vi "Position_TOTAL_R16.vi"(5 "Distance Between \nCameras  (*unit)":sgl=2.1) -> (0 "Valid Beacon Sets":bool[](array[boolean])=[FALSE, TRUE, TRUE, TRUE, FALSE], 12 "dX, dY\nLeft Cam":cluster{"X":sgl[], "Y":sgl[]}={"X"=[0.0, 0.30756128, 1.4106799, 2.4344175, 0.0], "Y"=[0.0, 5.248752, 5.2487316, 5.2487082, 0.0]}, 13 "Position Valid":bool=TRUE, 14 "Left Camera Real Coordinates":cluster{"X":sgl, "Y":sgl}={"X"=5.2487307, "Y"=1.1157805}, 16 "dX, dY\nRight Cam":cluster{"X":sgl[], "Y":sgl[]}={"X"=[-2.0986407, -1.7910794, -0.6879608, 0.3357769, -2.0986407], "Y"=[-0.07554352, 5.1732087, 5.1731877, 5.173165, -0.07554352]}, 17 "Distance to Each Beacon":cluster{" Right Cam":sgl[], " Left Cam":sgl[]}={" Right Cam"=[1.0, 5.491617, 5.181491, 5.20346, 1.0], " Left Cam"=[1.0, 5.2758446, 5.3987226, 5.8034377, 1.0]}, 18 "Robot Coordinates":cluster{"X":sgl, "Y":sgl}={"X"=5.210959, "Y"=2.1651008}, 19 "Orietnation\n(current)":sgl=-2.0627356 format="%#_13g")   [LabVIEW 2015]
uses:
  <vilib>/Analysis/NI_AALPro.lvlib
  <vilib>/myRIO/Instrument Drivers/Onboard IO/DIO/DIO.lvlib
  <vilib>/Instr/_visa.llb/VISA Configure Serial Port (Instr).vi
  <vilib>/Analysis/coordinate.llb/2D Cartesian Coordinate Rotation (Array).vi
panel:
  out "Current Recovery State -L":enum16{"Generic Sweep", "Recovery Search"}(ring)=enum."Recovery Search"
  out "Current Move Delta - L 2":u16
  out "Next Recovery State - Left":enum16{"Generic Sweep", "Recovery Search"}(ring)=enum."Recovery Search"
  out "Next Recovery State - Right":enum16{"Generic Sweep", "Recovery Search"}(ring)=enum."Recovery Search"
  out "Current Recovery State - Right":enum16{"Generic Sweep", "Recovery Search"}(ring)=enum."Recovery Search"
  in  "Initial Recovery State  - Right":enum16{"Generic Sweep", "Recovery Search"}(ring)=enum."Recovery Search"
  in  "Initial Recovery State - L":enum16{"Generic Sweep", "Recovery Search"}(ring)=enum."Recovery Search"
  out "Next Tracking State - Right":enum16{"Track", "Reactive Predict", ""}(ring)
  out "Current Tracking State - Right 2":enum16{"Track", "Reactive Predict", ""}(ring)
  in  "Initial Tracking State - Right":enum16{"Track", "Reactive Predict", ""}(ring)
  out "Last Track Angle - R":sgl=95.68359
  out "Next Tracking State - Left":enum16{"Track", "Reactive Predict", ""}(ring)
  in  "Initial Tracking State - Left":enum16{"Track", "Reactive Predict", ""}(ring)
  out "Current Tracking State - Left":enum16{"Track", "Reactive Predict", ""}(ring)
  in  "Timeout to \nEnable Reactive Predict":u16=10
  out "Tracking Timeout\nCount - R":i32
  in  "Tracking Timeout\nThreshold":i32=10
  out "Tracking Timeout\nCount - L":i32
  in  "Search Direction - in - Right":bool=TRUE
  out "Next Main State - Right":T1(ring)=enum."Tracking"
  in  "Recovery Search\nDirection - R":bool
  out "Recovery Mode Count in Right":i32
  out "Wait Tick Count - Right":i32
  out "Frames Processed\nCount - in Right":i32
  out "Recovery Search\nmove Count - Right":u16
  out "Recovery Search\nAttempt Count - Right":u16
  in  "Mounting Offset - Right":sgl=45.0
  in  "Tracking Angle - Right":sgl=95.568306
  in  "Current Servo Position\n- Right":u16
  out "New Data  Flag\nRight Servo":bool
  in  "Track Angle Valid  - R":bool=TRUE
  out "Current Main State - Right":T1(ring)=enum."Tracking"
  in  "Initial Main State- Right":T1(ring)
  in  "Recovery Search\nDirection - L 2":bool
  in  "Max Recovery Count\n(Recovery Search) 2":u16
  in  "Max Recovery\nSearch Attempts 2":u16
  in  "Image Lock - Right 2":bool
  out "Last Track Angle - L":sgl=73.76953
  in  "Recovery Search\nDirection - L":bool=TRUE
  out "Next Main State - Left":T1(ring)=enum."Tracking"
  out "Current Move Delta - L":u16
  in  "Max Recovery Count\n(Recovery Search)":u16=10
  in  "Max Recovery\nSearch Attempts":u16=3
  out "Recovery Search\nAttempt Count - in - L":u16
  out "Recovery Search\nmove Count - in - L":u16
  in  "Image Lock - Right":bool=TRUE
  out "Recovery Mode Count - in Left":u16
  in  "Middle Beacon\nCoordinates":cluster{"X":sgl, "Y":sgl}={"X"=0.0, "Y"=2.5}
  in  "Min Num Frames\nper Search":i32=3
  in  "Wait Tick Threshold":i32=10
  out "Wait Tick Count - in - L":i32
  out "Frames Processed\nCount - in -L":i32
  in  "Maximum Move \nServo Threshold":i16=300
  in  "Minimum Delta \nServo Threshold":i16=3
  in  "Mounting Offset - Left":sgl=-45.0
  in  "Search Step Size":u16=50
  in  "Search Direction - in - L":bool
  in  "Current Servo Position\n- Left":u16
  in  "Tracking Angle - Left":sgl=72.73481
  out "New Data  Flag\nLeft Servo":bool
  in  "Track Angle Valid - Left":bool=TRUE
  in  "Image Lock - Left":bool=TRUE
  in  "Initial Main State - Left":T1(ring)
  out "Current Main State - Left":T1(ring)=enum."Tracking"
  in  "Position Calc\nTimer":u32=100 caption="Position Calc Timer"
  in  "Fetch Input\n(mSec)":u32=20 caption="Update Camera Input\n(mSec)"
  out "Right Data\nInput Flag\n- Internal":bool
  in  "Position Calc\nReady":bool
  out "This Servo \nAngle - Right":sgl=95.09766
  in  "Beacon Angles -R":sgl[](array[numeric])=[117.22456, 106.97358, 95.568306, 84.2386, 100.09766]
  in  "Beacon Angles - L":sgl[](array[numeric])=[77.890625, 77.890625, 72.73481, 63.190956, 54.217514]
  in  "Valid Angles -R":bool[](array[boolean])=[TRUE, TRUE, TRUE, TRUE, FALSE]
  in  "Valid Angles - L":bool[](array[boolean])=[FALSE, FALSE, TRUE, TRUE, TRUE]
  out "Left Data\nInput Flag\n- Internal":bool=TRUE
  in  "Check Shared Var Timer":u32=50 caption="Main Loop\n Timer (ms)"
  out "Left_Flag 2":bool
  out "Right_Flag 2":bool
  out "Beacons Found\n- Left (Bool Array) 2":bool[](array[boolean])=[FALSE, FALSE, TRUE, TRUE, TRUE]
  out "LEFT Beacon Coord - X px (IN) 2":sgl[](array[numeric])=[0.0, 0.0, 159.73276, 214.00955, 263.49582]
  out "LEFT Beacon Position - Y px (IN) 2":sgl[](array[numeric])=[0.0, 0.0, 153.01732, 149.7353, 148.18039]
  out "This Servo \nAngle - Left":sgl=72.890625
  in  "Compliance Slope":u8=128
  out "deltaMoveServo\n- R":i16
  out "Move Respond - R":bool
  out "Move Respond - L":bool
  out "Last Position":cluster{"X":sgl, "Y":sgl}={"X"=5.210741, "Y"=2.1662946}
  out "Last Orientation":sgl=-2.061552
  in  "Distance\nBetween Beacons \n- Tolerance":sgl=0.35 format="%#_13g"
  in  "Distance\nBetween Beacons":sgl=1.0 format="%#_13g"
  out "atan2(y,x)":sgl=-2.481407
  out "dT":dbl=106.005
  in  "Orientation (-2) \nWeight":sgl=0.083333336 format="%#_13g"
  in  "Orientation (-1) \nWeight":sgl=0.16666667 format="%#_13g"
  in  "New Orientation \nThreshold":sgl=10.0
  out "Position Valid\nHistory":bool[](array[boolean])=[TRUE, FALSE, TRUE, TRUE, FALSE, TRUE, TRUE, FALSE, FALSE, FALSE, FALSE, FALSE, FALSE, FALSE, FALSE]
  out "Orientation\nHistory":sgl[](array[numeric])=[-2.061552, 0.0, -2.0449653, -2.0840735, 0.0, -2.086157, -2.0841389, 0.0, 0.0, 0.0, 0.0, 0.0, 0.0, 0.0, 0.0]
  out "Robot Coordinates\nHistory":cluster{sgl, sgl}[](array[cluster])=[{5.210741, 2.1662946}, {0.0, 0.0}, {5.209907, 2.1666946}, {5.2114477, 2.168679}, {0.0, 0.0}, {5.2056046, 2.1693063}, {5.2068563, 2.1687796}, {0.0, 0.0}, {0.0, 0.0}, {0.0, 0.0}, {0.0, 0.0}, {0.0, 0.0}, {0.0, 0.0}, {0.0, 0.0}, {0.0, 0.0}]
  in  "New Position \nThreshold":sgl=0.2
  in  "position(-2) weight":sgl=0.2 format="%#_13g"
  in  "position(-1) weight":sgl=0.3 format="%#_13g"
  out "Orientation Avgd":sgl=-2.061552
  in  "History Size":u8=15
  in  "Max Y (arena)":sgl=15.0
  in  "Max X (arena)":sgl=35.0
  in  "New Position\nWeight":sgl=0.5 format="%#_13g"
  in  "New Orientation\nWeight":sgl=0.75 format="%#_13g"
  in  "Max Std Dev (3)":sgl=0.2 format="%#_13g"
  in  "Max Std Dev (4)":sgl=0.2 format="%#_13g"
  out "Post Filtering\n- Valid Beacons":bool[](array[boolean])=[FALSE, TRUE, TRUE, TRUE, FALSE]
  in  "New Pos\nThreshold (*unit)\nfilterd UNUSED":sgl=0.2
  out "Robot Coordinates - Avgd":cluster{"X":sgl, "Y":sgl}={"X"=5.210741, "Y"=2.1662946}
  out "Real Position in Course 2":cluster{"X":dbl[], "Y":dbl[]}(graph)={"X"=[5.210741279561325], "Y"=[2.1662946728829504]}
  out "Position \nLock Status":bool=TRUE
  out "Right Camera Real Coordinate":cluster{"X":sgl, "Y":sgl}={"X"=5.1731873, "Y"=3.214421}
  out "deltaMoveServo\n- L":i16
  in  "Search Step Size\n(deg)":sgl=15.0 format="%#_13g"
  out "Beacons Found\n- Right (Bool Array)":bool[](array[boolean])=[TRUE, TRUE, TRUE, TRUE, FALSE]
  out "RIGHT Beacon Position - Y px (IN)":sgl[](array[numeric])=[160.86406, 153.76714, 154.61392, 152.4888, 0.0]
  out "RIGHT Beacon Coord - X px (IN)":sgl[](array[numeric])=[38.476494, 94.79557, 157.79951, 220.26955, 0.0]
  in  "Right Servo\nID":string="\u0001"
  in  "Servo Comm\nWait Time - (ms)":i32=1
  in  "Left Servo\nID":string="\u0000"
  out "dT - Comm Loop":u32=18
  in  "Servo Comm\nLoop Time (ms)":i32=10
  in  "close comms":bool
  in  "Max Read\nTx Attempts":u8=3
  in  "Max Write\nTx Attempts":u8=3
  out "Current R (10bit)":u16=683
  out "Servo Moving - R":bool
  out "Servo Moving - L":bool
  out "Current L (10bit)":u16=300
  in  "SERVO ENABLE":bool=TRUE
  out "Move Servo - L":bool
  out "Move Servo - R":bool
  in  "Servo Goal Position\n - Right":u16=685
  in  "Move Servo\nThreshold (deg)":sgl=2.0 format="%#_13g"
  in  "Servo Algorithm\nCycle Time(ms)":i32=50
  in  "Servo Goal Position\n - Left":u16=300
  in  "Current Angle\n - Left (internal)":sgl=72.890625
  in  "Current Angle\n - Right (internal)":sgl=95.09766
  in  "stop":bool
  in  "Num of Beacons (Total)":i8=5
  out "Angle to Pixel Ratios":T2={"Angle to Pixel\nRatio - Horizontal"=0.18125, "Angle to Pixel\nRatio - Vertical"=0.1875} {"Angle to Pixel\nRatio - Vertical" format="%#_13g"; "Angle to Pixel\nRatio - Horizontal" format="%#_13g"}
  in  "Cam AOV Vertical (deg)":sgl=45.0
  in  "Cam AOV Horizontal (deg)":sgl=58.0
  in  "Image Height (px)":sgl=240.0
  in  "Image Width (px)":sgl=320.0
  out "Beacon Coordinates - Left Image":T3={"Beacon Position - X px"=[0.0, 0.0, 159.73276, 214.00955, 263.49582], "Beacon Position - Y px"=[0.0, 0.0, 153.01732, 149.7353, 148.18039]}
  out "Beacon Coordinates - Right Image":T3={"Beacon Position - X px"=[38.476494, 94.79557, 157.79951, 220.26955, 0.0], "Beacon Position - Y px"=[160.86406, 153.76714, 154.61392, 152.4888, 0.0]}
  out "Distance to LBF":sgl[](array[numeric])=[0.024284193, 0.015691843, 0.008273765, 0.028971607, 0.03291407]
  out "Local Coordinates - Calculated":cluster{sgl[], sgl[]}(graph)={[0.0, 0.49682832, 1.5972277, 2.6223545, 0.0], [0.0, 5.2523994, 5.1570406, 5.1771755, 0.0]}
  out "Local Coordinates - Adjusted":cluster{sgl[], sgl[]}(graph)={[0.0, 0.49617612, 1.59858, 2.6216543, 0.0], [0.0, 5.234291, 5.1945877, 5.1577377, 0.0]}
  out "Normalized Beacons\nCoordinates Relative\nto Robot\n- Local":cluster{"X":sgl[], "Y":sgl[]}={"X"=[0.0, 0.49617612, 1.59858, 2.6216543, 0.0], "Y"=[0.0, 5.234291, 5.1945877, 5.1577377, 0.0]}
  out "Local Coordinates - Rotated":cluster{dbl[], dbl[]}(graph)={[2.0986406972551275, 0.0, 0.30756127015511747, 1.410679881134365, 2.4344175822405747, 0.0], [0.07554351912182478, 0.0, 5.248752221809901, 5.248731441918036, 5.24870847628271, 0.0]}
  out "All Object Coordinates \n- Local - Rotated":cluster{"X":sgl[], "Y":sgl[]}={"X"=[2.0986407, 0.0, 0.30756128, 1.4106799, 2.4344175, 0.0], "Y"=[0.07554352, 0.0, 5.248752, 5.2487316, 5.2487082, 0.0]}
  out "Local Coordinates - Normalized":cluster{sgl[], dbl[]}(graph)={[2.1, 0.0, 0.49617612, 1.59858, 2.6216543, 0.0], [0.0, 0.0, 5.234291076660156, 5.194587707519531, 5.157737731933594, 0.0]}
  in  "Max Std Dev (5)":sgl=0.2 format="%#_13g"
  out "All Object Coordinates \n- Local":cluster{"X":sgl[], "Y":sgl[]}={"X"=[2.1, 0.0, 0.49617612, 1.59858, 2.6216543, 0.0], "Y"=[0.0, 0.0, 5.234291, 5.1945877, 5.1577377, 0.0]}
  out "LOCAL\nBeacon Coordinates\nRelative to Robot":cluster{"dX_beacon":sgl[], "dY_beacon":sgl[]}={"dX_beacon"=[0.0, 0.49682832, 1.5972277, 2.6223545, 0.0], "dY_beacon"=[0.0, 5.2523994, 5.1570406, 5.1771755, 0.0]}
  out "dA2":sgl=26.863228 format="%#_13g"
  out "All Same\nDirection":bool=TRUE
  out "Valid Data\nSets":bool[](array[boolean])=[FALSE, TRUE, TRUE, TRUE, FALSE]
  in  "Distance Threshold\nRef Triangles (*unit)":sgl=20.0
  in  "Real Beacon\n - Coordinates":cluster{"X":dbl[], "Y":dbl[]}={"X"=[0.0, 0.0, 0.0, 0.0, 0.0, 0.0], "Y"=[0.5, 1.5, 2.5, 3.5, 4.5, 0.0]}
  # "POSITION CALCULATION VARIABLES"
  # "OUTPUT VALUES"
  # "CONFIG VALUES"
  # "FILTER CONFIG VALUES"
  # "FEEDBACK INPUT VALUES"
  # "INPUT VALUES"
  # "INTERMEDIATE VALUES"
  # "IMAGE TO ANGLE VARIABLES"
  # "VISION PROCESSEING INPUTS"
  # "Use moving average for previous orientation thresholds"
  # "INPUTS"
  # "CONFIG"
  # "OUTPUT VALUES"
  # "*********************"
  # "unfiltered"
  # "NEW FILTER VALS"
  # "Inter Beacon Distance Filtering"
  # "SERVO CONTROL VARIABLES"
  # "SERVO CONTROL VARIABLES"
  # "CONFIG"
  # "SHARED VARIABLE INPUTS"
  # "LOCAL VARIABLE INPUTS"
  # "INTERNRAL VARIABLES"
  # "SEARCH ROUTINE VARIABLES"
  # "MISC"
  # "SERVO IDs"
  # "CONTROL DELAYS"
  # "COMM LOOP DELAY"
  # "COMM PROTOCOL"
  # "SETTINGS"
  # "Make function of distance^^"
  # "**** only left side starts search\nat previously known good angle"
  # "LEFT SERVO"
  # "RIGHT SERVO"
  # "Main State Machine"
  # "Recovery State Machine"
  # "Current Track Angle Inputs"
  # "Servo Status Inputs"
  # "Main State Machine Inputs"
  # "Recovery State Machine Inputs"
  # "Current Track Angle Inputs"
  # "Servo Status Inputs"
  # "Recovery State Machine Feedback"
  # "Tracking State Machine Inputs"
  # "Tracking State Machine Inputs"
  # "NOTE: Must be 1 bigger than amount of beacons"
  # "NOTE: Must be 1 bigger than amount of beacons"
types:
  T1 = enum16{"Start Up Search", "Tracking", "Recovery Mode", ""}
  T2 = cluster{"Angle to Pixel\nRatio - Horizontal":sgl, "Angle to Pixel\nRatio - Vertical":sgl}
  T3 = cluster{"Beacon Position - X px":sgl[], "Beacon Position - Y px":sgl[]}
  T4 = cluster{"Array of Double":dbl[], "Array of Double":dbl[]}
  T5 = typedef "DIO.lvlib/DIO Reference.ctl" = cluster{"myRIO Reference":T6, "DIO Channels List":T10}
  T6 = typedef "myRIO Generic Hardware Reference.ctl" = cluster{"myRIO Model":T7, "myRIO Hardware Reference":T8}
  T7 = typedef "Hardware Version Enum.ctl" = enum16{"Unknown", "myRIO-1900", "myRIO-1950", "roboRIO"}
  T8 = typedef "myRIO v1.0 Reference.ctl" = cluster{"Generic FPGA Reference":T9, "Allow multiple opens":bool}
  T9 = typedef "Generic FPGA Reference.ctl" = refnum<k20>
  T10 = typedef "DIO Channels List.ctl" = T11[]
  T11 = typedef "DIO Channels Enum.ctl" = enum16{"Not Connected", "C/DIO0", "C/DIO1", "C/DIO2", "C/DIO3", "C/DIO4", "C/DIO5", "C/DIO6", "C/DIO7", "A/DIO0", "A/DIO1", "A/DIO2", "A/DIO3", "A/DIO4", "A/DIO5", "A/DIO6", "A/DIO7", "A/DIO8", "A/DIO9", "A/DIO10", "A/DIO11", "A/DIO12", "A/DIO13", "A/DIO14", "A/DIO15", "B/DIO0", "B/DIO1", "B/DIO2", "B/DIO3", "B/DIO4", "B/DIO5", "B/DIO6", "B/DIO7", "B/DIO8", "B/DIO9", "B/DIO10", "B/DIO11", "B/DIO12", "B/DIO13", "B/DIO14", "B/DIO15", "LED0", "LED1", "LED2", "LED3", "Button0", "DIO/DIO0", "DIO/DIO1", "DIO/DIO2", "DIO/DIO3", "DIO/DIO4", "DIO/DIO5", "DIO/DIO6", "DIO/DIO7", "DIO/DIO8", "DIO/DIO9", "SPI/CS0", "SPI/CS1", "SPI/CS2", "SPI/CS3", "LED RADIO (Green)", "LED RADIO (Red)", "LED COMM (Green)", "LED COMM (Red)", "LED MODE (Green)", "LED MODE (Red)"}
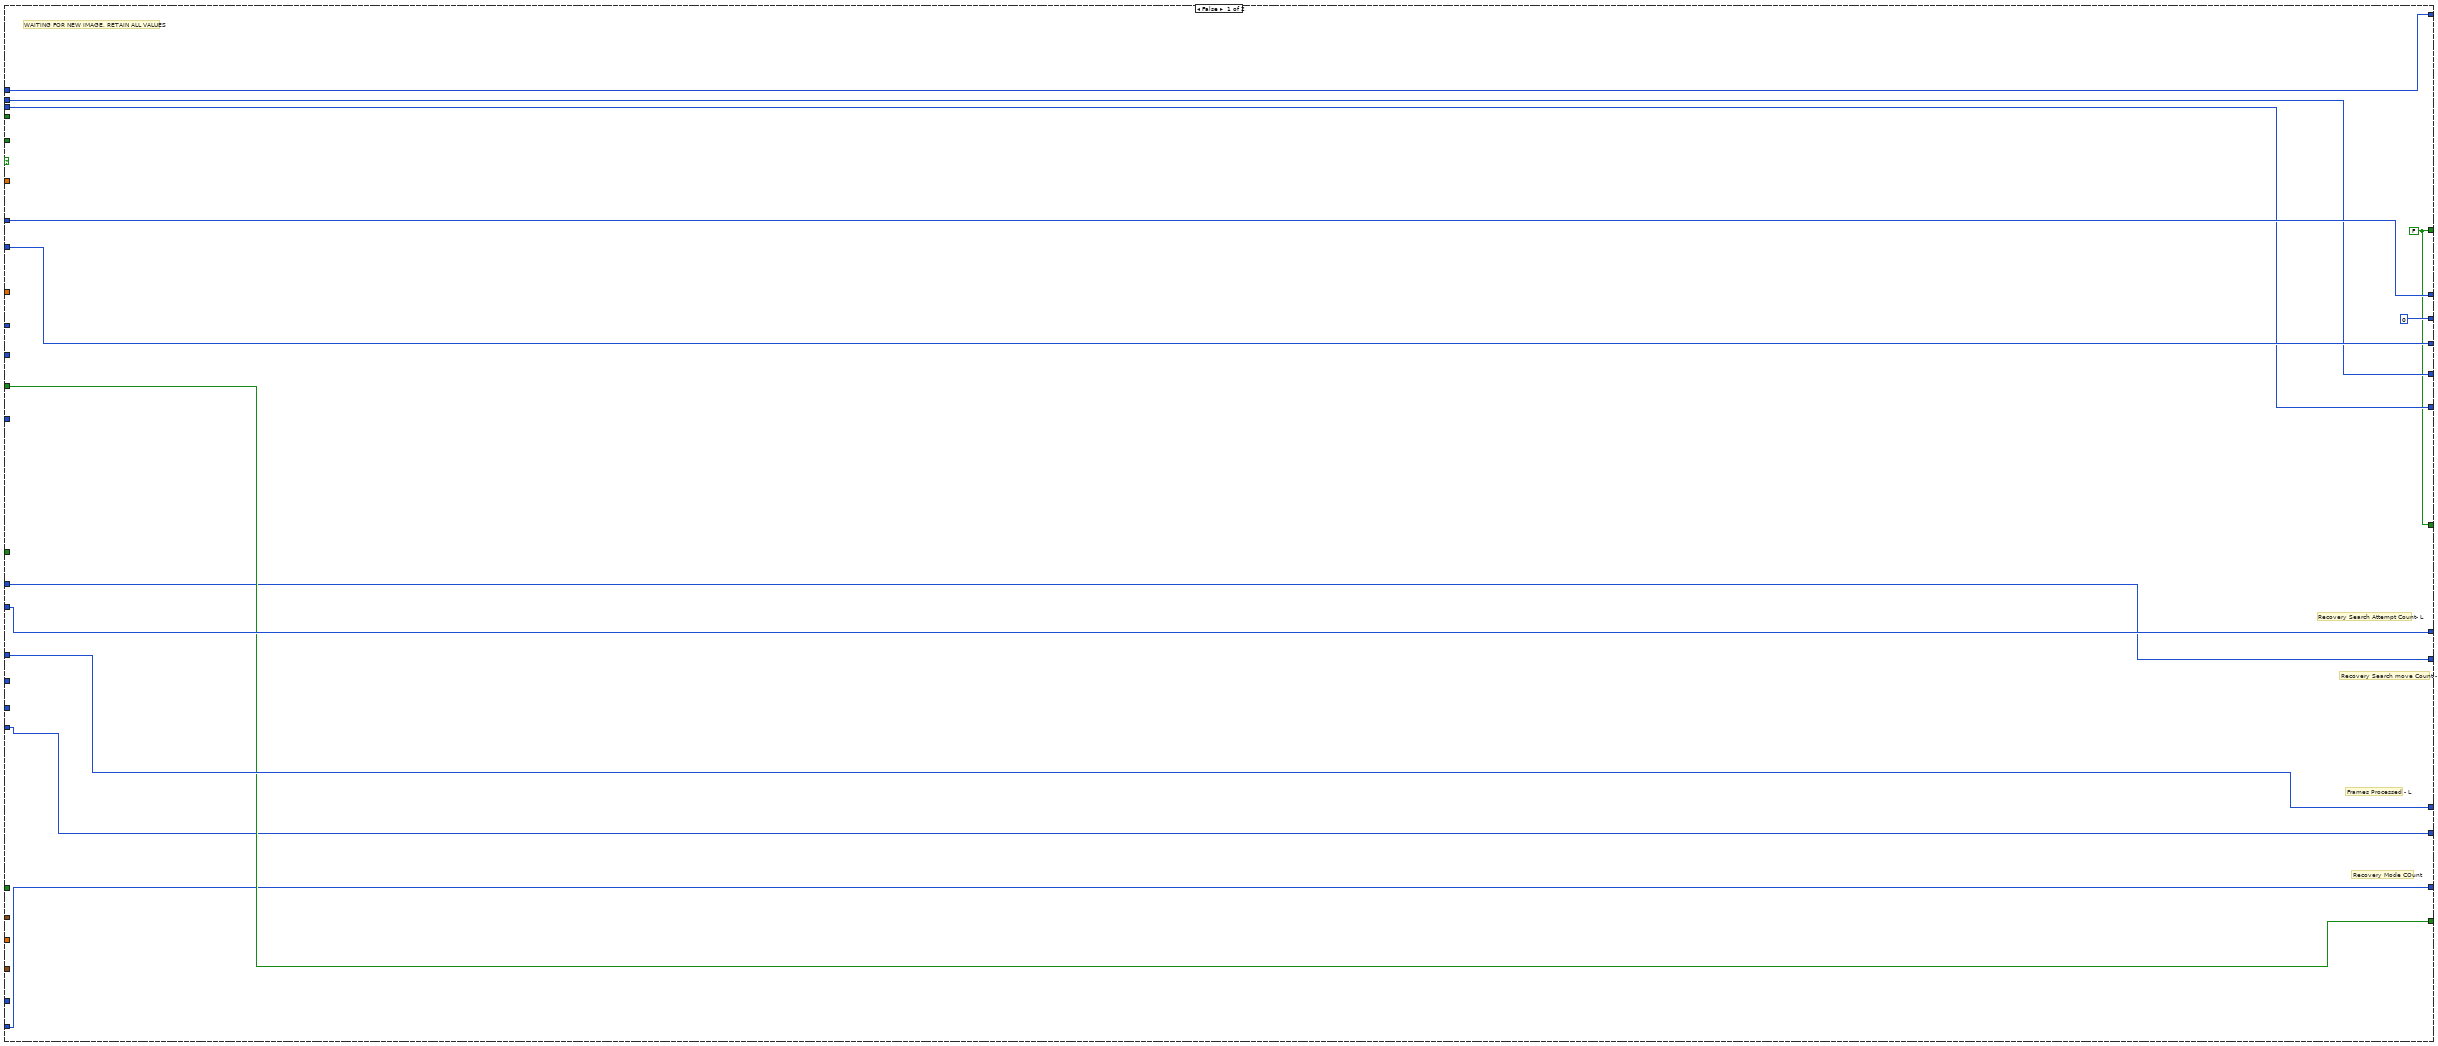
[diagram p2: hidden frame]
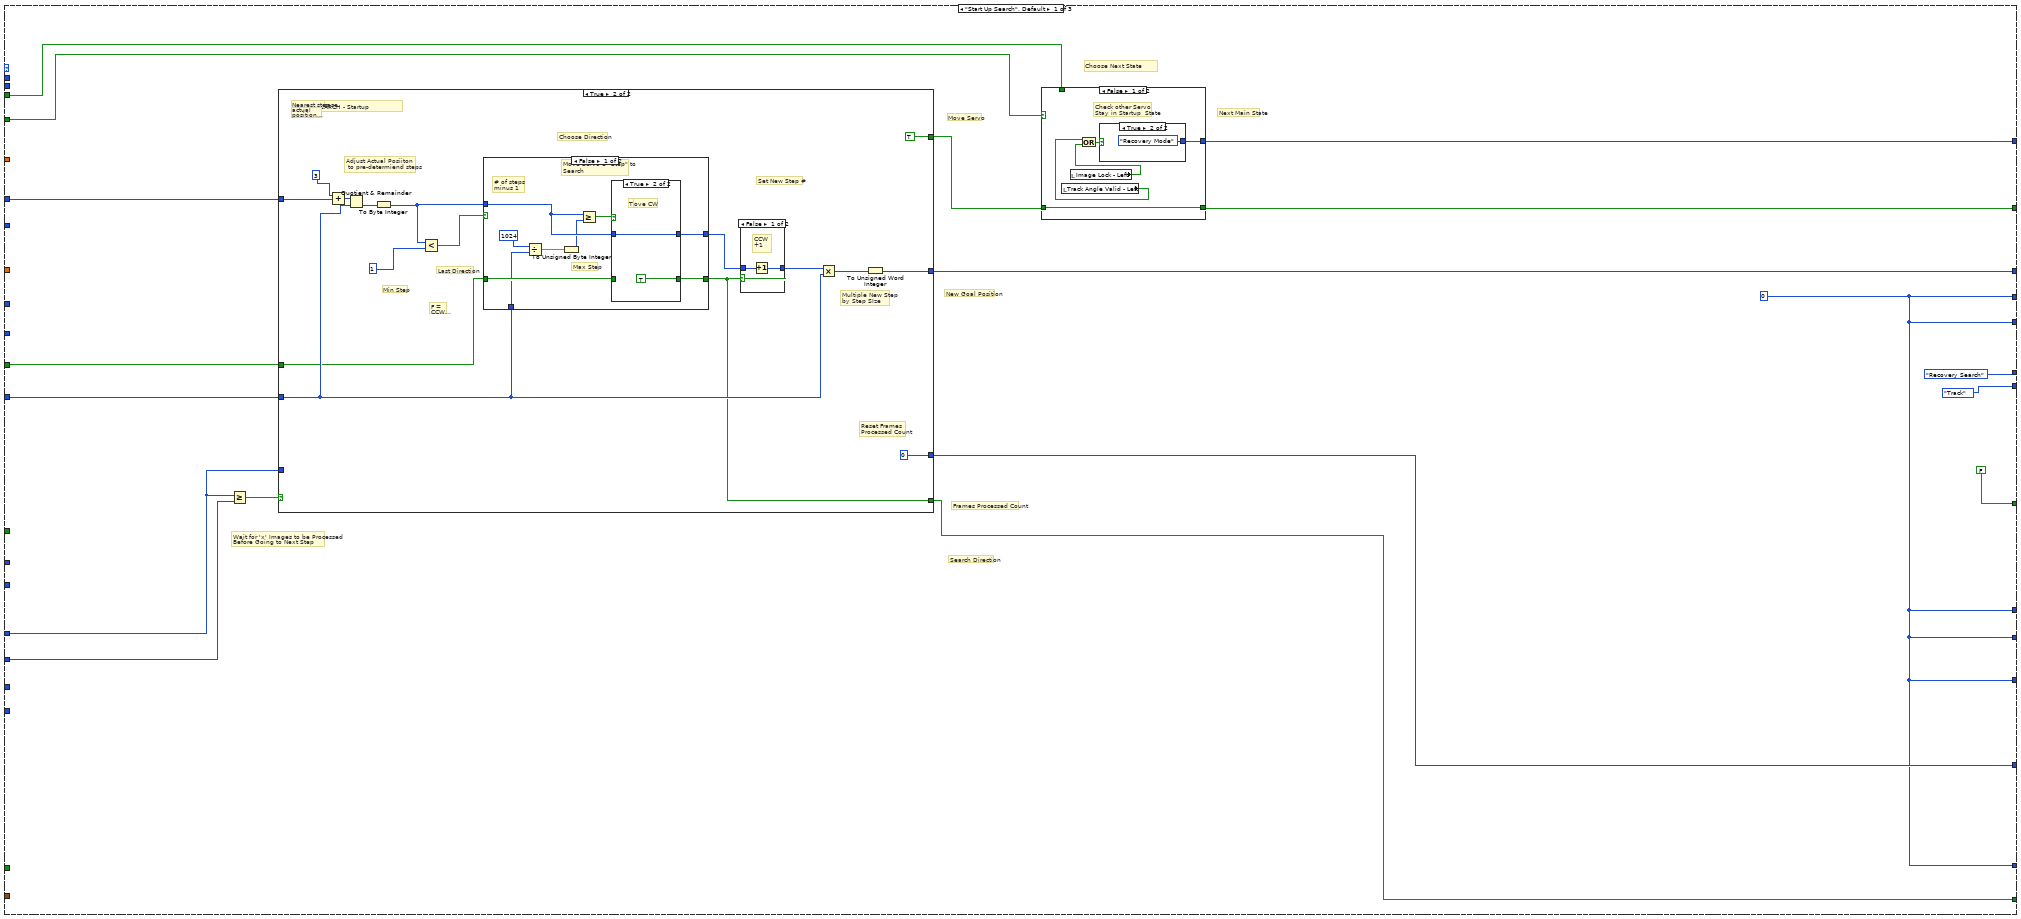
[diagram p3: hidden frame]
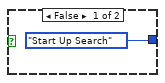
[diagram p4: hidden frame]
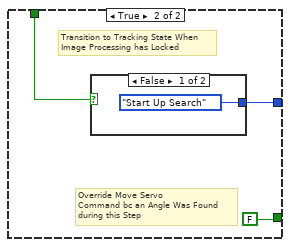
[diagram p5: hidden frame]
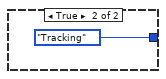
[diagram p6: hidden frame]
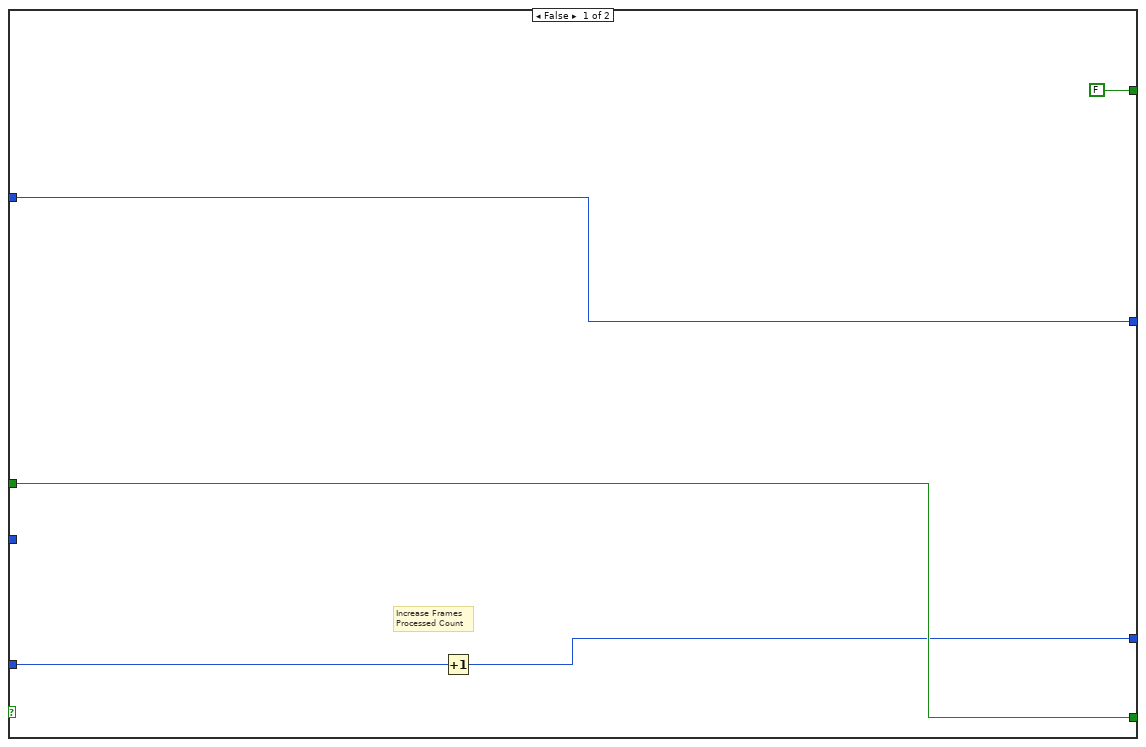
[diagram p7: hidden frame]
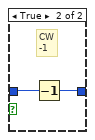
[diagram p8: hidden frame]
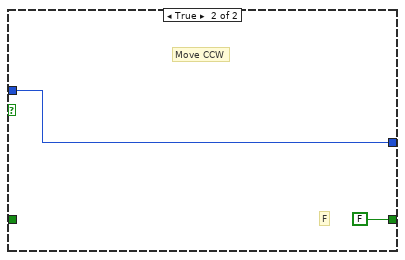
[diagram p10: hidden frame]
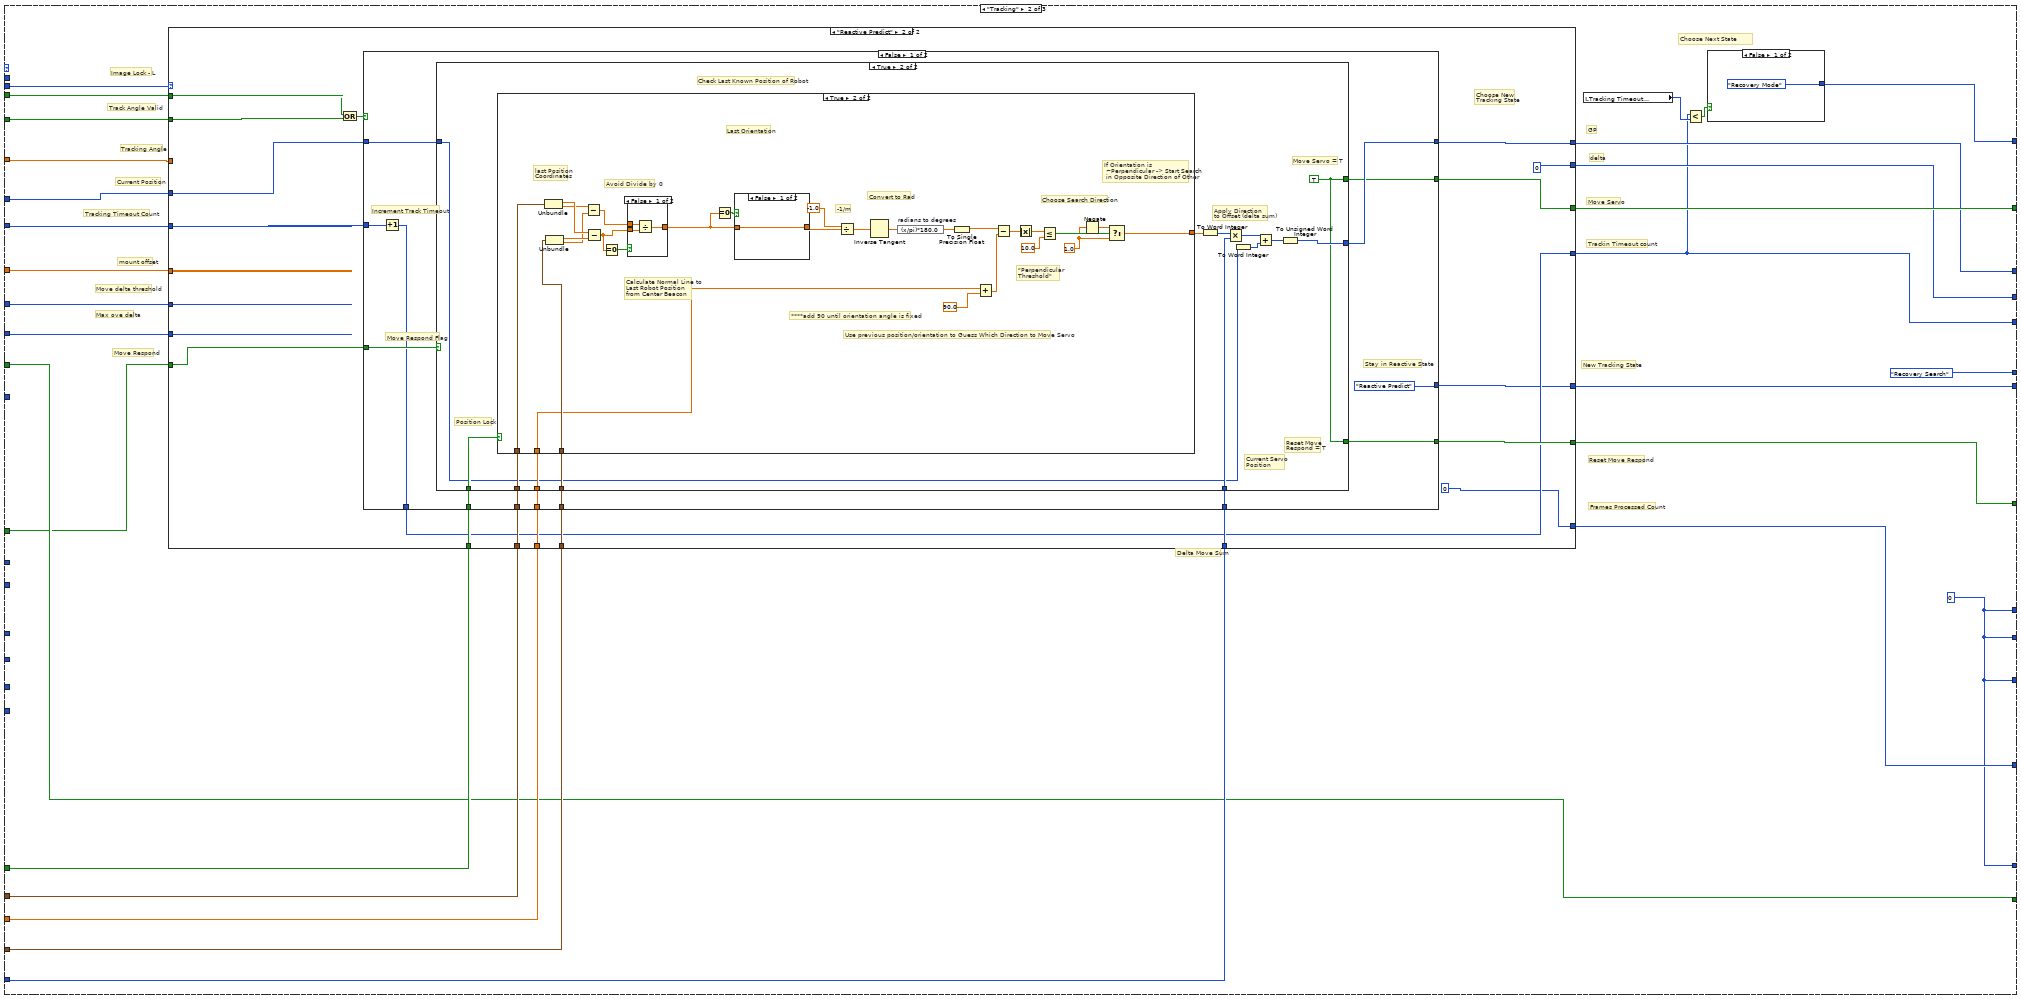
[diagram p11: hidden frame]
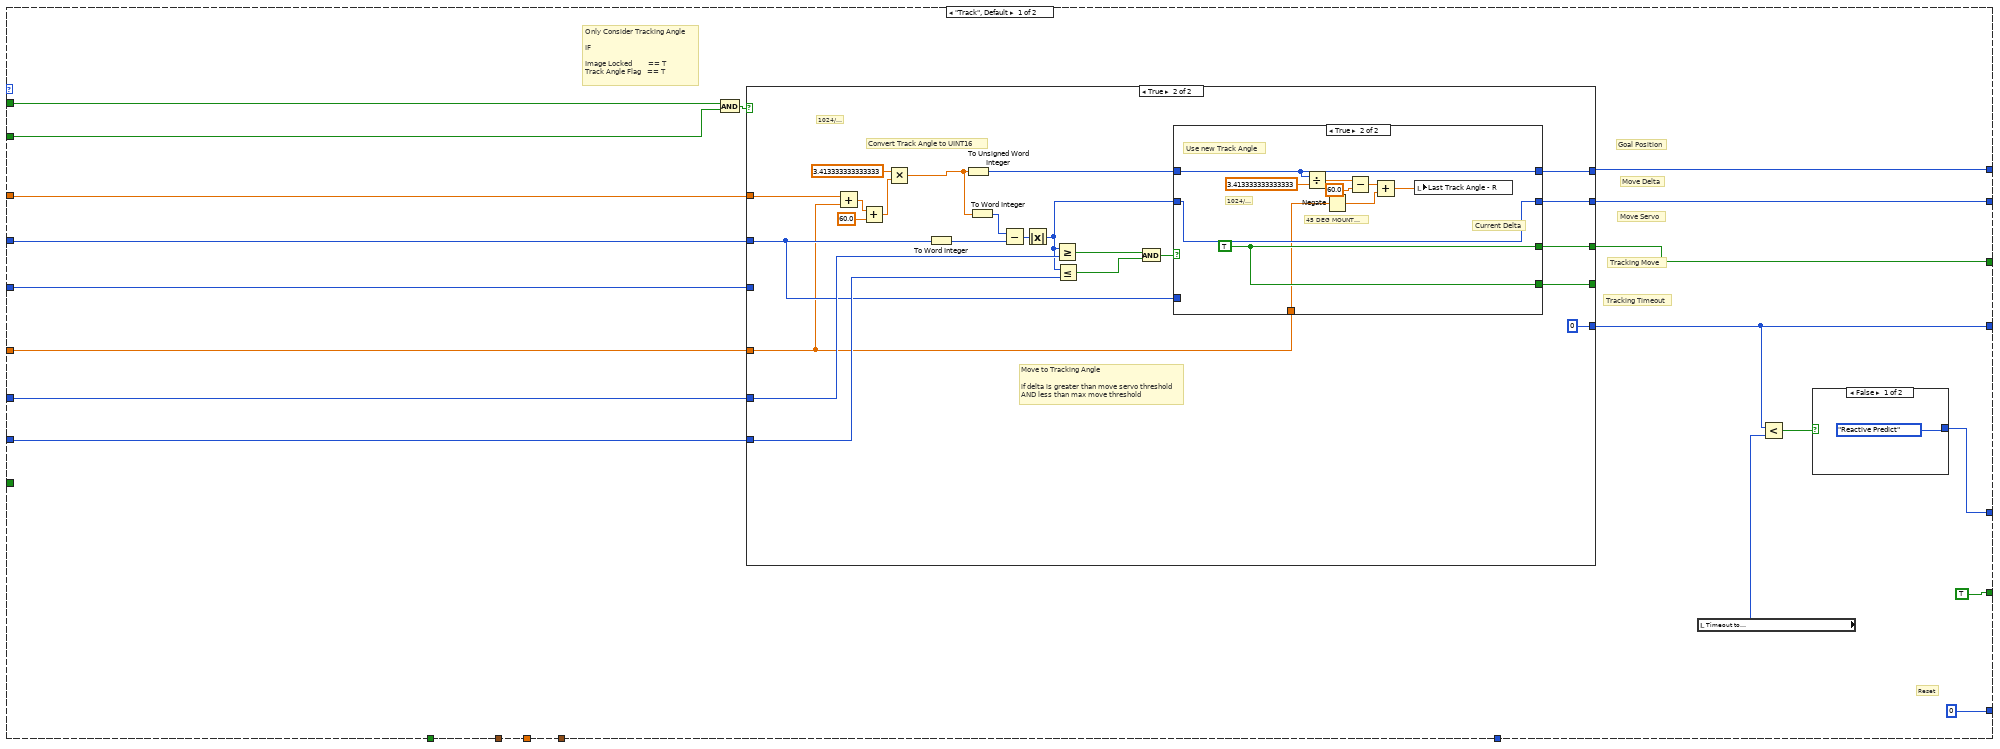
[diagram p12: hidden frame]
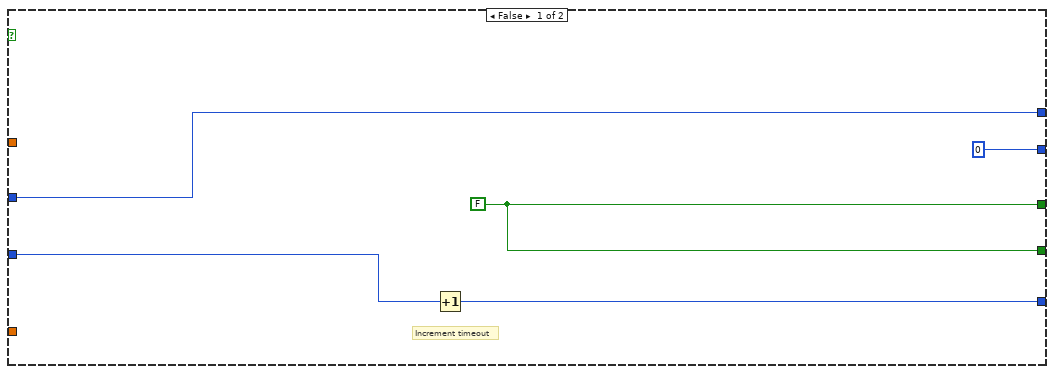
[diagram p13: hidden frame]
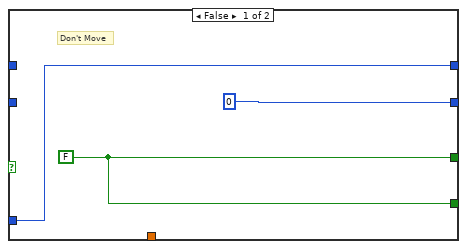
[diagram p14: hidden frame]
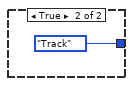
[diagram p15: hidden frame]
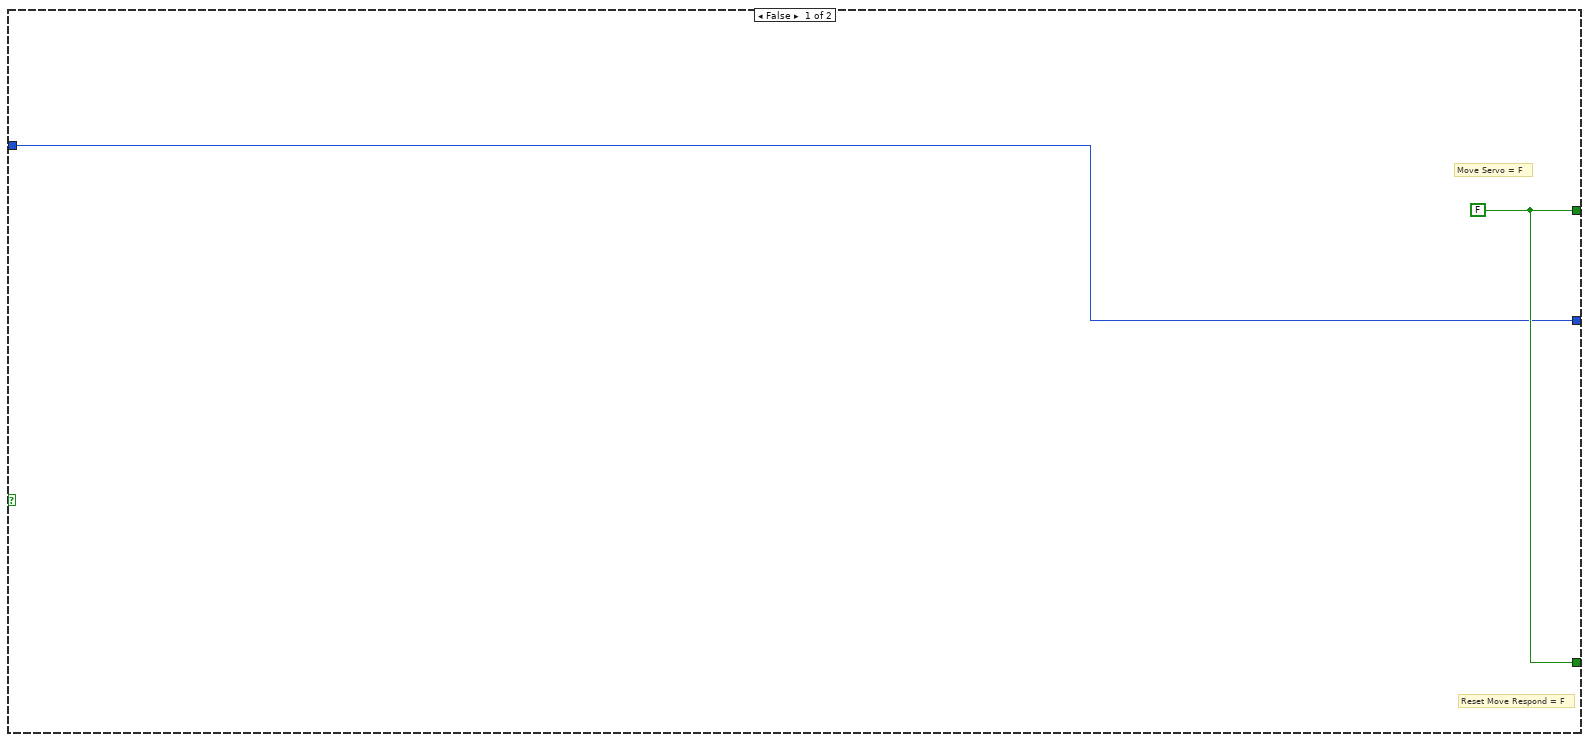
[diagram p16: hidden frame]
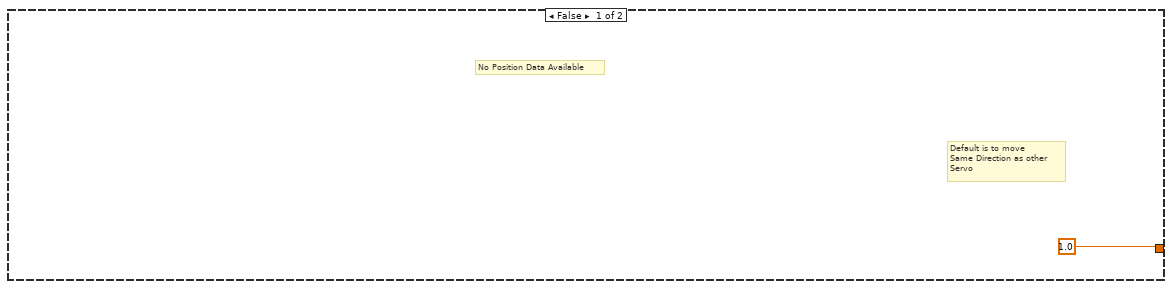
[diagram p17: hidden frame]
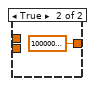
[diagram p18: hidden frame]
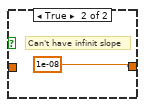
[diagram p19: hidden frame]
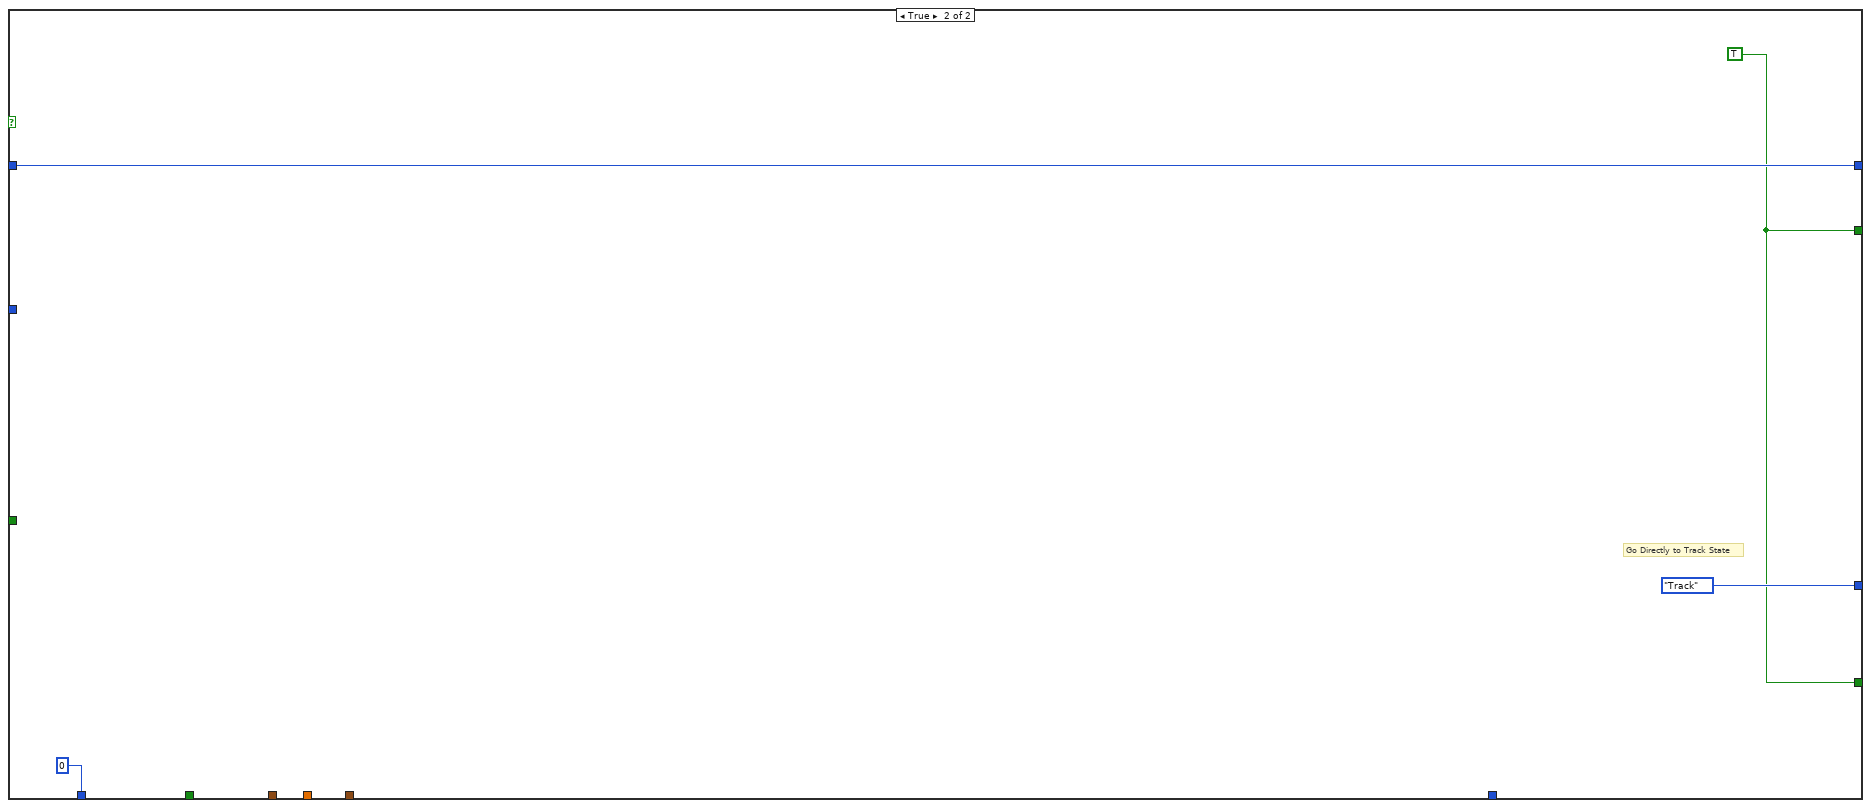
[diagram p20: hidden frame]
diagram:
  (unwired) enum16{"Generic Sweep", "Recovery Search"}."Recovery Search"
  w11 = 0 ("Frames Processed\nCount - in")
  w12 = 0 ("Frames Processed\nCount - in")
  w1 = FALSE
  w34 = sgl 0.0
  # "SERVO CONTROL FLAGS"
  # "***"
  # "Next Tracking State"
  # "Tracking Timeout Count"
  # "Search Direction - L"
  # "Next Recovery State"
  # "Move Respond"
  # "Recovery Mode Count - L"
  # "Delta Move Sum - L"
  # "Wait Tick Count - L"
  # "Frames Processed - L"
  # "Recovery Search move Count - L"
  # "Recovery Search Attempt Count- L"
  # "Next Main State"
  # "Search Direction - L"
  # "Next Recovery State"
  # "INPUTS - Local vars"
  # "Recovery Mode Count - L"
  # "Delta Move Sum - L"
  # "Wait Tick Count \nLeft"
  # "Frames Processed\nLeft"
  # "Move Respond - R"
  # "Initial Search Direction\n- Right"
  # "Move Respond"
  # "Recovery Mode Count - L"
  # "Delta Move Sum - L"
  # "Wait Tick Count - L"
  # "Frames Processed - L"
  # "Recovery Search move Count - L"
  # "Recovery Search Attempt Count- L"
  # "Next Main State"
  # "Settings -- Update in a slow loop"
  # "Recovery Mode Count - L"
  # "Delta Move Sum - L"
  # "Wait Tick Count \nLeft"
  # "Frames Processed\nLeft"
  # "Move Respond - L"
  # "Replace these with\nconstants"
  # "Initial Search Direction\n- Left"
  # "Read Inputs when Available"
  # "# of Physical Beacons"
  # "Right Data Internal Falg"
  # "Left Data Internal Falg"
  # "Initialize Shift Arrays"
  # "Robot Position (cluster)\nShift Array"
  # "Robot Position (cluster)\nShift Array"
  # "Position Valid Shift Array"
  # "Orientation Shift Array"
  # "Position Valid Shift Array"
  # "Orientation Shift Array"
  # "Servo Communication (to Servo- UART))"
  # "Internal Local Variables"
  # "Servo Control Logic"
  # "Local Variables"
  # "Images to Robot Position Calculation Process"
  # "SERVO MOTOR CONTROL"
  # "SERVO MOTOR CONTROL"
  n1 = Divide(x="Cam AOV Horizontal (deg)", y="Image Width (px)") -> (x/y=w25:sgl)
  n2 = Divide(x="Cam AOV Vertical (deg)", y="Image Height (px)") -> (x/y=w26:sgl)
  n3 = Bundle(w25, w26) -> (w20:cluster{sgl, sgl})  [unwired: 1 in]
  "Angle to Pixel Ratios" <- w20
  n4 = disable-structure shown="Disabled" {
    frame Disabled {
      # "Always Read Incoming Flags & Store"
      n5 = while {
        tunnel: "Check Shared Var Timer" -> [w46]
        stop <- FALSE stop-if-true
        n6 = shared-variable "myRIO-1900\\Lib1.lvlib\\RIGHT_FLAG"() -> (→"Right_Flag 2":bool)  [unwired: 1 in, 1 out]
        n7 = shared-variable "myRIO-1900\\Lib1.lvlib\\Left_Flag"() -> (→"Left_Flag 2":bool)  [unwired: 1 in, 1 out]
        n8 = call "Wait8"("Count(mSec)"=w46) -> ()  [unwired: 1 out]
      }
    }
    frame Enabled {
    }
  }
  n9 = while {
    shift-right: [w55] -> _
    shift-left: w1 -> [w60]
    shift-right: [w54] -> _
    shift-left: w1 -> [w58]
    tunnel: w20 -> [w56]
    tunnel: "Num of Beacons (Total)" -> [w57]
    stop <- FALSE stop-if-true
    # "Wait for Both Internal Flags"
    n10 = call "Wait6"("Count(mSec)"="Fetch Input\n(mSec)") -> ()  [unwired: 1 out]
    n11 = shared-variable "RT myRIO Target - Overlord\\Localization_Variables_r0.lvlib\\RIGHT_FLAG"() -> (w51:bool)  [unwired: 1 in, 1 out]
    n12 = shared-variable "RT myRIO Target - Overlord\\Localization_Variables_r0.lvlib\\Left_Flag"() -> (w52:bool)  [unwired: 1 in, 1 out]
    n13 = case shown="True" w51 {
      tunnel: w57 -> [_ w75]
      tunnel: w56 -> [_ w73]
      tunnel: [w61 w62] -> w49
      tunnel: w58 -> [w61 _]
      frame False {
        # "Don't Update Servo Position\nbc we're waiting on new Data to\ncome in and the servo position\nwas set at the previous set of data"
      }
      frame True {
        w62 = TRUE
        # "Store Values"
        # "Raise Internal Flag"
        # "If New Data Available"
        # "From Shift Reg"
        # "Perforrm Indivudual Angle Calculation"
        # "Pull Down Individual Flag"
        n14 = shared-variable "RT myRIO Target - Overlord\\Localization_Variables_r0.lvlib\\RIGHT_BEACON_X_array"() -> (w68:dbl[])  [unwired: 1 in, 1 out]
        "RIGHT Beacon Coord - X px (IN)" <- w68
        n15 = shared-variable "RT myRIO Target - Overlord\\Localization_Variables_r0.lvlib\\Image Lock - R"() -> (w63:bool)  [unwired: 1 in, 1 out]
        n16 = shared-variable "RT myRIO Target - Overlord\\Localization_Variables_r0.lvlib\\RIGHT_BEACON_Y_array"() -> (w67:dbl[])  [unwired: 1 in, 1 out]
        "RIGHT Beacon Position - Y px (IN)" <- w67
        n17 = shared-variable "RT myRIO Target - Overlord\\Localization_Variables_r0.lvlib\\RIGHT_BEACON_BOOL_array"() -> (w66:bool[])  [unwired: 1 in, 1 out]
        "Beacons Found\n- Right (Bool Array)" <- w66
        n18 = local write "Image Lock - Right"(w63) -> ()
        n19 = Bundle("Array of Double"=w68, "Array of Double"=w67) -> (w65:T4)  [unwired: 1 in]
        "Beacon Coordinates - Right Image" <- w65
        n20 = shared-variable "RT myRIO Target - Overlord\\Localization_Variables_r0.lvlib\\Right Servo Angle_Image"() -> (w64:dbl)  [unwired: 1 in, 1 out]
        "This Servo \nAngle - Right" <- w64
        n21 = shared-variable "RT myRIO Target - Overlord\\Localization_Variables_r0.lvlib\\RIGHT_FLAG"(FALSE) -> ()  [unwired: 1 in, 1 out]
        n22 = feedback #1() -> (w77:sgl[])  [unwired: 1 in]
        n23 = feedback #2() -> (w76:bool[])  [unwired: 1 in]
        n24 = call "Angle Calc_Individual Process R2.vi"("Angle to Pixel Ratios"=w73, "Previous Angles"=w77, "Num of Beacons"=w75, "Beacon Coordinates - Image"=w65, "Current Servo Angle"=w64, "Beacons Found (Bool Array)"=w66, "Previous Valid Angles"=w76) -> ("Servo Goal Angle"=w72:dbl, "Valid Beacons (Bool Array)\nPosition Calc"=w70:bool[], "Angle Of Beacons \nRelative to Robot"=w69:sgl[], "Angles Valid\nServo Control"=w71:bool)  [unwired: 2 in, 3 out]
        n25 = feedback-in #1(w69) -> ()
        n26 = feedback-in #2(w70) -> ()
        n27 = local write "Track Angle Valid  - R"(w71) -> ()
        n28 = local write "Beacon Angles -R"(w69) -> ()
        n29 = local write "Valid Angles -R"(w70) -> ()
        n30 = local write "Tracking Angle - Right"(w72) -> ()
        n31 = local write "New Data  Flag\nRight Servo"(w62) -> ()
      }
    }
    "Right Data\nInput Flag\n- Internal" <- w49
    n32 = case shown="True" w52 {
      tunnel: [w78 w79] -> w48
      tunnel: w60 -> [w78 _]
      tunnel: w56 -> [_ w83]
      tunnel: w57 -> [_ w82]
      frame False {
        # "Don't Update Servo Position\nbc we're waiting on new Data to\ncome in and the servo position\nwas set at the previous set of data"
      }
      frame True {
        w79 = TRUE
        # "Store Values"
        # "Raise Internal Flag"
        # "If New Data Available"
        # "Perforrm Indivudual Angle Calculation"
        # "Pull Down Individual Flag"
        n33 = shared-variable "RT myRIO Target - Overlord\\Localization_Variables_r0.lvlib\\LEFT_BEACON_X_array"() -> (w90:dbl[])  [unwired: 1 in, 1 out]
        "LEFT Beacon Coord - X px (IN) 2" <- w90
        n34 = shared-variable "RT myRIO Target - Overlord\\Localization_Variables_r0.lvlib\\LEFT_BEACON_Y_array"() -> (w91:dbl[])  [unwired: 1 in, 1 out]
        "LEFT Beacon Position - Y px (IN) 2" <- w91
        n35 = shared-variable "RT myRIO Target - Overlord\\Localization_Variables_r0.lvlib\\LEFT_BEACON_BOOL_array"() -> (w92:bool[])  [unwired: 1 in, 1 out]
        "Beacons Found\n- Left (Bool Array) 2" <- w92
        n36 = shared-variable "RT myRIO Target - Overlord\\Localization_Variables_r0.lvlib\\Image Lock - L"() -> (w80:bool)  [unwired: 1 in, 1 out]
        n37 = local write "Image Lock - Left"(w80) -> ()
        n38 = Bundle("Array of Double"=w90, "Array of Double"=w91) -> (w88:T4)  [unwired: 1 in]
        "Beacon Coordinates - Left Image" <- w88
        n39 = shared-variable "RT myRIO Target - Overlord\\Localization_Variables_r0.lvlib\\Left Servo Angle_Image"() -> (w81:dbl)  [unwired: 1 in, 1 out]
        "This Servo \nAngle - Left" <- w81
        n40 = shared-variable "RT myRIO Target - Overlord\\Localization_Variables_r0.lvlib\\Left_Flag"(FALSE) -> ()  [unwired: 1 in, 1 out]
        n41 = feedback #3() -> (w94:sgl[])  [unwired: 1 in]
        n42 = feedback #4() -> (w93:bool[])  [unwired: 1 in]
        n43 = call "Angle Calc_Individual Process R2.vi"("Angle to Pixel Ratios"=w83, "Previous Angles"=w94, "Num of Beacons"=w82, "Beacon Coordinates - Image"=w88, "Current Servo Angle"=w81, "Beacons Found (Bool Array)"=w92, "Previous Valid Angles"=w93) -> ("Servo Goal Angle"=w87:dbl, "Valid Beacons (Bool Array)\nPosition Calc"=w85:bool[], "Angle Of Beacons \nRelative to Robot"=w84:sgl[], "Angles Valid\nServo Control"=w86:bool)  [unwired: 2 in, 3 out]
        n44 = feedback-in #3(w84) -> ()
        n45 = feedback-in #4(w85) -> ()
        n46 = local write "Track Angle Valid - Left"(w86) -> ()
        n47 = local write "Beacon Angles - L"(w84) -> ()
        n48 = local write "Valid Angles - L"(w85) -> ()
        n49 = local write "Tracking Angle - Left"(w87) -> ()
        n50 = local write "New Data  Flag\nLeft Servo"(w79) -> ()
      }
    }
    "Left Data\nInput Flag\n- Internal" <- w48
    n51 = And(x=w48, y=w49) -> (x .and. y?=w59:bool)
    n52 = case shown="True" w59 {
      selector: w59 -> [_ w97]
      tunnel: w48 -> [w96 _]
      tunnel: [w96 w98] -> w55
      tunnel: [w95 w98] -> w54
      tunnel: w49 -> [w95 _]
      frame False {
      }
      frame True {
        w98 = FALSE
        # "Reset Internal Data Flags"
        # "Position Data\nReady Enabled"
        n53 = local write "Position Calc\nReady"(w97) -> ()
      }
    }
  }
  n54 = Bundle(w34, w34) -> (w37:cluster{sgl, sgl})  [unwired: 1 in]
  n55 = Initialize Array(w34, "History Size") -> (w32:sgl[])
  n56 = Initialize Array(w37, "History Size") -> (w33:cluster{sgl, sgl}[])
  n57 = Initialize Array(FALSE, "History Size") -> (w31:bool[])
  n58 = call "Tick Count4"() -> ("Tick Count(uSec)"=w30:u32)
  n59 = while {
    shift-right: [w109] -> _
    shift-left: w32 -> [w106]
    shift-right: [w108] -> _
    shift-left: w31 -> [w107]
    shift-right: [w110] -> _
    shift-left: w33 -> [w101]
    shift-right: [w102] -> _
    shift-left: w30 -> [w103]
    stop <- "stop" stop-if-true
    n60 = call "Wait5"("Count(mSec)"="Position Calc\nTimer") -> ()  [unwired: 1 out]
    n61 = case shown="True" "Position Calc\nReady" {
      selector: "Position Calc\nReady" -> [_ w122]
      tunnel: w101 -> [_ w159]
      tunnel: w101 -> [w119 w149]
      tunnel: w106 -> [w121 w148]
      tunnel: w107 -> [w120 w147]
      tunnel: [w121 w146] -> w109
      tunnel: [w120 w141] -> w108
      tunnel: [w119 w145] -> w110
      tunnel: w107 -> [_ w144]
      tunnel: w106 -> [_ w143]
      tunnel: [w118 w134] -> w104
      tunnel: w103 -> [_ w134]
      tunnel: [FALSE TRUE] -> w105
      tunnel: w101 -> [_ w129]
      frame False {
        n62 = call "Tick Count5"() -> ("Tick Count(uSec)"=w118:u32)
      }
      frame True {
        # "Update Outputs\nif Current Calc is Invalid\n(shouldn't matter)"
        # "Estimate Orienation Based on Previous Position"
        # "****# of previous in history that must be true\nin order for position to be considered \"locked\""
        # "New Position is Valid if both \nOrientation and Positions\nis within range of previous"
        # "Robot Position\n Shift Array"
        # "Position Valid Shift Array"
        # "Orientation Shift Array"
        # "Orientation Value"
        # "Shift & Insert Current Position Valid"
        # "Position Valid\n(orientation)"
        # "Position Valid\n(position)"
        # "Update Shift Registers"
        # "Shift & Insert Current Calculated Orientation"
        # "Shift & Insert Current Robot Position"
        # "UPDATE FINAL OUTPUT\n VALUES"
        # "Find Common Beacons\nAmong Cameras"
        # "Valid Beacon Sets"
        # "Currently will only\ncalculate position if 2+ \nbeacons are available \nfrom both cameras"
        n63 = Not(x=w122) -> (.not. x?=w123:bool)
        n64 = local write "Position Calc\nReady"(w123) -> ()
        n65 = disable-structure shown="Disabled" {
          disable-tunnel: "Valid Angles - L" -> [w224 _]
          disable-tunnel: "Valid Angles -R" -> [w223 _]
          frame Disabled {
            # "Each has at \nleast 1 beacon"
            n66 = Boolean Array To Number(Boolean array=w223) -> (number=w225:u32)
            n67 = Boolean Array To Number(Boolean array=w224) -> (number=w226:u32)
            n68 = Greater Than 0?(x=w225) -> (x > 0?=w227:bool)
            n69 = Greater Than 0?(x=w226) -> (x > 0?=w228:bool)
            n70 = And(x=w228, y=w227) -> ()  [unwired: 1 out]
          }
          frame Enabled {
          }
        }
        n71 = And(x="Valid Angles - L", y="Valid Angles -R") -> (x .and. y?=w160:bool[])
        "Valid Beacon Sets" <- w160
        n72 = local read "Num of Beacons (Total)"() -> (w124:i8)
        n73 = Boolean To (0,1)(Boolean=w160) -> (0, 1=w164:i16[])
        n74 = Add Array Elements(numeric array=w164) -> (sum=w163:i16)
        n75 = Greater?(x=w163, y=1) -> (0:w161:bool)
        n76 = case shown="True" w161 {
          tunnel: w160 -> [_ w245]
          tunnel: "Beacon Angles - L" -> [_ w243]
          tunnel: "Beacon Angles -R" -> [_ w242]
          tunnel: w124 -> [_ w244]
          tunnel: w160 -> [_ w240]
          tunnel: w159 -> [_ w239]
          tunnel: [w230 w238] -> w151
          tunnel: [w231 w237] -> w132
          tunnel: [w231 w236] -> w131
          tunnel: [w229 w235] -> w152
          tunnel: w144 -> [_ w234]
          tunnel: w143 -> [_ w233]
          tunnel: w129 -> [_ w232]
          frame False {
            w229 = sgl 0.0 ("f")
            w231 = FALSE
            # "FALSE"
            # "F"
            n77 = Bundle("f"=w229, "f"=w229) -> (w230:cluster{"f":sgl, "f":sgl})  [unwired: 1 in]
          }
          frame True {
            # "Number of Beacons"
            # "**maybe add case\nto handle if some arent\nsame direction"
            # "Check 1st element\nwith rest of elements"
            # "Find delta X and delta Y\nto Each Camera from Each Beacon"
            # "Make Sure all Pointed \nIn Same Direction"
            # "For Each Valid Beacon\nCalculate Distance from Each Camera to Each Beacon"
            n78 = for {
              N: w244 -> [_]
              tunnel: w245 -> [w719] mode=indexing
              tunnel: w243 -> [w718] mode=indexing
              tunnel: w242 -> [w717] mode=indexing
              tunnel: "Distance Between \nCameras  (*unit)" -> [w716]
              tunnel: "Distance Threshold\nRef Triangles (*unit)" -> [w715]
              tunnel: [w714] -> w250 mode=indexing
              tunnel: [w713] -> _ mode=indexing
              tunnel: [w712] -> w251 mode=indexing
              tunnel: [w711] -> w247 mode=indexing
              tunnel: [w710] -> w246 mode=indexing
              tunnel: [w709] -> w252 mode=indexing
              n79 = case shown="True" w719 {
                tunnel: w718 -> [w724 w734]
                tunnel: w717 -> [w723 w733]
                tunnel: w716 -> [_ w725]
                tunnel: w715 -> [_ w726]
                tunnel: [w724 w732] -> w714
                tunnel: [w723 w731] -> w713
                tunnel: [FALSE w730] -> w712
                tunnel: [w721 w729] -> w711
                tunnel: [w721 w728] -> w710
                tunnel: [0 w727] -> w709
                frame False {
                  w721 = sgl 1.0
                }
                frame True {
                  # "Build Reference Triangle"
                  n80 = call "Position Calc_Build Reference Triangle_R1.vi"("A2_in"=w734, "A3_in"=w733, "S1 (Length Between\n Cameras - inches)"=w725, "Distance\nThreshold"=w726) -> ("S2"=w729:sgl, "S3"=w728:sgl, "Direction"=w727:i8, "A2"=w732:sgl, "A3"=w731:sgl, "Accept"=w730:bool)  [unwired: 6 in]
                }
              }
            }
            "Valid Data\nSets" <- w251
            n81 = Bundle(w247, w246) -> (→"Distance to Each Beacon":cluster{sgl[], sgl[]})  [unwired: 1 in]
            n82 = Boolean To (0,1)(Boolean=w251) -> (0, 1=w260:i16[])
            n83 = for {
              N: w244 -> [_]
              tunnel: w251 -> [w262] mode=indexing
              tunnel: w252 -> [w263] mode=indexing
              tunnel: [w263] -> w257 mode=indexing if=w262
              # "Only add to array\nif valid distance"
            }
            n84 = Add Array Elements(numeric array=w260) -> (sum=w248:i16)
            n85 = Greater?(x=w248, y=1) -> (0:w254:bool)
            n86 = Index Array(array=w257, index=0) -> (element=w256:i32)
            n87 = Equal?(x=w257, y=w256) -> (x = y?=w255:bool[])
            n88 = And Array Elements(Boolean array=w255) -> (logical AND=w253:bool)
            "All Same\nDirection" <- w253
            n89 = case shown="True" w253 {
              tunnel: w244 -> [_ w284]
              tunnel: w251 -> [_ w288]
              tunnel: w254 -> [_ w287]
              tunnel: w246 -> [_ w285]
              tunnel: w247 -> [_ _]
              tunnel: w250 -> [_ w286]
              tunnel: w248 -> [_ w283]
              tunnel: w247 -> [_ w282]
              tunnel: w246 -> [_ w281]
              tunnel: w243 -> [_ w280]
              tunnel: w242 -> [_ w279]
              tunnel: w240 -> [_ w278]
              tunnel: "Distance Between \nCameras  (*unit)" -> [_ w277]
              tunnel: w239 -> [_ w276]
              tunnel: [w265 w275] -> w238
              tunnel: [w266 w274] -> w237
              tunnel: [w266 w273] -> w236
              tunnel: [w264 w272] -> w235
              tunnel: w234 -> [_ w271]
              tunnel: w233 -> [_ w270]
              tunnel: w232 -> [_ w269]
              frame False {
                w264 = sgl 0.0 ("f")
                w266 = FALSE
                w267 = 0
                w268 = sgl 0.0
                (unwired) FALSE
                # "FALSE"
                n90 = Build Array(w268, w268, w268) -> ()  [unwired: 1 out]
                n91 = Build Array(w268, w268, w268) -> ()  [unwired: 1 out]
                n92 = Build Array(w268, w268, w268) -> ()  [unwired: 1 out]
                n93 = Build Array(w268, w268, w268) -> ()  [unwired: 1 out]
                n94 = Build Array(w268, w268, w268) -> ()  [unwired: 1 out]
                n95 = Build Array(w268, w268, w268) -> ()  [unwired: 1 out]
                n96 = Build Array(w267, w267, w267) -> ()  [unwired: 1 out]
                n97 = Bundle("f"=w264, "f"=w264) -> (w265:cluster{"f":sgl, "f":sgl})  [unwired: 1 in]
              }
              frame True {
                # "All Values in Same Direction"
                n98 = case shown="True" w287 {
                  tunnel: w284 -> [_ w306]
                  tunnel: w288 -> [_ w376]
                  tunnel: w286 -> [_ w375]
                  tunnel: w285 -> [_ w374]
                  tunnel: w283 -> [_ _]
                  tunnel: w282 -> [_ _]
                  tunnel: w281 -> [_ _]
                  tunnel: w280 -> [_ _]
                  tunnel: w279 -> [_ _]
                  tunnel: w278 -> [_ _]
                  tunnel: w277 -> [_ w339]
                  tunnel: w276 -> [_ w324]
                  tunnel: [w291 w321] -> w275
                  tunnel: [w289 w318] -> w274
                  tunnel: [w289 w312] -> w273
                  tunnel: [w290 w309] -> w272
                  tunnel: w271 -> [_ w313]
                  tunnel: w270 -> [_ w314]
                  tunnel: w269 -> [_ w302]
                  frame False {
                    w290 = sgl 0.0 ("f")
                    w289 = FALSE
                    w292 = 0
                    w293 = sgl 0.0
                    (unwired) FALSE
                    # "FALSE"
                    # "1 Valid Data Set\n\nRun Single Position Calc for each?\n\nor estimate position based on previous \nposition and orientation"
                    n99 = Build Array(w293, w293, w293) -> ()  [unwired: 1 out]
                    n100 = Build Array(w293, w293, w293) -> ()  [unwired: 1 out]
                    n101 = Build Array(w293, w293, w293) -> ()  [unwired: 1 out]
                    n102 = Build Array(w293, w293, w293) -> ()  [unwired: 1 out]
                    n103 = Build Array(w293, w293, w293) -> ()  [unwired: 1 out]
                    n104 = Build Array(w293, w293, w293) -> ()  [unwired: 1 out]
                    n105 = Build Array(w292, w292, w292) -> ()  [unwired: 1 out]
                    n106 = Bundle("f"=w290, "f"=w290) -> (w291:cluster{"f":sgl, "f":sgl})  [unwired: 1 in]
                  }
                  frame True {
                    w350 = sgl 2.0
                    w369 = 0
                    # "Only Apply This Filtering \nif 3 or More Beacons Still Valid"
                    # "Orientation Value"
                    # "Orientation Valid"
                    # "Y (current)"
                    # "X (current)"
                    # "Number of Valid\nPrevious Orientations"
                    # "Position Valid Shift Array"
                    # "More than 1 Previous\nValid Positions"
                    # "More than\n1 previous position\navailable"
                    # "Choose Beacon Set\nwith Lowest Std Dev"
                    # "Y value cannot be negative"
                    # "Find New # Of Valid Beacons"
                    # "Adjust/Normalize\nLocal Beacon Positions\nusing Line of Best fit"
                    # "# Valid\nData Sets"
                    # "cam, y"
                    # "cam, x"
                    # "Calculate dX and dY\nfor right cam"
                    # "Average dX and dY from each (valid) beacon to find position of each camera\n\nthen average all  positions for each camera find center between"
                    # "Convert Slope\nto Radians"
                    # "*rotate CCW in rad"
                    # "Rotate Coordinate\n System by Slope"
                    # "2+ Data Sets"
                    n107 = for {
                      N: w306 -> [_]
                      tunnel: w376 -> [w677] mode=indexing
                      tunnel: w375 -> [w681] mode=indexing
                      tunnel: w374 -> [w680] mode=indexing
                      tunnel: [w679] -> w332 mode=indexing
                      tunnel: [w678] -> w331 mode=indexing
                      tunnel: [w676] -> w317 mode=indexing
                      n108 = case shown="True" w677 {
                        selector: w677 -> [w683 w687]
                        tunnel: w681 -> [_ w695]
                        tunnel: [w682 w685] -> w679
                        tunnel: [w682 w686] -> w678
                        tunnel: w680 -> [_ w684]
                        tunnel: [w683 w687] -> w676
                        frame False {
                          w682 = sgl 0.0
                          # "Current Data Set Was Not Valid\nFill with 0\nWill not be used later"
                        }
                        frame True {
                          # "dY"
                          # "dX"
                          # "Negate dX if A2>90"
                          # "Find LOCAL Coordinate of Each Beacon"
                          # "Current - Valid Data Set"
                          n109 = Less?(x=w695, y=sgl 90.0) -> (x < y?=w697:bool)
                          n110 = case shown="False" w697 {
                            tunnel: w695 -> [w704 w706]
                            tunnel: [w702 w707] -> w694
                            tunnel: [FALSE TRUE] -> w689
                            frame False {
                              # "Negative Y"
                              # "A2 is > 90"
                              n111 = Subtract(x=w704, y=sgl 90.0) -> (x-y=w702:sgl)
                            }
                            frame True {
                              # "Positive Y"
                              # "A2 is < 90"
                              n112 = Subtract(x=sgl 90.0, y=w706) -> (x-y=w707:sgl)
                            }
                          }
                          "dA2" <- w694
                          n113 = expression code="(x/180.0)*pi" "degrees to radians"(w694) -> (w692:sgl)
                          n114 = expression code="(x/180.0)*pi" "degrees to radians"(w694) -> (w693:sgl)
                          n115 = Cosine(x=w692) -> (cos(x)=w690:sgl)
                          n116 = Sine(x=w693) -> (sin(x)=w691:sgl)
                          n117 = Multiply(x=w684, y=w690) -> (x*y=w686:sgl)
                          n118 = Multiply(x=w684, y=w691) -> (x*y=w688:sgl)
                          n119 = case shown="True" w689 {
                            tunnel: w688 -> [w699 w700]
                            tunnel: [w698 w700] -> w685
                            frame False {
                              n120 = Negate(x=w699) -> (-x=w698:sgl)
                            }
                            frame True {
                            }
                          }
                        }
                      }
                    }
                    n121 = Boolean To (0,1)(Boolean=w313) -> (0, 1=w327:i16[])
                    n122 = Add Array Elements(numeric array=w327) -> (sum=w311:i16)
                    n123 = Greater?(x=w311, y=1) -> (0:w315:bool)
                    n124 = Bundle(w332, w331) -> (→"LOCAL\nBeacon Coordinates\nRelative to Robot" →"Local Coordinates - Calculated":cluster{sgl[], sgl[]})  [unwired: 1 in]
                    n125 = call "Coordinate_Outlier_Filtering_R2.vi"("Num of Beacons"=w306, "Max Std Dev(all 5)"="Max Std Dev (5)", "X in"=w332, "Valid Data\nSets in"=w317, "Y in"=w331, "Max Std Dev( 4 )"="Max Std Dev (4)", "Max Std Dev (3)"="Max Std Dev (3)") -> ("Y out"=w304:sgl[], "X out"=w305:sgl[], "Valid Beacons\nout"=w301:bool[], "Slope out"=w320:dbl)  [unwired: 3 in, 2 out]
                    n126 = Inverse Tangent(1:w320) -> (0:w344:dbl)
                    n127 = expression code="(x/pi)*180.0" "radians to degrees"(w344) -> (w319:dbl)
                    n128 = Boolean To (0,1)(Boolean=w301) -> (0, 1=w300:i16[])
                    n129 = To Single Precision Float(number=w319) -> (single precision float=w310:sgl)
                    "Orietnation\n(current)" <- w310
                    n130 = case shown="False" w315 {
                      tunnel: w313 -> [_ w410]
                      tunnel: [w386 w396] -> w312
                      tunnel: w314 -> [_ w397]
                      tunnel: w310 -> [w387 w391]
                      tunnel: [w385 w392] -> w309
                      tunnel: w302 -> [_ _]
                      frame False {
                        # "Since no history available,\ncheck that current is with 0-360"
                        # "Use Current Orientation bc \nPrevious are not available"
                        # "New Position\nValid"
                        n131 = In Range and Coerce(upper limit=sgl 360.0, x=w387, lower limit=sgl -360.0 ("upper limit")) -> (In Range?=w386:bool)  [unwired: 1 out]
                        n132 = Select(t=w387, s=w386, f=sgl 0.0) -> (s? t:f=w385:sgl)
                      }
                      frame True {
                        # "Valid Position Ccount\n(up to 2)"
                        # "Weighted\nOrientation"
                        # "New \nWeight"
                        # "Weighted Orientation (new)"
                        # "Position\nValid\n(current)\n\nbased on orientation"
                        # "Only Calculate MOving Avg\nif xx% of previous positions were valid"
                        n133 = Initialize Array(u8 0, u8 2) -> (w405:u8[])
                        n134 = local read "History Size"() -> (w406:u8)
                        n135 = while {
                          shift-right: [w461] -> w398
                          shift-left: w405 -> [w463]
                          tunnel: w410 -> [w470] mode=indexing
                          shift-right: [w468] -> w403
                          shift-left: u8 0 -> [w471]
                          tunnel: w406 -> [w469]
                          i -> [w462]
                          stop <- w464 stop-if-true
                          # "Grab Last 2 Valid Position Indexes"
                          n136 = case shown="True" w470 {
                            tunnel: w471 -> [w473 w475]
                            tunnel: [w473 w478] -> w468
                            tunnel: w463 -> [w472 w477]
                            tunnel: w462 -> [_ w476]
                            tunnel: [w472 w474] -> w461
                            frame False {
                            }
                            frame True {
                              # "Update Index\nto use"
                              # "Increment\nValid Count"
                              n137 = Replace Array Subset(array=w477, new element=w476, index=w475) -> (w474:u8[])
                              n138 = Increment(x=w475) -> (x+1=w478:u8)
                            }
                          }
                          n139 = Greater?(x=w462, y=w469) -> (0:w465:bool)
                          n140 = Greater?(x=w468, y=u8 2) -> (0:w466:bool)
                          n141 = Or(x=w466, y=w465) -> (x .or. y?=w464:bool)
                        }
                        n142 = case shown="2, Default" w403 {
                          tunnel: w398 -> [_ w445 w457]
                          tunnel: w397 -> [_ w446 w456]
                          tunnel: [sgl 0.0 ("y") w439 w452] -> w401
                          tunnel: "Orientation (-2) \nWeight" -> [w431 w442 w451]
                          tunnel: "Orientation (-1) \nWeight" -> [w433 w435 w449]
                          tunnel: "New Orientation\nWeight" -> [w432 w437 w450]
                          tunnel: [w430 w436 w450] -> w402
                          frame 0 {
                            n143 = Compound Arithmetic op=ADD(w433, w432, w431) -> (w430:sgl)
                          }
                          frame 1 {
                            # "Grab Last 1 Valid Position Values"
                            n144 = Index Array(array=w445, index=u8 0) -> (element=w443:u8)
                            n145 = Index Array(array=w446, index=w443) -> (element=w434:sgl)
                            n146 = Divide(x=w442, y=sgl 2.0) -> (x/y=w438:sgl)
                            n147 = Add(x=w435, y=w438) -> (x+y=w440:sgl)
                            n148 = Add(x=w438, y=w437) -> (x+y=w436:sgl)
                            n149 = Multiply(x=w434, y=w440) -> (x*y=w439:sgl)
                          }
                          frame 2, Default {
                            # "weighted vals"
                            # "Grab Last 2 Valid Position Values"
                            n150 = Index Array(array=w457, index=u8 0) -> (element=w459:u8)
                            n151 = Index Array(array=w457, index=u8 1) -> (element=w455:u8)
                            n152 = Index Array(array=w456, index=w459) -> (element=w448:sgl)
                            n153 = Index Array(array=w456, index=w455) -> (element=w447:sgl)
                            n154 = Multiply(x=w449, y=w448) -> (x*y=w453:sgl)
                            n155 = Multiply(x=w447, y=w451) -> (x*y=w454:sgl)
                            n156 = Add(x=w453, y=w454) -> (x+y=w452:sgl)
                          }
                        }
                        n157 = Multiply(x=w391, y=w402) -> (x*y=w400:sgl)
                        n158 = Add(x=w400, y=w401) -> (x+y=w399:sgl)
                        n159 = Greater Than 0?(x=w403) -> (x > 0?=w404:bool)
                        n160 = case shown="True" w404 {
                          tunnel: w399 -> [w413 w418]
                          tunnel: w398 -> [_ w426]
                          tunnel: w397 -> [_ w425]
                          tunnel: [w412 w417] -> w392
                          tunnel: [w411 w420] -> w396
                          frame False {
                            # "No Pevious is Available to Compare\ncheck that current is real angle"
                            n161 = In Range and Coerce(upper limit=sgl 360.0, x=w413, lower limit=sgl -360.0 ("upper limit")) -> (In Range?=w411:bool)  [unwired: 1 out]
                            n162 = Select(t=w413, s=w411, f=sgl 0.0) -> (s? t:f=w412:sgl)
                          }
                          frame True {
                            # "Calculate New, Weighted\nOrientation"
                            # "Check That New Value\nis within Range of Old\n(avg)"
                            # "(X1 - X2)^2"
                            # "Previous"
                            # "Pevious is Available to Compare"
                            n163 = Index Array(array=w426, index=u8 0) -> (element=w427:u8)
                            n164 = Index Array(array=w425, index=w427) -> (element=w423:sgl)
                            n165 = Subtract(x=w423, y=w418) -> (x-y=w422:sgl)
                            n166 = Absolute Value(x=w422) -> (abs(x)=w421:sgl)
                            n167 = Less Or Equal?(x=w421, y="New Orientation \nThreshold") -> (x <= y?=w420:bool)
                            n168 = Select(t=w418, s=w420, f=sgl 0.0) -> (s? t:f=w417:sgl)
                          }
                        }
                      }
                    }
                    n169 = Add Array Elements(numeric array=w300) -> (sum=w299:i16)
                    n170 = Greater?(x=w299, y=i16 2) -> (0:w297:bool)
                    n171 = case shown="True" w297 {
                      tunnel: w306 -> [_ w384]
                      tunnel: w301 -> [w377 w383]
                      tunnel: w305 -> [_ w382]
                      tunnel: w304 -> [_ w381]
                      tunnel: [w377 w380] -> w303
                      tunnel: "Distance\nBetween Beacons" -> [_ w379]
                      tunnel: "Distance\nBetween Beacons \n- Tolerance" -> [_ w378]
                      frame False {
                        # "Don't apply filtering,\nnot enough data points"
                      }
                      frame True {
                        # "This will filter beacons if they are calculate to be \ntoo close to each other. The beacon(s) that is\n discarded is chosen based distance between each/every\nbeacon,. Capable of filtering as long as 1/2 of sample\nset has uniform distances (between beacons)."
                        # "Validate Distance Between\nEach Beacon"
                        n172 = call "Beacon_Filtering_Inter_Beacon_Distance_R1.vi"("Num of Beacons"=w384, "Inter Beacon\nReal Distance"=w379, "X in"=w382, "Inter Beacon\ndelta Threshold"=w378, "Y in"=w381, "Valid Data\nSets in"=w383) -> ("Beacons Valid - Out"=w380:bool[])  [unwired: 9 in]
                      }
                    }
                    "Post Filtering\n- Valid Beacons" <- w303
                    n173 = Bundle("X out"=w305, "Y out"=w304) -> (→"Normalized Beacons\nCoordinates Relative\nto Robot\n- Local" →"Local Coordinates - Adjusted":cluster{"X out":sgl[], "Y out":sgl[]})  [unwired: 1 in]
                    n174 = Increment(x=w306) -> (x+1=w370:i8)
                    n175 = for {
                      N: w370 -> [_]
                      tunnel: [w666] -> w372 mode=indexing
                      tunnel: w305 -> [w662]
                      tunnel: w304 -> [w665]
                      tunnel: [w664] -> w373 mode=indexing
                      tunnel: w339 -> [w661]
                      i -> [w663]
                      # "Build Array's of Coordinates\nFor All Objects"
                      n176 = Greater Than 0?(x=w663) -> (x > 0?=w667:bool)
                      n177 = case shown="True" w667 {
                        tunnel: [w669 w675] -> w666
                        tunnel: w662 -> [w672 _]
                        tunnel: w665 -> [w671 _]
                        tunnel: [w668 0.0] -> w664
                        tunnel: w663 -> [w673 _]
                        tunnel: w661 -> [_ w675]
                        frame True {
                          # "Rest of Array is\nBeacon Coordinates"
                          n178 = Decrement(x=w673) -> (x-1=w670:i32)
                          n179 = Index Array(array=w672, index=w670) -> (element=w669:sgl)
                          n180 = Index Array(array=w671, index=w670) -> (element=w668:sgl)
                        }
                        frame False {
                          # "First object is the\nother Camera\n\nthis coordinate\nis simply:\nx = 0\ny = distance btween cams"
                        }
                      }
                    }
                    n181 = Bundle(w372, w373) -> (→"All Object Coordinates \n- Local" →"Local Coordinates - Normalized":cluster{sgl[], dbl[]})  [unwired: 1 in]
                    n182 = expression code="(x/180.0)*pi" "degrees to radians"(w309) -> (w316:sgl)
                    n183 = call-poly <vilib>:"2D Cartesian Coordinate Rotation.vi"("theta"=w316, "Y"=w373, "X"=w372) -> ("Y Out"=w347:dbl[], "X Out"=w348:dbl[])  [unwired: 6 in, 1 out]
                    n184 = Bundle("X Out"=w348, "Y Out"=w347) -> (→"All Object Coordinates \n- Local - Rotated" →"Local Coordinates - Rotated":cluster{"X Out":dbl[], "Y Out":dbl[]})  [unwired: 1 in]
                    n185 = Index Array(array=w347, index=w369) -> (element=w340:dbl)
                    n186 = Index Array(array=w348, index=w369) -> (element=w368:dbl)
                    n187 = for {
                      N: w306 -> [_]
                      tunnel: w347 -> [w657]
                      tunnel: w348 -> [w658]
                      tunnel: w368 -> [w656]
                      tunnel: w340 -> [w655]
                      tunnel: [w654] -> w336 mode=indexing
                      tunnel: [w653] -> w335 mode=indexing
                      tunnel: [w652] -> w294 mode=indexing
                      tunnel: [w651] -> w337 mode=indexing
                      i -> [w660]
                      n188 = Increment(x=w660) -> (x+1=w659:i32)
                      n189 = Index Array(array=w657, index=w659) -> (element=w651:dbl)
                      n190 = Index Array(array=w658, index=w659) -> (element=w652:dbl)
                      n191 = Subtract(x=w651, y=w655) -> (x-y=w653:dbl)
                      n192 = Subtract(x=w652, y=w656) -> (x-y=w654:dbl)
                    }
                    n193 = Bundle(w336, w335) -> (→"dX, dY\nRight Cam":cluster{dbl[], dbl[]})  [unwired: 1 in]
                    n194 = Bundle(w294, w337) -> (→"dX, dY\nLeft Cam":cluster{dbl[], dbl[]})  [unwired: 1 in]
                    n195 = Unbundle("Real Beacon\n - Coordinates") -> ("X"=w365:dbl[], "Y"=w341:dbl[])
                    n196 = Boolean To (0,1)(Boolean=w303) -> (0, 1=w338:i16[])
                    n197 = for {
                      N: w306 -> [_]
                      tunnel: w303 -> [w637] mode=indexing
                      tunnel: w365 -> [w634] mode=indexing
                      tunnel: w341 -> [w633] mode=indexing
                      tunnel: w294 -> [w636] mode=indexing
                      tunnel: w337 -> [w632] mode=indexing
                      tunnel: w336 -> [w635] mode=indexing
                      tunnel: w335 -> [w631] mode=indexing
                      tunnel: [w630] -> w364 mode=indexing
                      tunnel: [w629] -> w363 mode=indexing
                      tunnel: [w628] -> w362 mode=indexing
                      tunnel: [w627] -> w361 mode=indexing
                      n198 = case shown="True" w637 {
                        tunnel: w636 -> [_ w650]
                        tunnel: w635 -> [_ w649]
                        tunnel: w634 -> [_ w640]
                        tunnel: w633 -> [_ w639]
                        tunnel: w632 -> [_ w648]
                        tunnel: w631 -> [_ w641]
                        tunnel: [w638 w646] -> w630
                        tunnel: [w638 w645] -> w629
                        tunnel: [w638 w644] -> w628
                        tunnel: [w638 w643] -> w627
                        frame False {
                          w638 = sgl 0.0
                          # "Add Nothing"
                        }
                        frame True {
                          # "realX = beaconX + dY\nrealY = beaconY + (-dx)"
                          # "Right Cam"
                          # "Left Cam"
                          # "dX = -dX\nSwap dX, dY"
                          # "Translate to Real Coordinates\nOnly Apply for Valid Beacons"
                          n199 = Negate(x=w650) -> (-x=w647:dbl)
                          n200 = Negate(x=w649) -> (-x=w642:dbl)
                          n201 = Add(x=w640, y=w648) -> (x+y=w646:dbl)
                          n202 = Add(x=w639, y=w647) -> (x+y=w645:dbl)
                          n203 = Add(x=w640, y=w641) -> (x+y=w644:dbl)
                          n204 = Add(x=w639, y=w642) -> (x+y=w643:dbl)
                        }
                      }
                    }
                    n205 = Add Array Elements(numeric array=w338) -> (sum=w342:i16)
                    n206 = Add Array Elements(numeric array=w364) -> (sum=w360:dbl)
                    n207 = Add Array Elements(numeric array=w363) -> (sum=w359:dbl)
                    n208 = Add Array Elements(numeric array=w362) -> (sum=w358:dbl)
                    n209 = Add Array Elements(numeric array=w361) -> (sum=w357:dbl)
                    n210 = Divide(x=w360, y=w342) -> (x/y=w355:dbl)
                    n211 = Divide(x=w359, y=w342) -> (x/y=w353:dbl)
                    n212 = Divide(x=w358, y=w342) -> (x/y=w354:dbl)
                    n213 = Divide(x=w357, y=w342) -> (x/y=w352:dbl)
                    n214 = Bundle(w355, w353) -> (→"Left Camera Real Coordinates":cluster{dbl, dbl})  [unwired: 1 in]
                    n215 = Bundle(w354, w352) -> (→"Right Camera Real Coordinate":cluster{dbl, dbl})  [unwired: 1 in]
                    n216 = Add(x=w355, y=w354) -> (x+y=w351:dbl)
                    n217 = Add(x=w353, y=w352) -> (x+y=w349:dbl)
                    n218 = Divide(x=w351, y=w350) -> (x/y=w323:dbl)
                    n219 = Divide(x=w349, y=w350) -> (x/y=w322:dbl)
                    n220 = Bundle(w323, w322) -> (→"Robot Coordinates":cluster{dbl, dbl})  [unwired: 1 in]
                    n221 = case shown="False" w315 {
                      tunnel: w313 -> [_ w517]
                      tunnel: w311 -> [_ _]
                      tunnel: w323 -> [w483 w505]
                      tunnel: [w484 w495] -> w318
                      tunnel: w324 -> [_ w490]
                      tunnel: w322 -> [w482 w504]
                      tunnel: [w481 w516] -> w321
                      tunnel: "Max X (arena)" -> [w480 w493]
                      tunnel: "Max Y (arena)" -> [w479 w492]
                      frame False {
                        # "New Position\nValid"
                        # "Since no history available,\ncheck that current is within\nthe bounds of the arena size"
                        # "Use Current Position bc \nPrevious are not available"
                        n222 = In Range and Coerce(upper limit=w480, x=w483, lower limit=sgl 0.0 ("upper limit")) -> (In Range?=w486:bool)  [unwired: 1 out]
                        n223 = In Range and Coerce(upper limit=w479, x=w482, lower limit=sgl 0.0 ("upper limit")) -> (In Range?=w485:bool)  [unwired: 1 out]
                        n224 = Bundle(w483, w482) -> (w481:cluster{dbl, dbl})  [unwired: 1 in]
                        n225 = And(x=w486, y=w485) -> (x .and. y?=w484:bool)
                      }
                      frame True {
                        # "Only consider if velocity is\ngreater than certain speed"
                        # "Valid Position Ccount\n(up to 2)"
                        # "Weighted Y"
                        # "Weighted X"
                        # "New Pos\nWeight"
                        # "Weighted Robot \nCoordinates"
                        # "Position\nValid\n(current)"
                        # "Only Calculate MOving Avg\nif xx% of previous positions were valid"
                        n226 = Initialize Array(u8 0, u8 2) -> (w511:u8[])
                        n227 = local read "History Size"() -> (w512:u8)
                        n228 = while {
                          shift-right: [w610] -> w489
                          shift-left: w511 -> [w612]
                          tunnel: w517 -> [w618] mode=indexing
                          shift-right: [w616] -> w507
                          shift-left: u8 0 -> [w619]
                          tunnel: w512 -> [w617]
                          tunnel: [w609] -> w491
                          i -> [w611]
                          stop <- w613 stop-if-true
                          # "Grab Last 3 Valid Position Indexes"
                          n229 = case shown="True" w618 {
                            tunnel: w619 -> [w621 w623]
                            tunnel: [w621 w626] -> w616
                            tunnel: w612 -> [w620 w625]
                            tunnel: w611 -> [_ w624]
                            tunnel: [w620 w622] -> w610
                            frame False {
                            }
                            frame True {
                              # "Update Index\nto use"
                              # "Increment\nValid Count"
                              n230 = Replace Array Subset(array=w625, new element=w624, index=w623) -> (w622:u8[])
                              n231 = Increment(x=w623) -> (x+1=w626:u8)
                            }
                          }
                          n232 = Greater?(x=w611, y=w617) -> (0:w614:bool)
                          n233 = Greater?(x=w616, y=u8 2) -> (0:w609:bool)
                          n234 = Or(x=w609, y=w614) -> (x .or. y?=w613:bool)
                        }
                        n235 = case shown="True" w491 {
                          tunnel: w490 -> [_ w539]
                          tunnel: w489 -> [_ w525]
                          frame False {
                          }
                          frame True {
                            # "Angle between p(1) - p(2)"
                            # "Angle between p(0) - p(1)"
                            # "Calculate Orientation Based on Recent Positions"
                            # "*******"
                            n236 = Index Array(array=w525, index #1=0, index #2=1, index #3=2) -> (element #1=w521:u8, element #2=w520:u8, element #3=w519:u8)
                            n237 = Index Array(array=w539, index=w521) -> (element=w538:cluster{sgl, sgl})
                            n238 = Unbundle(w538) -> (w535:sgl, w534:sgl)
                            n239 = Index Array(array=w539, index=w520) -> (element=w537:cluster{sgl, sgl})
                            n240 = Unbundle(w537) -> (w527:sgl, w526:sgl)
                            n241 = Subtract(x=w535, y=w527) -> (x-y=w536:sgl)
                            n242 = Subtract(x=w534, y=w526) -> (x-y=w533:sgl)
                            n243 = Inverse Tangent (2 Input)(1:w533, 2:w536) -> (0:→"atan2(y,x)":sgl)
                            n244 = Index Array(array=w539, index=w519) -> (element=w528:cluster{sgl, sgl})
                            n245 = Unbundle(w528) -> (w531:sgl, w530:sgl)
                            n246 = Subtract(x=w527, y=w531) -> (x-y=w532:sgl)
                            n247 = Subtract(x=w526, y=w530) -> (x-y=w529:sgl)
                            n248 = Inverse Tangent (2 Input)(1:w529, 2:w532) -> ()  [unwired: 1 out]
                          }
                        }
                        n249 = case shown="2, Default" w507 {
                          tunnel: w489 -> [_ w586 w606]
                          tunnel: w490 -> [_ w587 w605]
                          tunnel: [w567 w576 w594] -> w503
                          tunnel: [w567 w575 w593] -> w502
                          tunnel: "position(-2) weight" -> [w569 w580 w592]
                          tunnel: "position(-1) weight" -> [w571 w578 w591]
                          tunnel: "New Position\nWeight" -> [w570 w573 w590]
                          tunnel: [w568 w572 w590] -> w506
                          frame 0 {
                            w567 = sgl 0.0 ("y")
                            n250 = Compound Arithmetic op=ADD(w571, w570, w569) -> (w568:sgl)
                          }
                          frame 1 {
                            # "Grab Last 1 Valid Position Values"
                            n251 = Index Array(array=w586, index=u8 0) -> (element=w584:u8)
                            n252 = Index Array(array=w587, index=w584) -> (element=w581:cluster{sgl, sgl})
                            n253 = Unbundle(w581) -> (w582:sgl, w583:sgl)
                            n254 = Divide(x=w580, y=sgl 2.0) -> (x/y=w574:sgl)
                            n255 = Add(x=w578, y=w574) -> (x+y=w577:sgl)
                            n256 = Add(x=w574, y=w573) -> (x+y=w572:sgl)
                            n257 = Multiply(x=w582, y=w577) -> (x*y=w576:sgl)
                            n258 = Multiply(x=w583, y=w577) -> (x*y=w575:sgl)
                          }
                          frame 2, Default {
                            # "weighted vals"
                            # "Grab Last 2 Valid Position Values"
                            n259 = Index Array(array=w606, index #1=u8 0, index #2=u8 1) -> (element #1=w607:u8, element #2=w588:u8)
                            n260 = Index Array(array=w605, index=w607) -> (element=w604:cluster{sgl, sgl})
                            n261 = Index Array(array=w605, index=w588) -> (element=w603:cluster{sgl, sgl})
                            n262 = Unbundle(w604) -> (w601:sgl, w602:sgl)
                            n263 = Unbundle(w603) -> (w600:sgl, w599:sgl)
                            n264 = Multiply(x=w601, y=w591) -> (x*y=w597:sgl)
                            n265 = Multiply(x=w602, y=w591) -> (x*y=w596:sgl)
                            n266 = Multiply(x=w600, y=w592) -> (x*y=w598:sgl)
                            n267 = Multiply(x=w599, y=w592) -> (x*y=w595:sgl)
                            n268 = Add(x=w597, y=w598) -> (x+y=w594:sgl)
                            n269 = Add(x=w596, y=w595) -> (x+y=w593:sgl)
                          }
                        }
                        n270 = Multiply(x=w505, y=w506) -> (x*y=w500:dbl)
                        n271 = Multiply(x=w504, y=w506) -> (x*y=w501:dbl)
                        n272 = Greater Than 0?(x=w507) -> (x > 0?=w508:bool)
                        n273 = Add(x=w500, y=w503) -> (x+y=w499:dbl)
                        n274 = Add(x=w501, y=w502) -> (x+y=w498:dbl)
                        n275 = case shown="True" w508 {
                          tunnel: w499 -> [w544 w551]
                          tunnel: w498 -> [w543 w550]
                          tunnel: w489 -> [_ w563]
                          tunnel: w490 -> [_ w562]
                          tunnel: [w541 w551] -> w497
                          tunnel: [w540 w550] -> w496
                          tunnel: [w545 w552] -> w495
                          tunnel: w493 -> [w547 _]
                          tunnel: w492 -> [w546 _]
                          frame False {
                            w542 = sgl 0.0 ("upper limit")
                            # "Check that within bounds of arena"
                            # "No Pevious is Available to Compare"
                            n276 = In Range and Coerce(upper limit=w547, x=w544, lower limit=w542) -> (In Range?=w549:bool)  [unwired: 1 out]
                            n277 = In Range and Coerce(upper limit=w546, x=w543, lower limit=w542) -> (In Range?=w548:bool)  [unwired: 1 out]
                            n278 = And(x=w549, y=w548) -> (x .and. y?=w545:bool)
                            n279 = Select(t=w544, s=w545, f=w542) -> (s? t:f=w541:dbl)
                            n280 = Select(t=w543, s=w545, f=w542) -> (s? t:f=w540:dbl)
                          }
                          frame True {
                            # "New"
                            # "(Y1 - Y2)^2"
                            # "(X1 - X2)^2"
                            # "Previous"
                            # "Pevious is Available to Compare"
                            n281 = Index Array(array=w563, index=u8 0) -> (element=w565:u8)
                            n282 = Index Array(array=w562, index=w565) -> (element=w564:cluster{sgl, sgl})
                            n283 = Unbundle(w564) -> (w554:sgl, w553:sgl)
                            n284 = Subtract(x=w554, y=w551) -> (x-y=w559:dbl)
                            n285 = Subtract(x=w550, y=w553) -> (x-y=w558:dbl)
                            n286 = Square(x=w559) -> (x^2=w557:dbl)
                            n287 = Square(x=w558) -> (x^2=w556:dbl)
                            n288 = Add(x=w557, y=w556) -> (x+y=w560:dbl)
                            n289 = Square Root(x=w560) -> (sqrt(x)=w555:dbl)
                            n290 = Less Or Equal?(x=w555, y="New Position \nThreshold") -> (x <= y?=w552:bool)
                          }
                        }
                        n291 = Bundle("upper limit"=w497, "upper limit"=w496) -> (w516:cluster{"upper limit":dbl, "upper limit":dbl})  [unwired: 1 in]
                      }
                    }
                    n292 = Less Than 0?(x=w322) -> ()  [unwired: 1 out]
                  }
                }
              }
            }
          }
        }
        n293 = And(x=w132, y=w131) -> (x .and. y?=w136:bool)
        "Position Valid" <- w136
        n294 = Exclusive Or(1:w131, 2:w132) -> (0:w130:bool)
        n295 = case shown="True" w136 {
          tunnel: [w171 w174] -> w150
          tunnel: [w172 w173] -> w135
          tunnel: w152 -> [_ w174]
          tunnel: w151 -> [_ w173]
          tunnel: w130 -> [_ _]
          frame False {
            w171 = sgl 0.0 ("f")
            n296 = Bundle("f"=w171, "f"=w171) -> (w172:cluster{"f":sgl, "f":sgl})  [unwired: 1 in]
          }
          frame True {
            # "For Servos"
            "Last Orientation" <- w174
            "Last Position" <- w173
          }
        }
        "Robot Coordinates - Avgd" <- w135
        "Orientation Avgd" <- w150
        n297 = local read "History Size"() -> (w142:u8)
        n298 = Reverse 1D Array(array=w149) -> (reversed array=w155:cluster{sgl, sgl}[])
        n299 = for {
          N: w142 -> [w212]
          shift-right: [w213] -> w156
          shift-left: w155 -> [w208]
          tunnel: w135 -> [w207]
          i -> [w209]
          n300 = Decrement(x=w212) -> (x-1=w210:i32)
          n301 = Equal?(x=w210, y=w209) -> (x = y?=w211:bool)
          n302 = case shown="True" w211 {
            tunnel: w209 -> [w215 w220]
            tunnel: w208 -> [w218 w221]
            tunnel: [w216 w222] -> w213
            tunnel: w207 -> [_ w219]
            frame False {
              n303 = Increment(x=w215) -> (x+1=w214:i32)
              n304 = Index Array(array=w218, index=w214) -> (element=w217:cluster{sgl, sgl})
              n305 = Replace Array Subset(array=w218, new element=w217, index=w215) -> (w216:cluster{sgl, sgl}[])
            }
            frame True {
              n306 = Replace Array Subset(array=w221, new element=w219, index=w220) -> (w222:cluster{sgl, sgl}[])
            }
          }
        }
        n307 = Reverse 1D Array(array=w148) -> (reversed array=w157:sgl[])
        n308 = Reverse 1D Array(array=w156) -> (reversed array=w145:cluster{sgl, sgl}[])
        n309 = for {
          N: w142 -> [w196]
          shift-right: [w197] -> w158
          shift-left: w157 -> [w192]
          tunnel: w150 -> [w191]
          i -> [w193]
          n310 = Decrement(x=w196) -> (x-1=w194:i32)
          n311 = Equal?(x=w194, y=w193) -> (x = y?=w195:bool)
          n312 = case shown="True" w195 {
            tunnel: w193 -> [w199 w204]
            tunnel: w192 -> [w202 w205]
            tunnel: [w200 w206] -> w197
            tunnel: w191 -> [_ w203]
            frame False {
              n313 = Increment(x=w199) -> (x+1=w198:i32)
              n314 = Index Array(array=w202, index=w198) -> (element=w201:sgl)
              n315 = Replace Array Subset(array=w202, new element=w201, index=w199) -> (w200:sgl[])
            }
            frame True {
              n316 = Replace Array Subset(array=w205, new element=w203, index=w204) -> (w206:sgl[])
            }
          }
        }
        n317 = Reverse 1D Array(array=w147) -> (reversed array=w153:bool[])
        n318 = Reverse 1D Array(array=w158) -> (reversed array=w146:sgl[])
        n319 = for {
          N: w142 -> [w180]
          shift-right: [w181] -> w154
          shift-left: w153 -> [w176]
          tunnel: w136 -> [w175]
          i -> [w177]
          n320 = Decrement(x=w180) -> (x-1=w178:i32)
          n321 = Equal?(x=w178, y=w177) -> (x = y?=w179:bool)
          n322 = case shown="True" w179 {
            tunnel: w177 -> [w183 w188]
            tunnel: w176 -> [w186 w189]
            tunnel: [w184 w190] -> w181
            tunnel: w175 -> [_ w187]
            frame False {
              n323 = Increment(x=w183) -> (x+1=w182:i32)
              n324 = Index Array(array=w186, index=w182) -> (element=w185:bool)
              n325 = Replace Array Subset(array=w186, new element=w185, index=w183) -> (w184:bool[])
            }
            frame True {
              n326 = Replace Array Subset(array=w189, new element=w187, index=w188) -> (w190:bool[])
            }
          }
        }
        n327 = Reverse 1D Array(array=w154) -> (reversed array=w141:bool[])
        n328 = Boolean To (0,1)(Boolean=w141) -> (0, 1=w140:i16[])
        n329 = Add Array Elements(numeric array=w140) -> (sum=w138:i16)
        n330 = Greater Or Equal?(x=w138, y=i16 2) -> (x >= y?=→"Position \nLock Status":bool)
        n331 = case shown="True" w136 {
          tunnel: w135 -> [_ w170]
          frame False {
          }
          frame True {
            # "update debug graph\nif current is valid"
            n332 = Unbundle(w170) -> ("upper limit"=w169:dbl, "upper limit"=w168:dbl)
            n333 = Build Array(w168) -> (w166:dbl[])
            n334 = Build Array(w169) -> (w167:dbl[])
            n335 = Bundle(w167, w166) -> (→"Real Position in Course 2":cluster{dbl[], dbl[]})  [unwired: 1 in]
          }
        }
      }
    }
    n336 = case shown="True" w105 {
      tunnel: w104 -> [_ w112]
      frame False {
      }
      frame True {
        n337 = call "Tick Count3"() -> ("Tick Count(uSec)"=w113:u32)
        n338 = Subtract(x=w113, y=w112) -> (x-y=w116:u32)
        n339 = Divide(x=w116, y=u32 1000 ("x")) -> (x/y=→"dT":dbl)
      }
    }
    n340 = call "Tick Count6"() -> ("Tick Count(uSec)"=w102:u32)
    "Robot Coordinates\nHistory" <- w101
    "Orientation\nHistory" <- w106
    "Position Valid\nHistory" <- w107
  }
  n341 = disable-structure shown="Disabled" {
    frame Disabled {
      w741 = sgl 0.0
      # "Y"
      # "X"
      n342 = Bundle(w741, w741) -> (w738:cluster{sgl, sgl})  [unwired: 1 in]
      n343 = Initialize Array(w741, 10 ("dimension size")) -> (w735:sgl[])
      n344 = Initialize Array(FALSE, 10 ("dimension size")) -> (w736:bool[])
      n345 = local read "Real Beacon\n - Coordinates"() -> (w742:cluster{"X":dbl[], "Y":dbl[]})
      n346 = Unbundle(w742) -> ("X"=w740:dbl[], "Y"=w739:dbl[])
      n347 = while {
        shift-right: [w768] -> _
        shift-left: w735 -> [w769]
        shift-right: [w752] -> _
        shift-left: w736 -> [w772]
        shift-right: [w754] -> _
        shift-left: w735 -> [w773]
        shift-right: [w755] -> _
        shift-left: w738 -> [w757]
        shift-right: [w751] -> _
        shift-left: FALSE -> [w756]
        tunnel: w740 -> [w748]
        tunnel: w739 -> [w747]
        stop <- FALSE stop-if-true
        w753 = 0
        w765 = 5
        # "Update Shift Regs"
        # "Update Shift Arrays"
        n348 = local read "Robot Coordinates"() -> (w761:cluster{"X":sgl, "Y":sgl})
        n349 = local read "Position Valid"() -> (w762:bool)
        n350 = Unbundle(w761) -> ("X"=w771:sgl, "Y"=w770:sgl)
        n351 = Reverse 1D Array(array=w772) -> (reversed array=w774:bool[])
        n352 = Reverse 1D Array(array=w773) -> (reversed array=w780:sgl[])
        n353 = Reverse 1D Array(array=w769) -> (reversed array=w777:sgl[])
        n354 = for {
          N: 10 -> [w869]
          shift-right: [w870] -> w782
          shift-left: w780 -> [w865]
          tunnel: w771 -> [w864]
          i -> [w866]
          n355 = Decrement(x=w869) -> (x-1=w867:i32)
          n356 = Equal?(x=w867, y=w866) -> (x = y?=w868:bool)
          n357 = case shown="True" w868 {
            tunnel: w866 -> [w872 w877]
            tunnel: w865 -> [w875 w878]
            tunnel: [w873 w879] -> w870
            tunnel: w864 -> [_ w876]
            frame False {
              n358 = Increment(x=w872) -> (x+1=w871:i32)
              n359 = Index Array(array=w875, index=w871) -> (element=w874:sgl)
              n360 = Replace Array Subset(array=w875, new element=w874, index=w872) -> (w873:sgl[])
            }
            frame True {
              n361 = Replace Array Subset(array=w878, new element=w876, index=w877) -> (w879:sgl[])
            }
          }
        }
        n362 = for {
          N: 10 -> [w853]
          shift-right: [w854] -> w779
          shift-left: w777 -> [w849]
          tunnel: w770 -> [w848]
          i -> [w850]
          n363 = Decrement(x=w853) -> (x-1=w851:i32)
          n364 = Equal?(x=w851, y=w850) -> (x = y?=w852:bool)
          n365 = case shown="True" w852 {
            tunnel: w850 -> [w856 w861]
            tunnel: w849 -> [w859 w862]
            tunnel: [w857 w863] -> w854
            tunnel: w848 -> [_ w860]
            frame False {
              n366 = Increment(x=w856) -> (x+1=w855:i32)
              n367 = Index Array(array=w859, index=w855) -> (element=w858:sgl)
              n368 = Replace Array Subset(array=w859, new element=w858, index=w856) -> (w857:sgl[])
            }
            frame True {
              n369 = Replace Array Subset(array=w862, new element=w860, index=w861) -> (w863:sgl[])
            }
          }
        }
        n370 = for {
          N: 10 -> [w837]
          shift-right: [w838] -> w776
          shift-left: w774 -> [w833]
          tunnel: w762 -> [w832]
          i -> [w834]
          n371 = Decrement(x=w837) -> (x-1=w835:i32)
          n372 = Equal?(x=w835, y=w834) -> (x = y?=w836:bool)
          n373 = case shown="False" w836 {
            tunnel: w834 -> [w840 w845]
            tunnel: w833 -> [w843 w846]
            tunnel: [w841 w847] -> w838
            tunnel: w832 -> [_ w844]
            frame False {
              n374 = Increment(x=w840) -> (x+1=w839:i32)
              n375 = Index Array(array=w843, index=w839) -> (element=w842:bool)
              n376 = Replace Array Subset(array=w843, new element=w842, index=w840) -> (w841:bool[])
            }
            frame True {
              n377 = Replace Array Subset(array=w846, new element=w844, index=w845) -> (w847:bool[])
            }
          }
        }
        n378 = Reverse 1D Array(array=w776) -> (reversed array=w752:bool[])
        n379 = Reverse 1D Array(array=w779) -> (reversed array=w768:sgl[])
        n380 = Reverse 1D Array(array=w782) -> (reversed array=w754:sgl[])
        n381 = Boolean To (0,1)(Boolean=w752) -> (0, 1=w767:i16[])
        n382 = Add Array Elements(numeric array=w767) -> (sum=w760:i16)
        n383 = Greater Or Equal?(x=w760, y=3) -> (x >= y?=w758:bool)
        n384 = case shown="True" w758 {
          tunnel: w768 -> [_ w801]
          tunnel: w754 -> [_ w800]
          tunnel: w752 -> [_ w795]
          tunnel: w760 -> [_ w794]
          tunnel: [w786 w787] -> w755
          tunnel: w757 -> [w786 w793]
          tunnel: "New Pos\nThreshold (*unit)\nfilterd UNUSED" -> [_ w792]
          tunnel: w756 -> [_ w791]
          tunnel: [FALSE w790] -> w751
          tunnel: [w784 w789] -> w750
          tunnel: [w784 w788] -> w749
          frame False {
            w784 = sgl 0.0
            # "false bc did not meet\ncriteria for enough previous \nvalid positions"
            # "Retain Last Valid Position Value"
          }
          frame True {
            w799 = sgl 0.0
            # "Only Calculate MOving Avg\nif xx% of previous positions were valid"
            n385 = for {
              N: 10 -> [_]
              tunnel: w795 -> [w823] mode=indexing
              tunnel: w801 -> [w822] mode=indexing
              tunnel: w800 -> [w821] mode=indexing
              shift-right: [w819] -> w797
              shift-left: w799 -> [w820]
              shift-right: [w817] -> w796
              shift-left: w799 -> [w818]
              # "Calculate Moving Average"
              n386 = case shown="True" w823 {
                tunnel: w822 -> [_ w827]
                tunnel: w821 -> [_ w830]
                tunnel: w820 -> [w825 w831]
                tunnel: [w825 w829] -> w819
                tunnel: w818 -> [w824 w828]
                tunnel: [w824 w826] -> w817
                frame False {
                }
                frame True {
                  n387 = Add(x=w831, y=w830) -> (x+y=w829:sgl)
                  n388 = Add(x=w828, y=w827) -> (x+y=w826:sgl)
                }
              }
            }
            n389 = Divide(x=w797, y=w794) -> (x/y=w789:sgl)
            n390 = Divide(x=w796, y=w794) -> (x/y=w788:sgl)
            n391 = Bundle(w789, w788) -> (w787:cluster{sgl, sgl})  [unwired: 1 in]
            n392 = case shown="True" w791 {
              tunnel: w793 -> [_ w806]
              tunnel: w787 -> [_ w805]
              tunnel: w792 -> [_ w804]
              tunnel: [TRUE w803] -> w790
              frame False {
                # "True bc this position has\nno previous position\nto compare to"
              }
              frame True {
                # "Previous Position"
                # "New (filtered) Position"
                # "Only Check If Close to previous position\nif previous position was valid"
                # "(Y1 - Y2)^2"
                # "(X1 - X2)^2"
                n393 = Unbundle(w806) -> (w814:sgl, w816:sgl)
                n394 = Unbundle(w805) -> (w813:sgl, w815:sgl)
                n395 = Subtract(x=w813, y=w814) -> (x-y=w811:sgl)
                n396 = Subtract(x=w815, y=w816) -> (x-y=w810:sgl)
                n397 = Square(x=w811) -> (x^2=w809:sgl)
                n398 = Square(x=w810) -> (x^2=w808:sgl)
                n399 = Add(x=w809, y=w808) -> (x+y=w812:sgl)
                n400 = Square Root(x=w812) -> (sqrt(x)=w807:sgl)
                n401 = Less?(x=w807, y=w804) -> (x < y?=w803:bool)
              }
            }
          }
        }
        n402 = Replace Array Subset(array=w754, new element=w750, index=w753) -> ()  [unwired: 1 out]
        n403 = Replace Array Subset(array=w752, new element=w751, index=w753) -> ()  [unwired: 1 out]
        n404 = Replace Array Subset(array=w754, new element=w749, index=w753) -> ()  [unwired: 1 out]
        n405 = Replace Array Subset(array=w748, new element=w750, index=w765) -> (w764:dbl[])
        n406 = Replace Array Subset(array=w747, new element=w749, index=w765) -> (w763:dbl[])
        n407 = call "Wait7"("Count(mSec)"=u32 200) -> ()  [unwired: 1 out]
      }
    }
    frame Enabled {
    }
  }
  n408 = disable-structure shown="Enabled" {
    disable-tunnel: [w882 _] -> _
    disable-tunnel: ["Search Step Size\n(deg)" _] -> _
    frame Enabled {
      n409 = Multiply(x=3.413333333333333, y="Search Step Size\n(deg)") -> (x*y=w880:dbl)
      n410 = To Unsigned Word Integer(number=w880) -> (unsigned 16bit integer=w882:u16)
    }
    frame Disabled {
    }
  }
  n411 = Multiply(x="Move Servo\nThreshold (deg)", y=3.413333333333333) -> (x*y=w17:dbl)
  n412 = To Unsigned Word Integer(number=w17) -> ()  [unwired: 1 out]
  n413 = call "Tick Count8"() -> ()  [unwired: 1 out]
  n414 = flat-sequence {
    tunnel: [w886] -> w42
    tunnel: [w885] -> w41
    tunnel: [w890] -> w40
    tunnel: ["Left Servo\nID"] -> w29
    tunnel: ["Right Servo\nID"] -> w28
    tunnel: ["Compliance Slope"] -> w27
    tunnel: [w930] -> w39
    tunnel: [w929] -> w38
    tunnel: w42 -> [w928]
    tunnel: w41 -> [w927]
    tunnel: w40 -> [w926]
    tunnel: w29 -> [w924]
    tunnel: w28 -> [w923]
    tunnel: w27 -> [w922]
    tunnel: w39 -> [w1203]
    tunnel: w38 -> [w1202]
    frame #0 {
      # "BAUD RATE"
      # "Initialize UART and DIO"
      n415 = call-poly "VISA Configure Serial Port"("VISA resource name"=refnum<visa-resource-name> "ASRL1::INSTR", "Enable Termination\nChar (T)"=FALSE ("Enable Termination\nChar (T)"), "baud rate (9600)"=u32 115200) -> ("VISA resource name out"=w886:refnum<visa-resource-name>)  [unwired: 11 in, 1 out]
      n416 = call <vilib>:"Smart Open.vi"("Channel Names"=tag[] ["A/DIO2"]) -> ("DIO Ref Out"=w885:T5)  [unwired: 9 in, 1 out]
      n417 = flat-sequence {
        tunnel: w886 -> [w898]
        tunnel: w885 -> [w897]
        tunnel: "Left Servo\nID" -> [w899]
        tunnel: [w896] -> w887
        tunnel: "Compliance Slope" -> [w895]
        tunnel: "Right Servo\nID" -> [w912]
        tunnel: w887 -> [w911]
        tunnel: "Compliance Slope" -> [w910]
        tunnel: w886 -> [w909]
        tunnel: w885 -> [w908]
        frame #0 {
          w896 = 3
          n418 = while {
            tunnel: w896 -> [w905]
            tunnel: w898 -> [w903]
            tunnel: w897 -> [w902]
            tunnel: w899 -> [w901]
            tunnel: w895 -> [w900]
            i -> [w906]
            stop <- w904 stop-if-true
            n419 = call "Set_Compliance_Slope_R2.vi"("Compliance Slope"=w900, "DIO Ref Out"=w902, "VISA resource name"=w903, "Servo ID"=w901) -> ()  [unwired: 6 in, 2 out]
            n420 = Increment(x=w906) -> (x+1=w907:i32)
            n421 = Greater Or Equal?(x=w907, y=w905) -> (x >= y?=w904:bool)
          }
        }
        frame #1 {
          n422 = while {
            tunnel: w911 -> [w918]
            tunnel: w912 -> [w916]
            tunnel: w909 -> [w915]
            tunnel: w908 -> [w914]
            tunnel: w910 -> [w913]
            i -> [w919]
            stop <- w917 stop-if-true
            n423 = call "Set_Compliance_Slope_R2.vi"("Compliance Slope"=w913, "DIO Ref Out"=w914, "VISA resource name"=w915, "Servo ID"=w916) -> ()  [unwired: 6 in, 2 out]
            n424 = Increment(x=w919) -> (x+1=w920:i32)
            n425 = Greater Or Equal?(x=w920, y=w918) -> (x >= y?=w917:bool)
          }
        }
      }
      n426 = call "Tick Count"() -> ("Tick Count(uSec)"=w890:u32)
    }
    frame #1 {
      # "Service Count"
      n427 = while {
        shift-right: [w933] -> _
        shift-left: w926 -> [w950]
        tunnel: "Max Write\nTx Attempts" -> [w945]
        tunnel: "Max Read\nTx Attempts" -> [w944]
        shift-right: [w940] -> w930
        shift-left: w928 -> [w943]
        shift-right: [w939] -> w929
        shift-left: w927 -> [w942]
        tunnel: w924 -> [w938]
        tunnel: w923 -> [w937]
        tunnel: w922 -> [w936]
        shift-right: [w934] -> _
        shift-left: u16 0 -> [w935]
        stop <- "close comms" stop-if-true
        # "Loop Timer"
        n428 = local read "SERVO ENABLE"() -> (w932:bool)
        n429 = call "Tick Count2"() -> ("Tick Count(uSec)"=w933:u32)
        n430 = Subtract(x=w933, y=w950) -> (x-y=w949:u32)
        n431 = call "Wait4"("Count(mSec)"="Servo Comm\nLoop Time (ms)") -> ()  [unwired: 1 out]
        n432 = Divide(x=w949, y=u32 1000) -> (x/y=→"dT - Comm Loop":dbl)
        n433 = case shown="True" w932 {
          tunnel: w945 -> [_ w959]
          tunnel: w944 -> [_ w990]
          tunnel: w943 -> [w953 w954]
          tunnel: w942 -> [w952 w983]
          tunnel: [w953 w956] -> w940
          tunnel: [w952 w955] -> w939
          tunnel: w938 -> [_ w962]
          tunnel: w937 -> [_ w961]
          tunnel: w936 -> [_ w960]
          tunnel: w935 -> [_ w958]
          tunnel: [u16 100 w957] -> w934
          frame False {
            # "Restart at same value\nUsed to Periodically update \nCompliance Slope"
          }
          frame True {
            n434 = flat-sequence {
              tunnel: [w996] -> w994
              tunnel: [w997] -> w993
              tunnel: [w995] -> w992
              tunnel: w990 -> [w998]
              tunnel: [w1000] -> w981
              tunnel: [w999] -> w979
              tunnel: w954 -> [w1000]
              tunnel: w983 -> [w999]
              tunnel: w962 -> [w995]
              tunnel: w994 -> [w1018]
              tunnel: w993 -> [w1019]
              tunnel: w992 -> [w1017]
              tunnel: [w1017] -> w991
              tunnel: [w1016] -> w984
              tunnel: [w1015] -> w982
              tunnel: w981 -> [w1015]
              tunnel: [w1014] -> w980
              tunnel: w979 -> [w1014]
              tunnel: w991 -> [w1040]
              tunnel: w959 -> [w1039]
              tunnel: w984 -> [w1034]
              tunnel: w982 -> [w1036]
              tunnel: w980 -> [w1035]
              tunnel: [w1036] -> w977
              tunnel: [w1035] -> w975
              tunnel: [w1073] -> w978
              tunnel: w977 -> [w1073]
              tunnel: [w1072] -> w976
              tunnel: w975 -> [w1072]
              tunnel: ["Servo Comm\nWait Time - (ms)"] -> w967
              tunnel: w990 -> [w1080]
              tunnel: [w1079] -> w989
              tunnel: [w1078] -> w988
              tunnel: [w1074] -> w986
              tunnel: w978 -> [w1077]
              tunnel: w976 -> [w1076]
              tunnel: [w1077] -> w974
              tunnel: [w1076] -> w971
              tunnel: [w1075] -> w968
              tunnel: w967 -> [w1075]
              tunnel: w961 -> [w1074]
              tunnel: w989 -> [w1100]
              tunnel: w988 -> [w1099]
              tunnel: [w1098] -> w987
              tunnel: w986 -> [w1098]
              tunnel: [w1097] -> w985
              tunnel: w974 -> [w1096]
              tunnel: [w1096] -> w973
              tunnel: [w1095] -> w972
              tunnel: w971 -> [w1095]
              tunnel: w968 -> [w1094]
              tunnel: [w1094] -> w966
              tunnel: w987 -> [w1122]
              tunnel: w985 -> [w1120]
              tunnel: w959 -> [w1121]
              tunnel: w973 -> [w1119]
              tunnel: w972 -> [w1118]
              tunnel: [w1119] -> w970
              tunnel: [w1118] -> w969
              tunnel: w966 -> [w1115]
              tunnel: [w1115] -> w965
              tunnel: w970 -> [w1155]
              tunnel: w969 -> [w1154]
              tunnel: w965 -> [w1153]
              tunnel: [w1155] -> w964
              tunnel: [w1154] -> w963
              tunnel: w964 -> [w1159]
              tunnel: w963 -> [w1158]
              tunnel: w962 -> [w1164]
              tunnel: w961 -> [w1163]
              tunnel: w960 -> [w1162]
              tunnel: w958 -> [w1157]
              tunnel: w959 -> [w1161]
              tunnel: [w1160] -> w957
              tunnel: [w1159] -> w956
              tunnel: [w1158] -> w955
              frame #0 {
                n435 = while {
                  tunnel: [w1013] -> w996
                  tunnel: w995 -> [w1012]
                  tunnel: [w1005] -> w997
                  tunnel: w998 -> [w1003]
                  tunnel: w1000 -> [w1002]
                  tunnel: w999 -> [w1001]
                  i -> [w1004]
                  stop <- w1006 stop-if-true
                  # "Attemp to Read Until\nMax Read Tx Attemps Limit"
                  n436 = call "ReadServo_R3.vi"("DIO Ref In"=w1001, "VISA resource name out"=w1002, "Servo ID"=w1012) -> ("Error"=w1009:u8, "Valid Checksum"=w1010:bool, "Current Position"=w1013:u64)  [unwired: 6 in]
                  n437 = Increment(x=w1004) -> (x+1=w1007:i32)
                  n438 = Equal To 0?(x=w1009) -> (x = 0?=w1011:bool)
                  n439 = Greater Or Equal?(x=w1007, y=w1003) -> (x >= y?=w1008:bool)
                  n440 = And(x=w1010, y=w1011) -> (x .and. y?=w1005:bool)
                  n441 = Or(x=w1005, y=w1008) -> (x .or. y?=w1006:bool)
                }
              }
              frame #1 {
                # "Read Position First"
                n442 = local read "Servo Goal Position\n - Left"() -> (w1016:u16)
                n443 = case shown="True" w1019 {
                  tunnel: w1018 -> [_ w1024]
                  tunnel: w1016 -> [_ w1022]
                  frame False {
                  }
                  frame True {
                    # "Convert Received Position to Angle Relative to Robot"
                    # "45 DEG MOUNT OFFSET"
                    # "1024/300"
                    n444 = local write "Current L (10bit)"(w1024) -> ()
                    n445 = To Word Integer(number=w1024) -> (16bit integer=w1028:i16)
                    n446 = To Word Integer(number=w1022) -> (16bit integer=w1027:i16)
                    n447 = Subtract(x=w1027, y=w1028) -> (x-y=w1026:i16)
                    n448 = Divide(x=w1024, y=3.413333333333333) -> (x/y=w1032:dbl)
                    n449 = Absolute Value(x=w1026) -> (abs(x)=w1025:i16)
                    n450 = Subtract(x=w1032, y=sgl 60.0) -> (x-y=w1030:dbl)
                    n451 = Greater?(x=w1025, y=u16 5) -> (0:w1021:bool)
                    n452 = Add(x=w1030, y=sgl 45.0) -> (x+y=w1020:dbl)
                    n453 = local write "Move Servo - L"(w1021) -> ()
                    n454 = local write "Servo Moving - L"(w1021) -> ()
                    n455 = local write "Current Angle\n - Left (internal)"(w1020) -> ()
                    n456 = shared-variable "RT myRIO Target - Overlord\\Localization_Variables_r0.lvlib\\Left Servo Angle_Current"(w1020) -> ()  [unwired: 1 in, 1 out]
                  }
                }
              }
              frame #2 {
                n457 = local read "Move Servo - L"() -> (w1037:bool)
                n458 = case shown="True" w1037 {
                  tunnel: w1040 -> [_ w1055]
                  tunnel: w1034 -> [_ w1042]
                  tunnel: [TRUE w1053] -> w1038
                  tunnel: w1039 -> [_ w1045]
                  tunnel: w1036 -> [_ w1044]
                  tunnel: w1035 -> [_ w1043]
                  frame False {
                    # "Only Send if Current Position is far enough"
                  }
                  frame True {
                    w1051 = 1
                    # "High Byte"
                    # "Low Byte"
                    n459 = Type Cast(type="", x=w1042) -> (*(type *) &x=w1052:string)
                    n460 = local write "Servo Moving - L"(TRUE) -> ()
                    n461 = String Subset(string=w1052, offset (0)=1, length (rest)=w1051) -> (substring=w1047:string)
                    n462 = String Subset(string=w1052, offset (0)=0, length (rest)=w1051) -> (substring=w1046:string)
                    n463 = while {
                      tunnel: w1055 -> [w1069]
                      tunnel: [w1061] -> w1053
                      tunnel: w1047 -> [w1065]
                      tunnel: w1046 -> [w1064]
                      tunnel: w1045 -> [w1058]
                      tunnel: w1044 -> [w1057]
                      tunnel: w1043 -> [w1056]
                      i -> [w1059]
                      stop <- w1060 stop-if-true
                      # "Attemp to Write Until\nMax Write Tx Attemps Limit"
                      n464 = call "MoveServo_R3.vi"("DIO Ref Out"=w1056, "VISA resource name out"=w1057, "GP - Low Byte"=w1065, "GP - High Byte"=w1064, "Servo ID"=w1069) -> ("Valid Checksum"=w1066:bool, "Error"=w1068:u64)  [unwired: 5 in]
                      n465 = Equal To 0?(x=w1068) -> (x = 0?=w1067:bool)
                      n466 = And(x=w1066, y=w1067) -> (x .and. y?=w1061:bool)
                      n467 = Increment(x=w1059) -> (x+1=w1063:i32)
                      n468 = Greater Or Equal?(x=w1063, y=w1058) -> (x >= y?=w1062:bool)
                      n469 = Or(x=w1061, y=w1062) -> (x .or. y?=w1060:bool)
                    }
                  }
                }
                n470 = case shown="True" w1038 {
                  frame False {
                  }
                  frame True {
                    # "Update Servo flag"
                    n471 = local write "Move Servo - L"(FALSE) -> ()
                  }
                }
              }
              frame #3 {
                n472 = call "Wait2"("Count(mSec)"="Servo Comm\nWait Time - (ms)") -> ()  [unwired: 1 out]
              }
              frame #4 {
                n473 = while {
                  tunnel: [w1093] -> w1079
                  tunnel: w1074 -> [w1092]
                  tunnel: [w1085] -> w1078
                  tunnel: w1080 -> [w1083]
                  tunnel: w1077 -> [w1082]
                  tunnel: w1076 -> [w1081]
                  i -> [w1084]
                  stop <- w1086 stop-if-true
                  # "Attemp to Read Until\nMax Read Tx Attemps Limit"
                  n474 = call "ReadServo_R3.vi"("DIO Ref In"=w1081, "VISA resource name out"=w1082, "Servo ID"=w1092) -> ("Error"=w1089:u8, "Valid Checksum"=w1090:bool, "Current Position"=w1093:u64)  [unwired: 6 in]
                  n475 = Increment(x=w1084) -> (x+1=w1087:i32)
                  n476 = Equal To 0?(x=w1089) -> (x = 0?=w1091:bool)
                  n477 = Greater Or Equal?(x=w1087, y=w1083) -> (x >= y?=w1088:bool)
                  n478 = And(x=w1090, y=w1091) -> (x .and. y?=w1085:bool)
                  n479 = Or(x=w1085, y=w1088) -> (x .or. y?=w1086:bool)
                }
              }
              frame #5 {
                n480 = local read "Servo Goal Position\n - Right"() -> (w1097:u16)
                n481 = case shown="True" w1099 {
                  tunnel: w1100 -> [_ w1104]
                  tunnel: w1097 -> [_ w1103]
                  frame False {
                    # "Don't update current position"
                  }
                  frame True {
                    # "Convert Received Position to Angle Relative to Robot"
                    # "45 DEG MOUNT OFFSET"
                    # "1024/300"
                    n482 = local write "Current R (10bit)"(w1104) -> ()
                    n483 = Divide(x=w1104, y=3.413333333333333) -> (x/y=w1113:dbl)
                    n484 = Subtract(x=w1113, y=sgl 60.0) -> (x-y=w1111:dbl)
                    n485 = Subtract(x=w1111, y=sgl 45.0) -> (x-y=w1101:dbl)
                    n486 = To Word Integer(number=w1103) -> (16bit integer=w1108:i16)
                    n487 = To Word Integer(number=w1104) -> (16bit integer=w1109:i16)
                    n488 = shared-variable "RT myRIO Target - Overlord\\Localization_Variables_r0.lvlib\\Right Servo Angle_Current"(w1101) -> ()  [unwired: 1 in, 1 out]
                    n489 = local write "Current Angle\n - Right (internal)"(w1101) -> ()
                    n490 = Subtract(x=w1108, y=w1109) -> (x-y=w1107:i16)
                    n491 = Absolute Value(x=w1107) -> (abs(x)=w1106:i16)
                    n492 = Greater?(x=w1106, y=u16 5) -> (0:w1102:bool)
                    n493 = local write "Move Servo - R"(w1102) -> ()
                    n494 = local write "Servo Moving - R"(w1102) -> ()
                  }
                }
              }
              frame #6 {
                n495 = local read "Move Servo - R"() -> (w1116:bool)
                n496 = case shown="True" w1116 {
                  tunnel: w1120 -> [_ w1125]
                  tunnel: w1122 -> [_ w1132]
                  tunnel: [TRUE w1133] -> w1117
                  tunnel: w1121 -> [_ w1128]
                  tunnel: w1119 -> [_ w1127]
                  tunnel: w1118 -> [_ w1126]
                  frame False {
                  }
                  frame True {
                    w1135 = 1
                    # "High Byte"
                    # "Low Byte"
                    n497 = Type Cast(type="", x=w1125) -> (*(type *) &x=w1134:string)
                    n498 = local write "Servo Moving - R"(TRUE) -> ()
                    n499 = String Subset(string=w1134, offset (0)=1, length (rest)=w1135) -> (substring=w1131:string)
                    n500 = String Subset(string=w1134, offset (0)=0, length (rest)=w1135) -> (substring=w1130:string)
                    n501 = while {
                      tunnel: [w1144] -> w1133
                      tunnel: w1132 -> [w1149]
                      tunnel: w1131 -> [w1148]
                      tunnel: w1130 -> [w1147]
                      tunnel: w1128 -> [w1142]
                      tunnel: w1127 -> [w1140]
                      tunnel: w1126 -> [w1139]
                      i -> [w1143]
                      stop <- w1141 stop-if-true
                      # "Attemp to Write Until\nMax Write Tx Attemps Limit"
                      n502 = call "MoveServo_R3.vi"("DIO Ref Out"=w1139, "VISA resource name out"=w1140, "GP - Low Byte"=w1148, "GP - High Byte"=w1147, "Servo ID"=w1149) -> ("Valid Checksum"=w1151:bool, "Error"=w1150:u64)  [unwired: 5 in]
                      n503 = Increment(x=w1143) -> (x+1=w1145:i32)
                      n504 = Greater Or Equal?(x=w1145, y=w1142) -> (x >= y?=w1146:bool)
                      n505 = Equal To 0?(x=w1150) -> (x = 0?=w1152:bool)
                      n506 = And(x=w1151, y=w1152) -> (x .and. y?=w1144:bool)
                      n507 = Or(x=w1144, y=w1146) -> (x .or. y?=w1141:bool)
                    }
                  }
                }
                n508 = case shown="True" w1117 {
                  frame False {
                  }
                  frame True {
                    # "Update Servo flag"
                    n509 = local write "Move Servo - R"(FALSE) -> ()
                  }
                }
              }
              frame #7 {
                n510 = call "Wait3"("Count(mSec)"=w1153) -> ()  [unwired: 1 out]
              }
              frame #8 {
                # "Increment Service Count"
                # "Update Compliance Slope\nEvery x loops"
                n511 = Equal?(x=w1157, y=u16 1000) -> (x = y?=w1166:bool)
                n512 = case shown="True" w1166 {
                  tunnel: w1162 -> [_ w1176]
                  tunnel: w1159 -> [_ w1175]
                  tunnel: w1158 -> [_ w1174]
                  tunnel: w1159 -> [_ w1173]
                  tunnel: w1158 -> [_ w1172]
                  tunnel: w1164 -> [_ w1171]
                  tunnel: w1163 -> [_ w1170]
                  tunnel: w1157 -> [w1167 _]
                  tunnel: [w1167 u16 0] -> w1165
                  tunnel: w1161 -> [_ w1168]
                  frame False {
                  }
                  frame True {
                    # "Reset Service\nCount"
                    n513 = flat-sequence {
                      tunnel: w1175 -> [w1181]
                      tunnel: w1174 -> [w1180]
                      tunnel: w1171 -> [w1182]
                      tunnel: [w1178] -> w1177
                      tunnel: w1176 -> [w1179]
                      tunnel: w1168 -> [w1178]
                      tunnel: w1170 -> [w1194]
                      tunnel: w1177 -> [w1193]
                      tunnel: w1176 -> [w1192]
                      tunnel: w1173 -> [w1191]
                      tunnel: w1172 -> [w1190]
                      frame #0 {
                        n514 = while {
                          tunnel: w1178 -> [w1189]
                          tunnel: w1181 -> [w1187]
                          tunnel: w1180 -> [w1186]
                          tunnel: w1182 -> [w1185]
                          tunnel: w1179 -> [w1184]
                          i -> [w1183]
                          stop <- w1188 stop-if-true
                          n515 = call "Set_Compliance_Slope_R2.vi"("Compliance Slope"=w1184, "DIO Ref Out"=w1186, "VISA resource name"=w1187, "Servo ID"=w1185) -> ()  [unwired: 6 in, 2 out]
                          n516 = Greater Or Equal?(x=w1183, y=w1189) -> (x >= y?=w1188:bool)
                        }
                      }
                      frame #1 {
                        n517 = while {
                          tunnel: w1193 -> [w1201]
                          tunnel: w1194 -> [w1199]
                          tunnel: w1191 -> [w1198]
                          tunnel: w1190 -> [w1197]
                          tunnel: w1192 -> [w1196]
                          i -> [w1195]
                          stop <- w1200 stop-if-true
                          n518 = call "Set_Compliance_Slope_R2.vi"("Compliance Slope"=w1196, "DIO Ref Out"=w1197, "VISA resource name"=w1198, "Servo ID"=w1199) -> ()  [unwired: 6 in, 2 out]
                          n519 = Greater Or Equal?(x=w1195, y=w1201) -> (x >= y?=w1200:bool)
                        }
                      }
                    }
                  }
                }
                n520 = Increment(x=w1165) -> (x+1=w1160:u16)
              }
            }
          }
        }
      }
    }
    frame #2 {
      n521 = VISA Close(VISA resource name=w1203) -> ()  [unwired: 1 in, 1 out]
      n522 = call <vilib>:"Close.vi"("DIO Ref In"=w1202) -> ()  [unwired: 10 in, 1 out]
    }
  }
  n523 = while {
    stop <- FALSE stop-if-true
    n524 = call "Wait9"("Count(mSec)"=u32 1000) -> ()  [unwired: 1 out]
  }
  n525 = while {
    shift-right: [w1269] -> _
    shift-left: "Initial Main State - Left" -> [w1295]
    shift-right: [w1260] -> _
    shift-left: "Search Direction - in - L" -> [w1289]
    shift-right: [w1259] -> _
    shift-left: FALSE -> [w1288]
    shift-right: [w1262] -> _
    shift-left: w12 -> [w1261]
    shift-right: [w1263] -> _
    shift-left: w12 -> [w1281]
    shift-right: [w1265] -> _
    shift-left: w12 -> [w1287]
    shift-right: [w1264] -> _
    shift-left: w12 -> [w1286]
    shift-right: [w1266] -> _
    shift-left: w12 -> [w1280]
    shift-right: [w1267] -> _
    shift-left: w12 -> [w1279]
    shift-right: [w1207] -> _
    shift-left: "Search Direction - in - Right" -> [w1234]
    shift-right: [w1255] -> _
    shift-left: FALSE -> [w1232]
    shift-right: [w1256] -> _
    shift-left: w11 -> [w1221]
    shift-right: [w1208] -> _
    shift-left: w11 -> [w1220]
    shift-right: [w1209] -> _
    shift-left: w11 -> [w1229]
    shift-right: [w1210] -> _
    shift-left: w11 -> [w1226]
    shift-right: [w1211] -> _
    shift-left: w11 -> [w1231]
    shift-right: [w1212] -> _
    shift-left: w11 -> [w1230]
    shift-right: [w1219] -> _
    shift-left: "Initial Main State- Right" -> [w1246]
    shift-right: [w1251] -> _
    shift-left: 0 -> [w1253]
    shift-right: [w1216] -> _
    shift-left: 0 -> [w1238]
    shift-right: [w1250] -> _
    shift-left: "Initial Tracking State - Left" -> [w1252]
    shift-right: [w1214] -> _
    shift-left: "Initial Tracking State - Right" -> [w1244]
    shift-right: [w1215] -> _
    shift-left: "Initial Recovery State  - Right" -> [w1245]
    shift-right: [w1248] -> _
    shift-left: "Initial Recovery State - L" -> [w1249]
    stop <- FALSE stop-if-true
    w1273 = T1."Tracking" ("Next Main State")
    # "Wait for New"
    # "ADD TRACKING TIMEOUT COUNT**********************"
    # "Service Track Angle Flag"
    # "Add Logic to Have Search Directions\nopposite if Both Searching"
    # "REMOVE LAST GOAL POSITION WITH cURRENT"
    # "Go to Current State"
    # "Add Logic to Have Search Directions\nopposite if Both Searching"
    # "Manuallly Reset\nRespond Var"
    # "Manuallly Reset\nRespond Var"
    # "Update Comm Process Variables"
    # "Both Tracking"
    # "Current delta - L"
    # "delta move sum - R"
    # "delta move sum - L"
    # "Current delta - R"
    # "Service Move Respond Variables"
    n526 = local read "Min Num Frames\nper Search"() -> (w1258:i32)
    n527 = local read "Minimum Delta \nServo Threshold"() -> (w1278:i16)
    n528 = local read "Maximum Move \nServo Threshold"() -> (w1277:i16)
    n529 = local read "Middle Beacon\nCoordinates"() -> (w1222:cluster{"X":sgl, "Y":sgl})
    n530 = local read "Wait Tick Threshold"() -> (w1257:i32)
    n531 = local read "Position \nLock Status"() -> (w1285:bool)
    n532 = local read "Position \nLock Status"() -> (w1225:bool)
    n533 = local read "Search Step Size"() -> (w1276:u16)
    n534 = local read "Last Orientation"() -> (w1283:sgl)
    n535 = local read "Last Orientation"() -> (w1223:sgl)
    n536 = local read "Last Position"() -> (w1284:cluster{"X":sgl, "Y":sgl})
    n537 = local read "Last Position"() -> (w1224:cluster{"X":sgl, "Y":sgl})
    n538 = call "Wait"("Count(mSec)"="Servo Algorithm\nCycle Time(ms)") -> ()  [unwired: 1 out]
    n539 = local read "Min Num Frames\nper Search"() -> (w1228:i32)
    n540 = local read "Wait Tick Threshold"() -> (w1227:i32)
    n541 = local read "Minimum Delta \nServo Threshold"() -> (w1236:i16)
    n542 = local read "Maximum Move \nServo Threshold"() -> (w1235:i16)
    n543 = local read "Search Step Size"() -> (w1233:u16)
    n544 = local read "New Data  Flag\nRight Servo"() -> (w1241:bool)
    n545 = local read "New Data  Flag\nLeft Servo"() -> (w1247:bool)
    n546 = local read "Image Lock - Right"() -> (w1243:bool)
    n547 = local read "Image Lock - Left"() -> (w1294:bool)
    n548 = local read "Tracking Angle - Right"() -> (w1240:sgl)
    n549 = local read "Tracking Angle - Left"() -> (w1292:sgl)
    n550 = local read "Current R (10bit)"() -> (w1239:u16)
    n551 = local read "Current L (10bit)"() -> (w1291:u16)
    n552 = case shown="True" w1241 {
      tunnel: [w1323 w1364] -> w1206
      tunnel: [w1317 w1363] -> w1218
      tunnel: w1246 -> [w1318 w1362]
      tunnel: w1243 -> [_ w1361]
      tunnel: "Track Angle Valid  - R" -> [_ w1360]
      tunnel: w1240 -> [_ w1359]
      tunnel: w1239 -> [w1323 w1358]
      tunnel: "Mounting Offset - Right" -> [_ w1357]
      tunnel: w1234 -> [w1314 w1356]
      tunnel: w1232 -> [_ w1355]
      tunnel: w1229 -> [w1315 w1354]
      tunnel: w1225 -> [_ w1353]
      tunnel: w1224 -> [_ w1352]
      tunnel: w1223 -> [_ w1351]
      tunnel: w1222 -> [_ w1350]
      tunnel: w1220 -> [w1313 w1349]
      tunnel: w1231 -> [w1312 w1348]
      tunnel: w1230 -> [w1316 w1347]
      tunnel: w1236 -> [_ w1346]
      tunnel: w1235 -> [_ w1345]
      tunnel: w1233 -> [_ w1344]
      tunnel: [0 w1343] -> w1217
      tunnel: [w1318 w1342] -> w1219
      tunnel: [w1317 w1341] -> w1213
      tunnel: [w1316 w1340] -> w1212
      tunnel: [w1312 w1339] -> w1211
      tunnel: [w1315 w1338] -> w1209
      tunnel: [w1311 w1337] -> w1210
      tunnel: [w1313 w1336] -> w1208
      tunnel: w1221 -> [_ w1335]
      tunnel: [w1314 w1334] -> w1207
      tunnel: w1228 -> [_ w1333]
      tunnel: w1227 -> [_ w1332]
      tunnel: w1238 -> [w1321 w1331]
      tunnel: w1244 -> [w1320 w1330]
      tunnel: [w1321 w1329] -> w1216
      tunnel: [w1320 w1328] -> w1214
      tunnel: w1245 -> [w1319 w1327]
      tunnel: [w1319 w1326] -> w1215
      tunnel: w1226 -> [w1311 w1324]
      frame False {
        w1317 = FALSE
        # "Recovery Mode COunt"
        # "Frames Processed - L"
        # "Recovery Search move Count - L"
        # "Recovery Search Attempt Count- L"
        # "WAITING FOR NEW IMAGE, RETAIN ALL VALUES"
      }
      frame True {
        w1366 = u16 1023
        w1369 = u16 0
        # "New Tracking State"
        # "Tracking Timeout Count"
        # "Next Main State"
        # "Next Recovery State"
        # "Reset Respond"
        # "Search Direction"
        # "Recovery Count"
        # "Wait Tick Count"
        # "Recovery Search move Count"
        # "Recovery Search Attempt Count"
        # "Frames Processed"
        # "Apply Floor/Ceiling to Goal Position"
        # "Current move Delta"
        # "Service Track Angle Flag"
        # "Move Servo"
        # "Goal Position"
        # "Go to Current State"
        n553 = case shown="\"Recovery Mode\"" w1362 {
          tunnel: w1358 -> [w1388 w1465 w1647]
          tunnel: w1359 -> [_ w1467 _]
          tunnel: w1344 -> [w1387 _ w1638]
          tunnel: w1356 -> [w1386 w1447 w1632]
          tunnel: [w1385 w1463 w1646] -> w1370
          tunnel: [w1373 w1441 w1642] -> w1337
          tunnel: w1324 -> [_ _ w1643]
          tunnel: w1332 -> [_ _ w1644]
          tunnel: [w1383 w1464 w1645] -> w1363
          tunnel: w1360 -> [w1381 w1458 w1618]
          tunnel: [w1380 w1460 w1627] -> w1342
          tunnel: w1361 -> [w1379 w1459 w1617]
          tunnel: w1357 -> [_ w1468 w1640]
          tunnel: w1346 -> [_ w1466 _]
          tunnel: [w1373 w1462 w1622] -> w1343
          tunnel: w1345 -> [_ w1461 _]
          tunnel: w1354 -> [w1378 _ w1633]
          tunnel: [enum16{"Generic Sweep", "Recovery Search"}."Recovery Search" enum16{"Generic Sweep", "Recovery Search"}."Recovery Search" w1641] -> w1326
          tunnel: w1349 -> [_ _ w1637]
          tunnel: w1327 -> [_ _ w1619]
          tunnel: w1355 -> [_ w1444 w1653]
          tunnel: w1335 -> [_ w1449 w1648]
          tunnel: w1351 -> [_ w1451 w1650]
          tunnel: w1352 -> [_ w1452 w1651]
          tunnel: w1353 -> [_ w1453 w1652]
          tunnel: w1350 -> [_ w1450 w1649]
          tunnel: [FALSE w1446 w1620] -> w1341
          tunnel: w1333 -> [w1377 _ w1631]
          tunnel: [w1373 w1441 w1629] -> w1336
          tunnel: [w1373 w1441 w1636] -> w1340
          tunnel: [w1373 w1441 w1635] -> w1339
          tunnel: [w1376 w1442 w1634] -> w1338
          tunnel: w1348 -> [_ _ w1625]
          tunnel: w1347 -> [_ _ w1624]
          tunnel: [w1374 w1447 w1623] -> w1334
          tunnel: w1331 -> [_ w1457 _]
          tunnel: [w1373 w1448 w1622] -> w1329
          tunnel: w1330 -> [_ w1454 _]
          tunnel: [enum16{"Track", "Reactive Predict", ""}."Track" ("Initial Tracking State - Right") w1445 enum16{"Track", "Reactive Predict", ""}."Track" ("Initial Tracking State - Right")] -> w1328
          frame "Start Up Search", Default {
            w1373 = u16 0
            # "Search Direction"
            # "Wait for 'x' Images to be Processed\nBefore Going to Next Step"
            # "Next Main State"
            # "New Goal Position"
            # "Move Servo"
            # "Choose Next State"
            # "Frames Processed Count"
            n554 = Greater Or Equal?(x=w1378, y=w1377) -> (x >= y?=w1384:bool)
            n555 = case shown="True" w1384 {
              tunnel: w1388 -> [w1403 w1415]
              tunnel: w1387 -> [_ w1413]
              tunnel: w1386 -> [w1402 w1412]
              tunnel: [w1403 w1409] -> w1385
              tunnel: [w1401 0] -> w1376
              tunnel: [FALSE TRUE] -> w1382
              tunnel: w1378 -> [w1404 _]
              tunnel: [w1402 w1406] -> w1374
              frame False {
                # "Increase Frames\nProcessed Count"
                n556 = Increment(x=w1404) -> (x+1=w1401:i32)
              }
              frame True {
                # "Reset Frames\nProcessed Count"
                # "SWEEP SEARCH - Startup"
                # "Multiple New Step\nby Step SIze"
                # "F = CCW\nT = CW"
                # "Last Direction"
                # "Min Step"
                # "add 10 in case\nactual position\nis lower than GP"
                # "Set New Step #"
                # "Choose Direction"
                # "Nearest step"
                # "Adjust Actual Posiiton\n to pre-determiend steps"
                # "Move Servo 1 \"Step\" to\nSearch"
                n557 = Add(x=3, y=w1415) -> (x+y=w1421:i32)
                n558 = Quotient & Remainder(x=w1421, y=w1413) -> (floor(x/y)=w1419:i32)  [unwired: 1 out]
                n559 = To Byte Integer(number=w1419) -> (8bit integer=w1410:i8)
                n560 = Less?(x=w1410, y=1) -> (x < y?=w1416:bool)
                n561 = case shown="False" w1416 {
                  tunnel: w1410 -> [w1432 w1440]
                  tunnel: [w1434 FALSE] -> w1406
                  tunnel: [w1433 w1440] -> w1418
                  tunnel: w1412 -> [w1431 _]
                  tunnel: w1413 -> [w1429 _]
                  frame False {
                    # "Max Step"
                    # "# of steps\nminus 1"
                    n562 = Divide(x=1024, y=w1429) -> (x/y=w1426:dbl)
                    n563 = To Unsigned Byte Integer(number=w1426) -> (unsigned 8bit integer=w1427:u8)
                    n564 = Greater Or Equal?(x=w1432, y=w1427) -> (x >= y?=w1428:bool)
                    n565 = case shown="True" w1428 {
                      tunnel: [w1435 TRUE] -> w1434
                      tunnel: [w1436 w1437] -> w1433
                      tunnel: w1432 -> [w1436 w1437]
                      tunnel: w1431 -> [w1435 _]
                      frame False {
                        # "No Need to\nChange Direction"
                      }
                      frame True {
                        # "T"
                        # "Move CW"
                      }
                    }
                  }
                  frame True {
                    # "F"
                    # "Move CCW"
                  }
                }
                n566 = case shown="False" w1406 {
                  tunnel: w1418 -> [w1423 w1424]
                  tunnel: [w1422 w1425] -> w1414
                  frame False {
                    # "CCW\n+1"
                    n567 = Increment(x=w1423) -> (x+1=w1422:i8)
                  }
                  frame True {
                    # "CW\n-1"
                    n568 = Decrement(x=w1424) -> (x-1=w1425:i8)
                  }
                }
                n569 = Multiply(x=w1414, y=w1413) -> (x*y=w1411:u16)
                n570 = To Unsigned Word Integer(number=w1411) -> (unsigned 16bit integer=w1409:u16)
              }
            }
            n571 = case shown="False" w1381 {
              tunnel: [w1392 FALSE] -> w1383
              tunnel: w1382 -> [w1392 _]
              tunnel: [w1393 w1398] -> w1380
              tunnel: w1379 -> [_ w1396]
              frame False {
                # "Check other Servo\nStay in Startup  State"
                n572 = local read "Track Angle Valid - Left"() -> (w1389:bool)
                n573 = local read "Image Lock - Left"() -> (w1390:bool)
                n574 = Or(x=w1389, y=w1390) -> (x .or. y?=w1391:bool)
                n575 = case shown="True" w1391 {
                  tunnel: [T1."Start Up Search" ("Next Main State") T1."Recovery Mode" ("Next Main State")] -> w1393
                  frame False {
                  }
                  frame True {
                  }
                }
              }
              frame True {
                # "Override Move Servo\nCommand bc an Angle Was Found\nduring this Step"
                # "Transition to Tracking State When\nImage Processing has Locked"
                n576 = case shown="False" w1396 {
                  tunnel: [T1."Start Up Search" ("Next Main State") T1."Tracking" ("Next Main State")] -> w1398
                  frame False {
                  }
                  frame True {
                  }
                }
              }
            }
          }
          frame "Tracking" {
            w1441 = 0
            # "Frames Processed Count"
            # "Image Lock - L"
            # "Track Angle Valid"
            # "Tracking Angle"
            # "Tracking Timeout Count"
            # "Max ove delta"
            # "Move delta threshold"
            # "mount offset"
            # "Current Position"
            # "Move Respond"
            # "Trackin Timeout count"
            # "Move Servo"
            # "delta"
            # "GP"
            # "Reset Move Respond"
            # "New Tracking State"
            # "Delta Move Sum"
            # "Choose Next State"
            n577 = case shown="\"Reactive Predict\"" w1454 {
              tunnel: w1468 -> [w1486 _]
              tunnel: w1467 -> [w1485 _]
              tunnel: w1466 -> [w1484 _]
              tunnel: w1465 -> [w1483 w1541]
              tunnel: [w1482 w1539] -> w1464
              tunnel: [w1481 w1547] -> w1463
              tunnel: [w1480 0] -> w1462
              tunnel: w1461 -> [w1479 _]
              tunnel: w1459 -> [w1478 w1531]
              tunnel: w1458 -> [w1477 w1534]
              tunnel: w1457 -> [w1476 w1536]
              tunnel: w1453 -> [_ w1546]
              tunnel: w1452 -> [_ w1545]
              tunnel: w1451 -> [_ w1544]
              tunnel: w1450 -> [_ w1543]
              tunnel: w1444 -> [_ w1542]
              tunnel: w1449 -> [_ w1540]
              tunnel: [TRUE w1537] -> w1446
              tunnel: [w1473 w1535] -> w1448
              tunnel: [w1471 w1533] -> w1445
              tunnel: [0 0] -> w1442
              frame "Track", Default {
                # "Reset"
                # "Tracking Timeout"
                # "Move Delta"
                # "Goal Position"
                # "Tracking Move"
                # "Move Servo"
                # "Only Consider Tracking Angle\n\nIF\n\nImage Locked        == T\nTrack Angle Flag   == T"
                n578 = And(x=w1478, y=w1477) -> (x .and. y?=w1470:bool)
                n579 = case shown="True" w1470 {
                  tunnel: w1486 -> [_ w1492]
                  tunnel: w1485 -> [_ w1510]
                  tunnel: w1484 -> [_ w1507]
                  tunnel: w1483 -> [w1489 w1497]
                  tunnel: [w1489 w1506] -> w1481
                  tunnel: [w1491 w1505] -> w1482
                  tunnel: [w1491 w1504] -> _
                  tunnel: [u16 0 w1503] -> w1480
                  tunnel: w1479 -> [_ w1499]
                  tunnel: w1476 -> [w1488 _]
                  tunnel: [w1487 0] -> w1473
                  frame False {
                    w1491 = FALSE
                    # "Increment timeout"
                    n580 = Increment(x=w1488) -> (x+1=w1487:i32)
                  }
                  frame True {
                    # "Convert Track Angle to UINT16"
                    # "1024/300"
                    # "Move to Tracking Angle \n\nif delta is greater than move servo threshold\nAND less than max move threshold"
                    n581 = Add(x=w1510, y=w1492) -> (x+y=w1513:sgl)
                    n582 = Add(x=w1513, y=sgl 60.0) -> (x+y=w1512:sgl)
                    n583 = Multiply(x=3.413333333333333, y=w1512) -> (x*y=w1493:dbl)
                    n584 = To Word Integer(number=w1497) -> (16bit integer=w1495:i16)
                    n585 = To Unsigned Word Integer(number=w1493) -> (unsigned 16bit integer=w1509:u16)
                    n586 = To Word Integer(number=w1493) -> (16bit integer=w1508:i16)
                    n587 = Subtract(x=w1508, y=w1495) -> (x-y=w1498:i16)
                    n588 = Absolute Value(x=w1498) -> (abs(x)=w1494:i16)
                    n589 = Greater Or Equal?(x=w1494, y=w1507) -> (x >= y?=w1501:bool)
                    n590 = Less Or Equal?(x=w1494, y=w1499) -> (x <= y?=w1500:bool)
                    n591 = And(x=w1501, y=w1500) -> (x .and. y?=w1502:bool)
                    n592 = case shown="True" w1502 {
                      tunnel: w1509 -> [_ w1521]
                      tunnel: [w1516 w1521] -> w1506
                      tunnel: [w1517 w1527] -> w1505
                      tunnel: [w1517 w1527] -> w1504
                      tunnel: w1497 -> [w1516 _]
                      tunnel: w1494 -> [_ w1526]
                      tunnel: [u16 0 w1526] -> w1503
                      tunnel: w1492 -> [_ w1520]
                      frame False {
                        w1517 = FALSE
                        # "Don't Move"
                      }
                      frame True {
                        w1527 = TRUE
                        # "45 DEG MOUNT OFFSET"
                        # "1024/300"
                        # "Current Delta"
                        # "Use new Track Angle"
                        n593 = Divide(x=w1521, y=3.413333333333333) -> (x/y=w1523:dbl)
                        n594 = Negate(x=w1520) -> (-x=w1519:sgl)
                        n595 = Subtract(x=w1523, y=sgl 60.0) -> (x-y=w1525:dbl)
                        n596 = Add(x=w1525, y=w1519) -> (x+y=w1518:dbl)
                        n597 = local write "Last Track Angle - R"(w1518) -> ()
                      }
                    }
                  }
                }
                n598 = local read "Timeout to \nEnable Reactive Predict"() -> (w1474:u16)
                n599 = Less?(x=w1473, y=w1474) -> (x < y?=w1472:bool)
                n600 = case shown="False" w1472 {
                  tunnel: [enum16{"Track", "Reactive Predict", ""}."Reactive Predict" ("Initial Tracking State - Right") enum16{"Track", "Reactive Predict", ""}."Track" ("Initial Tracking State - Right")] -> w1471
                  frame False {
                  }
                  frame True {
                  }
                }
              }
              frame "Reactive Predict" {
                # "Choose New\nTracking State"
                n601 = Or(x=w1531, y=w1534) -> (x .or. y?=w1530:bool)
                n602 = case shown="False" w1530 {
                  tunnel: [w1560 w1612] -> w1547
                  tunnel: w1546 -> [w1559 _]
                  tunnel: w1545 -> [w1558 _]
                  tunnel: w1544 -> [w1557 _]
                  tunnel: w1543 -> [w1556 _]
                  tunnel: w1542 -> [w1555 _]
                  tunnel: w1540 -> [w1554 _]
                  tunnel: [w1553 w1611] -> w1539
                  tunnel: [w1552 w1611] -> w1537
                  tunnel: w1536 -> [w1551 _]
                  tunnel: [w1550 0] -> w1535
                  tunnel: [enum16{"Track", "Reactive Predict", ""}."Reactive Predict" ("Initial Tracking State - Right") enum16{"Track", "Reactive Predict", ""}."Track" ("Initial Tracking State - Right")] -> w1533
                  tunnel: w1541 -> [w1548 w1612]
                  frame False {
                    # "Stay in Reactive State"
                    # "Increment Track Timeout"
                    # "Move Respond Flag"
                    n603 = Increment(x=w1551) -> (x+1=w1550:i32)
                    n604 = case shown="True" w1555 {
                      tunnel: w1559 -> [_ w1575]
                      tunnel: w1558 -> [_ w1574]
                      tunnel: w1557 -> [_ w1573]
                      tunnel: w1556 -> [_ w1572]
                      tunnel: w1554 -> [_ w1569]
                      tunnel: [w1561 w1565] -> w1560
                      tunnel: [w1562 w1564] -> w1553
                      tunnel: [w1562 w1564] -> w1552
                      tunnel: w1548 -> [w1561 w1563]
                      frame False {
                        w1562 = FALSE
                        # "Reset Move Respond = F"
                        # "Move Servo = F"
                      }
                      frame True {
                        w1564 = TRUE
                        # "Position Lock"
                        # "Current Servo\nPosition"
                        # "Reset Move\nRespond = T"
                        # "Move Servo = T"
                        # "Apply Direction \nto Offset (delta sum)"
                        # "Check Last Known Position of Robot"
                        n605 = case shown="True" w1575 {
                          tunnel: w1574 -> [_ w1603]
                          tunnel: w1573 -> [_ w1578]
                          tunnel: w1572 -> [_ w1579]
                          tunnel: [sgl 1.0 ("y") w1577] -> w1571
                          frame False {
                            # "No Position Data Available"
                            # "Default is to move\nSame Direction as other\nServo"
                          }
                          frame True {
                            w1584 = sgl 1.0 ("y")
                            # "Use previous position/orientation to Guess Which Direction to Move Servo"
                            # "Choose Search Direction"
                            # "\"Perpendicular \nThreshold\""
                            # "If Orientation is\n ~Perpendicular -> Start Search\n in Opposite Direction of Other"
                            # "****add 90 until orientation angle is fixed"
                            # "Last Orientation"
                            # "Convert to Rad"
                            # "Avoid Divide by 0"
                            # "-1/m"
                            # "Calculate Normal Line to \nLast Robot Position\nfrom Center Beacon"
                            # "last Position \nCoordinates"
                            n606 = Unbundle(w1603) -> ("X"=w1583:sgl, "Y"=w1582:sgl)
                            n607 = Unbundle(w1579) -> ("X"=w1581:sgl, "Y"=w1580:sgl)
                            n608 = Subtract(x=w1582, y=w1580) -> (x-y=w1599:sgl)
                            n609 = Subtract(x=w1583, y=w1581) -> (x-y=w1597:sgl)
                            n610 = Equal To 0?(x=w1597) -> (x = 0?=w1598:bool)
                            n611 = case shown="False" w1598 {
                              tunnel: w1599 -> [w1606 _]
                              tunnel: w1597 -> [w1605 _]
                              tunnel: [w1604 1000000000000000.0] -> w1596
                              frame False {
                                n612 = Divide(x=w1606, y=w1605) -> (x/y=w1604:sgl)
                              }
                              frame True {
                              }
                            }
                            n613 = Equal To 0?(x=w1596) -> (x = 0?=w1601:bool)
                            n614 = case shown="False" w1601 {
                              tunnel: [w1608 1e-08] -> w1600
                              tunnel: w1596 -> [w1608 _]
                              frame False {
                              }
                              frame True {
                                # "Can't have infinit slope"
                              }
                            }
                            n615 = Divide(x=-1.0, y=w1600) -> (x/y=w1595:dbl)
                            n616 = Inverse Tangent(1:w1595) -> (0:w1593:dbl)
                            n617 = expression code="(x/pi)*180.0" "radians to degrees"(w1593) -> (w1594:dbl)
                            n618 = To Single Precision Float(number=w1594) -> (single precision float=w1591:sgl)
                            n619 = Add(x=w1578, y=sgl 90.0) -> (x+y=w1590:sgl)
                            n620 = Subtract(x=w1591, y=w1590) -> (x-y=w1589:sgl)
                            n621 = Absolute Value(x=w1589) -> (abs(x)=w1588:sgl)
                            n622 = Less Or Equal?(x=w1588, y=sgl 10.0) -> (x <= y?=w1586:bool)
                            n623 = Negate(x=w1584) -> (-x=w1585:sgl)
                            n624 = Select(t=w1585, s=w1586, f=w1584) -> (s? t:f=w1577:sgl)
                          }
                        }
                        n625 = To Word Integer(number=w1571) -> (16bit integer=w1570:i16)
                        n626 = Multiply(x=w1570, y=w1569) -> (x*y=w1568:i32)
                        n627 = To Word Integer(number=w1563) -> (16bit integer=w1567:i16)
                        n628 = Add(x=w1568, y=w1567) -> (x+y=w1566:i32)
                        n629 = To Unsigned Word Integer(number=w1566) -> (unsigned 16bit integer=w1565:u16)
                      }
                    }
                  }
                  frame True {
                    w1611 = TRUE
                    # "Go Directly to Track State"
                  }
                }
              }
            }
            n630 = local read "Tracking Timeout\nThreshold"() -> (w1455:i32)
            n631 = Less?(x=w1448, y=w1455) -> (x < y?=w1456:bool)
            n632 = case shown="False" w1456 {
              tunnel: [T1."Recovery Mode" ("Next Main State") T1."Tracking" ("Next Main State")] -> w1460
              frame False {
              }
              frame True {
              }
            }
          }
          frame "Recovery Mode" {
            w1622 = u16 0
            # "Frames Processed"
            # "Choose Next Main State"
            # "Reset recovery count"
            # "Recovery move\nCount"
            # "Recovery Search\nAttempt count"
            # "Wait Tick Timer"
            # "Move Servo = T"
            # "Service Recovery Count"
            # "delta move sum"
            # "Robot Position Valid"
            n633 = local read "Image Lock - Left"() -> (w1626:bool)
            n634 = Greater Or Equal?(x=w1643, y=w1644) -> (x >= y?=w1639:bool)
            n635 = Or(x=w1617, y=w1618) -> (x .or. y?=w1616:bool)
            n636 = case shown="\"Recovery Search\"" w1619 {
              tunnel: w1653 -> [_ _]
              tunnel: w1652 -> [_ _]
              tunnel: w1651 -> [_ _]
              tunnel: w1650 -> [_ _]
              tunnel: w1649 -> [_ _]
              tunnel: w1648 -> [_ _]
              tunnel: w1647 -> [w1688 w1774]
              tunnel: [w1680 w1772] -> w1646
              tunnel: [w1677 w1766] -> w1645
              tunnel: [FALSE FALSE] -> w1620
              tunnel: [w1682 w1763] -> w1641
              tunnel: w1637 -> [w1686 _]
              tunnel: w1640 -> [w1689 _]
              tunnel: w1639 -> [_ _]
              tunnel: w1638 -> [w1687 w1769]
              tunnel: [w1679 w1762] -> w1635
              tunnel: [w1678 w1762] -> w1636
              tunnel: w1626 -> [w1676 _]
              tunnel: [w1667 w1773] -> w1634
              tunnel: w1633 -> [w1665 w1757]
              tunnel: w1632 -> [w1670 w1770]
              tunnel: w1631 -> [w1666 w1768]
              tunnel: w1617 -> [_ _]
              tunnel: w1618 -> [_ w1765]
              tunnel: [FALSE w1764] -> w1628
              tunnel: w1625 -> [w1674 _]
              tunnel: w1624 -> [w1673 _]
              tunnel: [w1670 w1761] -> w1623
              frame "Recovery Search" {
                # "Wait for 2 Images to be Processed\nBefore Going to Next Step"
                # "Choose Next Reovery State"
                # "Recovery Search \nAttempt Count"
                # "Move Servo"
                # "Goal Position"
                # "Recovery Search\nmove Count"
                # "Attempt Recovery Search if Other Servo has Valid Angle"
                n637 = local read "Last Track Angle - L"() -> (w1669:sgl)
                n638 = Greater Or Equal?(x=w1665, y=w1666) -> (x >= y?=w1668:bool)
                n639 = case shown="True" w1668 {
                  tunnel: w1689 -> [_ w1709]
                  tunnel: [w1694 w1708] -> w1678
                  tunnel: w1688 -> [w1697 w1707]
                  tunnel: w1687 -> [_ w1706]
                  tunnel: [w1695 w1705] -> w1679
                  tunnel: [w1697 w1704] -> w1680
                  tunnel: [FALSE w1703] -> w1677
                  tunnel: w1674 -> [w1695 w1702]
                  tunnel: w1673 -> [w1694 w1701]
                  tunnel: w1676 -> [_ w1700]
                  tunnel: w1669 -> [_ w1699]
                  tunnel: [w1692 0 ("Frames Processed\nCount - in")] -> w1667
                  tunnel: w1665 -> [w1693 _]
                  frame False {
                    # "Increment Frames Processed"
                    # "WAIT"
                    n640 = Increment(x=w1693) -> (x+1=w1692:i32)
                  }
                  frame True {
                    n641 = case shown="True" w1700 {
                      tunnel: w1699 -> [_ w1722]
                      tunnel: w1702 -> [w1710 w1718]
                      tunnel: w1709 -> [_ w1723]
                      tunnel: [w1713 w1721] -> w1704
                      tunnel: [w1711 w1720] -> w1708
                      tunnel: w1701 -> [w1711 w1719]
                      tunnel: w1707 -> [w1713 w1717]
                      tunnel: w1706 -> [_ w1716]
                      tunnel: [FALSE TRUE] -> w1703
                      tunnel: [w1710 w1714] -> w1705
                      frame False {
                        # "Don't Move bc Other Servo Doesn't Have Image Lock"
                      }
                      frame True {
                        # "Move Servo = T"
                        n642 = Greater Than 0?(x=w1718) -> (x > 0?=w1724:bool)
                        n643 = case shown="True" w1724 {
                          tunnel: w1723 -> [w1731 _]
                          tunnel: w1722 -> [w1725 _]
                          tunnel: [w1730 w1741] -> w1721
                          tunnel: [w1728 w1747] -> w1720
                          tunnel: w1719 -> [w1729 w1747]
                          tunnel: w1718 -> [w1727 w1744]
                          tunnel: [w1726 w1746] -> w1714
                          tunnel: w1717 -> [_ w1742]
                          tunnel: w1716 -> [_ w1739]
                          frame False {
                            # "Increment move count to transition\nto Pan mode"
                            # "Increment Recovery Search Attempt Count"
                            # "1024/300"
                            # "Move Parallel to Other Servo"
                            n644 = Increment(x=w1729) -> (x+1=w1728:i32)
                            n645 = Add(x=w1725, y=w1731) -> (x+y=w1737:sgl)
                            n646 = Add(x=w1737, y=sgl 60.0) -> (x+y=w1736:sgl)
                            n647 = Multiply(x=3.413333333333333, y=w1736) -> (x*y=w1734:dbl)
                            n648 = Add(x=0.5, y=w1734) -> (x+y=w1732:dbl)
                            n649 = To Unsigned Word Integer(number=w1732) -> (unsigned 16bit integer=w1730:u16)
                            n650 = Increment(x=w1727) -> (x+1=w1726:i32)
                          }
                          frame True {
                            # "Apply Direction"
                            # "Step SIze"
                            # "Current Position"
                            # "Attempt to Pan in Steps Towards other Servo"
                            # "Could be same or function of \nregular search step size"
                            # "Max # of Pan\nMoves"
                            # "Pan Towards Other Servo"
                            n651 = Greater Or Equal?(x=w1744, y=u16 20) -> (x >= y?=w1745:bool)
                            n652 = case shown="False" w1745 {
                              tunnel: w1744 -> [w1755 _]
                              tunnel: [w1754 u16 0] -> w1746
                              frame False {
                                # "Increment Pan Count"
                                n653 = Increment(x=w1755) -> (x+1=w1754:i32)
                              }
                              frame True {
                                # "Reset move count"
                              }
                            }
                            n654 = local read "Recovery Search\nDirection - R"() -> (w1740:bool)
                            n655 = case shown="False" w1740 {
                              tunnel: w1742 -> [w1749 w1753]
                              tunnel: w1739 -> [w1750 w1752]
                              tunnel: [w1748 w1751] -> w1741
                              frame False {
                                # "CCW"
                                n656 = Add(x=w1749, y=w1750) -> (x+y=w1748:u16)
                              }
                              frame True {
                                # "CW"
                                n657 = Subtract(x=w1753, y=w1752) -> (x-y=w1751:u16)
                              }
                            }
                          }
                        }
                      }
                    }
                  }
                }
                n658 = local read "Max Recovery Count\n(Recovery Search)"() -> (w1671:u16)
                n659 = local read "Max Recovery\nSearch Attempts"() -> (w1672:u16)
                n660 = Less Or Equal?(x=w1678, y=w1672) -> (x <= y?=w1684:bool)
                n661 = Less Or Equal?(x=w1686, y=w1671) -> (x <= y?=w1685:bool)
                n662 = And(x=w1684, y=w1685) -> (x .and. y?=w1683:bool)
                n663 = case shown="True" w1683 {
                  tunnel: [enum16{"Generic Sweep", "Recovery Search"}."Generic Sweep" enum16{"Generic Sweep", "Recovery Search"}."Recovery Search"] -> w1682
                  frame False {
                  }
                  frame True {
                  }
                }
              }
              frame "Generic Sweep" {
                w1762 = u16 0
                # "Angle Valid?"
                # "Choose Next Recovery State"
                # "Wait for 2 Images to be Processed\nBefore Going to Next Step"
                # "New Goal Position"
                # "Move Servo"
                # "Frames Processed Count"
                n664 = Greater Or Equal?(x=w1757, y=w1768) -> (x >= y?=w1775:bool)
                n665 = case shown="True" w1775 {
                  tunnel: w1774 -> [w1791 w1803]
                  tunnel: w1769 -> [_ w1801]
                  tunnel: w1770 -> [w1790 w1800]
                  tunnel: [w1791 w1797] -> w1772
                  tunnel: [w1789 0] -> w1773
                  tunnel: [FALSE TRUE] -> w1767
                  tunnel: w1757 -> [w1792 _]
                  tunnel: [w1790 w1794] -> w1761
                  frame False {
                    # "Increment Frames Processed"
                    n666 = Increment(x=w1792) -> (x+1=w1789:i32)
                  }
                  frame True {
                    # "Reset Frames\nProcessed Count"
                    # "SWEEP SEARCH - Startup"
                    # "Multiple New Step\nby Step SIze"
                    # "F = CCW\nT = CW"
                    # "Last Direction"
                    # "Min Step"
                    # "add 10 in case\nactual position\nis lower than GP"
                    # "Set New Step #"
                    # "Choose Direction"
                    # "Nearest step"
                    # "Adjust Actual Posiiton\n to pre-determiend steps"
                    # "Move Servo 1 \"Step\" to\nSearch"
                    n667 = Add(x=5, y=w1803) -> (x+y=w1809:i32)
                    n668 = Quotient & Remainder(x=w1809, y=w1801) -> (floor(x/y)=w1807:i32)  [unwired: 1 out]
                    n669 = To Byte Integer(number=w1807) -> (8bit integer=w1798:i8)
                    n670 = Less?(x=w1798, y=1) -> (x < y?=w1804:bool)
                    n671 = case shown="False" w1804 {
                      tunnel: w1798 -> [w1820 w1828]
                      tunnel: [w1822 FALSE] -> w1794
                      tunnel: [w1821 w1828] -> w1806
                      tunnel: w1800 -> [w1819 _]
                      tunnel: w1801 -> [w1817 _]
                      frame False {
                        # "Max Step"
                        # "# of steps\nminus 1"
                        n672 = Divide(x=1024, y=w1817) -> (x/y=w1814:dbl)
                        n673 = To Unsigned Byte Integer(number=w1814) -> (unsigned 8bit integer=w1815:u8)
                        n674 = Greater Or Equal?(x=w1820, y=w1815) -> (x >= y?=w1816:bool)
                        n675 = case shown="True" w1816 {
                          tunnel: [w1823 TRUE] -> w1822
                          tunnel: [w1824 w1825] -> w1821
                          tunnel: w1820 -> [w1824 w1825]
                          tunnel: w1819 -> [w1823 _]
                          frame False {
                            # "No Need to\nChange Direction"
                          }
                          frame True {
                            # "T"
                            # "Move CW"
                          }
                        }
                      }
                      frame True {
                        # "F"
                        # "Move CCW"
                      }
                    }
                    n676 = case shown="True" w1794 {
                      tunnel: w1806 -> [w1811 w1812]
                      tunnel: [w1810 w1813] -> w1802
                      frame False {
                        # "CCW\n+1"
                        n677 = Increment(x=w1811) -> (x+1=w1810:i8)
                      }
                      frame True {
                        # "CW\n-1"
                        n678 = Decrement(x=w1812) -> (x-1=w1813:i8)
                      }
                    }
                    n679 = Multiply(x=w1802, y=w1801) -> (x*y=w1799:u16)
                    n680 = To Unsigned Word Integer(number=w1799) -> (unsigned 16bit integer=w1797:u16)
                  }
                }
                n681 = local read "Track Angle Valid - Left"() -> (w1760:bool)
                n682 = local read "Image Lock - Left"() -> (w1759:bool)
                n683 = Or(x=w1759, y=w1760) -> (x .or. y?=w1758:bool)
                n684 = case shown="True" w1765 {
                  tunnel: [w1778 w1788] -> w1766
                  tunnel: w1767 -> [w1779 _]
                  tunnel: [w1780 enum16{"Generic Sweep", "Recovery Search"}."Generic Sweep"] -> w1763
                  tunnel: [w1777 w1788] -> w1764
                  tunnel: w1758 -> [w1776 _]
                  frame False {
                    # "Is other servo tracking?"
                    n685 = case shown="True" w1776 {
                      tunnel: [enum16{"Generic Sweep", "Recovery Search"}."Generic Sweep" enum16{"Generic Sweep", "Recovery Search"}."Recovery Search"] -> w1780
                      tunnel: w1779 -> [w1783 _]
                      tunnel: [w1783 FALSE] -> w1778
                      tunnel: [FALSE TRUE] -> w1777
                      frame False {
                        # "Stay in Sweep"
                      }
                      frame True {
                        # "G o to Recovery Search  State"
                      }
                    }
                  }
                  frame True {
                    w1788 = FALSE
                    # "Override Move Servo\nCommand bc an Angle Was Found\nduring this Step"
                    # "Stay In Sweep\nLet Main State Machine transition\ninto Tracking"
                  }
                }
              }
            }
            n686 = case shown="True" w1639 {
              tunnel: [w1659 0] -> w1642
              tunnel: w1643 -> [w1661 _]
              tunnel: w1637 -> [w1660 w1663]
              tunnel: [w1660 w1662] -> w1630
              frame False {
                # "Increase Wait Tick"
                n687 = Increment(x=w1661) -> (x+1=w1659:i32)
              }
              frame True {
                # "Increment Recovery\n Mode Count"
                # "Reset Wait Tick Count"
                n688 = Increment(x=w1663) -> (x+1=w1662:i32)
              }
            }
            n689 = case shown="True" w1628 {
              tunnel: w1630 -> [w1656 _]
              tunnel: [w1656 w1657] -> w1629
              frame False {
              }
              frame True {
                n690 = local read "Max Recovery Count\n(Recovery Search)"() -> (w1658:u16)
                n691 = Decrement(x=w1658) -> (x-1=w1657:u16)
              }
            }
            n692 = case shown="False" w1616 {
              tunnel: [T1."Recovery Mode" ("Next Main State") T1."Tracking" ("Next Main State")] -> w1627
              frame False {
              }
              frame True {
              }
            }
          }
        }
        "Current Move Delta - L 2" <- w1343
        n693 = Less?(x=w1370, y=w1369) -> (x < y?=w1368:bool)
        n694 = local write "New Data  Flag\nRight Servo"(FALSE) -> ()
        n695 = Select(t=w1369, s=w1368, f=w1370) -> (s? t:f=w1365:u16)
        n696 = Greater?(x=w1365, y=w1366) -> (0:w1367:bool)
        n697 = Select(t=w1366, s=w1367, f=w1365) -> (s? t:f=w1364:u16)
      }
    }
    "Next Main State - Right" <- w1219
    "Next Tracking State - Right" <- w1214
    "Next Recovery State - Right" <- w1215
    n698 = case shown="True" w1247 {
      tunnel: [w1841 w1882] -> w1297
      tunnel: [w1835 w1881] -> w1296
      tunnel: w1295 -> [w1836 w1880]
      tunnel: w1294 -> [_ w1879]
      tunnel: "Track Angle Valid - Left" -> [_ w1878]
      tunnel: w1292 -> [_ w1877]
      tunnel: w1291 -> [w1841 w1876]
      tunnel: "Mounting Offset - Left" -> [_ w1875]
      tunnel: w1289 -> [w1831 w1874]
      tunnel: w1288 -> [_ w1873]
      tunnel: w1287 -> [w1833 w1872]
      tunnel: w1286 -> [w1832 w1871]
      tunnel: w1285 -> [_ w1870]
      tunnel: w1284 -> [_ w1869]
      tunnel: w1283 -> [_ w1868]
      tunnel: "Middle Beacon\nCoordinates" -> [_ w1867]
      tunnel: w1281 -> [w1830 w1866]
      tunnel: w1280 -> [w1829 w1865]
      tunnel: w1279 -> [w1834 w1864]
      tunnel: w1278 -> [_ w1863]
      tunnel: w1277 -> [_ w1862]
      tunnel: w1276 -> [_ w1861]
      tunnel: [0 w1860] -> w1270
      tunnel: [w1836 w1859] -> w1269
      tunnel: [w1835 w1858] -> w1268
      tunnel: [w1834 w1857] -> w1267
      tunnel: [w1829 w1856] -> w1266
      tunnel: [w1833 w1855] -> w1265
      tunnel: [w1832 w1854] -> w1264
      tunnel: [w1830 w1853] -> w1263
      tunnel: w1261 -> [_ w1852]
      tunnel: [w1831 w1851] -> w1260
      tunnel: w1258 -> [_ w1850]
      tunnel: w1257 -> [_ w1849]
      tunnel: w1253 -> [w1839 w1848]
      tunnel: w1252 -> [w1838 w1847]
      tunnel: [w1839 w1846] -> w1251
      tunnel: [w1838 w1845] -> w1250
      tunnel: w1249 -> [w1837 w1844]
      tunnel: [w1837 w1843] -> w1248
      frame False {
        w1835 = FALSE
        # "Recovery Mode COunt"
        # "Frames Processed - L"
        # "Recovery Search move Count - L"
        # "Recovery Search Attempt Count- L"
        # "WAITING FOR NEW IMAGE, RETAIN ALL VALUES"
      }
      frame True {
        w1884 = u16 1023
        w1887 = u16 0
        # "New Tracking State"
        # "Tracking Timeout Count"
        # "Next Main State"
        # "Next Recovery State"
        # "Reset Respond"
        # "Search Direction"
        # "Recovery Count"
        # "Wait Tick Count"
        # "Recovery Search move Count"
        # "Recovery Search Attempt Count"
        # "Frames Processed"
        # "Apply Floor/Ceiling to Goal Position"
        # "Current move Delta"
        # "Service Track Angle Flag"
        # "Move Servo"
        # "Goal Position"
        # "Go to Current State"
        n699 = case shown="\"Recovery Mode\"" w1880 {
          tunnel: w1876 -> [w1906 w1983 w2165]
          tunnel: w1877 -> [_ w1985 _]
          tunnel: w1861 -> [w1905 _ w2156]
          tunnel: w1874 -> [w1904 w1965 w2150]
          tunnel: [w1903 w1981 w2164] -> w1888
          tunnel: [w1891 w1959 w2160] -> w1854
          tunnel: w1871 -> [_ _ w2161]
          tunnel: w1849 -> [_ _ w2162]
          tunnel: [w1901 w1982 w2163] -> w1881
          tunnel: w1878 -> [w1899 w1976 w2136]
          tunnel: [w1898 w1978 w2145] -> w1859
          tunnel: w1879 -> [w1897 w1977 w2135]
          tunnel: w1875 -> [_ w1986 w2158]
          tunnel: w1863 -> [_ w1984 _]
          tunnel: [w1891 w1980 w2140] -> w1860
          tunnel: w1862 -> [_ w1979 _]
          tunnel: w1872 -> [w1896 _ w2151]
          tunnel: [enum16{"Generic Sweep", "Recovery Search"}."Recovery Search" enum16{"Generic Sweep", "Recovery Search"}."Recovery Search" w2159] -> w1843
          tunnel: w1866 -> [_ _ w2155]
          tunnel: w1844 -> [_ _ w2137]
          tunnel: w1873 -> [_ w1962 w2171]
          tunnel: w1852 -> [_ w1967 w2166]
          tunnel: w1868 -> [_ w1969 w2168]
          tunnel: w1869 -> [_ w1970 w2169]
          tunnel: w1870 -> [_ w1971 w2170]
          tunnel: w1867 -> [_ w1968 w2167]
          tunnel: [FALSE w1964 w2138] -> w1858
          tunnel: w1850 -> [w1895 _ w2149]
          tunnel: [w1891 w1959 w2147] -> w1853
          tunnel: [w1891 w1959 w2154] -> w1857
          tunnel: [w1891 w1959 w2153] -> w1856
          tunnel: [w1894 w1960 w2152] -> w1855
          tunnel: w1865 -> [_ _ w2143]
          tunnel: w1864 -> [_ _ w2142]
          tunnel: [w1892 w1965 w2141] -> w1851
          tunnel: w1848 -> [_ w1975 _]
          tunnel: [w1891 w1966 w2140] -> w1846
          tunnel: w1847 -> [_ w1972 _]
          tunnel: [enum16{"Track", "Reactive Predict", ""}."Track" ("Initial Tracking State - Right") w1963 enum16{"Track", "Reactive Predict", ""}."Track" ("Initial Tracking State - Right")] -> w1845
          frame "Start Up Search", Default {
            w1891 = u16 0
            # "Search Direction"
            # "Wait for 'x' Images to be Processed\nBefore Going to Next Step"
            # "Next Main State"
            # "New Goal Position"
            # "Move Servo"
            # "Choose Next State"
            # "Frames Processed Count"
            n700 = Greater Or Equal?(x=w1896, y=w1895) -> (x >= y?=w1902:bool)
            n701 = case shown="True" w1902 {
              tunnel: w1906 -> [w1921 w1933]
              tunnel: w1905 -> [_ w1931]
              tunnel: w1904 -> [w1920 w1930]
              tunnel: [w1921 w1927] -> w1903
              tunnel: [w1919 0] -> w1894
              tunnel: [FALSE TRUE] -> w1900
              tunnel: w1896 -> [w1922 _]
              tunnel: [w1920 w1924] -> w1892
              frame False {
                # "Increase Frames\nProcessed Count"
                n702 = Increment(x=w1922) -> (x+1=w1919:i32)
              }
              frame True {
                # "Reset Frames\nProcessed Count"
                # "SWEEP SEARCH - Startup"
                # "Multiple New Step\nby Step SIze"
                # "F = CCW\nT = CW"
                # "Last Direction"
                # "Min Step"
                # "add 10 in case\nactual position\nis lower than GP"
                # "Set New Step #"
                # "Choose Direction"
                # "Nearest step"
                # "Adjust Actual Posiiton\n to pre-determiend steps"
                # "Move Servo 1 \"Step\" to\nSearch"
                n703 = Add(x=3, y=w1933) -> (x+y=w1939:i32)
                n704 = Quotient & Remainder(x=w1939, y=w1931) -> (floor(x/y)=w1937:i32)  [unwired: 1 out]
                n705 = To Byte Integer(number=w1937) -> (8bit integer=w1928:i8)
                n706 = Less?(x=w1928, y=1) -> (x < y?=w1934:bool)
                n707 = case shown="False" w1934 {
                  tunnel: w1928 -> [w1950 w1958]
                  tunnel: [w1952 FALSE] -> w1924
                  tunnel: [w1951 w1958] -> w1936
                  tunnel: w1930 -> [w1949 _]
                  tunnel: w1931 -> [w1947 _]
                  frame False {
                    # "Max Step"
                    # "# of steps\nminus 1"
                    n708 = Divide(x=1024, y=w1947) -> (x/y=w1944:dbl)
                    n709 = To Unsigned Byte Integer(number=w1944) -> (unsigned 8bit integer=w1945:u8)
                    n710 = Greater Or Equal?(x=w1950, y=w1945) -> (x >= y?=w1946:bool)
                    n711 = case shown="True" w1946 {
                      tunnel: [w1953 TRUE] -> w1952
                      tunnel: [w1954 w1955] -> w1951
                      tunnel: w1950 -> [w1954 w1955]
                      tunnel: w1949 -> [w1953 _]
                      frame False {
                        # "No Need to\nChange Direction"
                      }
                      frame True {
                        # "T"
                        # "Move CW"
                      }
                    }
                  }
                  frame True {
                    # "F"
                    # "Move CCW"
                  }
                }
                n712 = case shown="False" w1924 {
                  tunnel: w1936 -> [w1941 w1942]
                  tunnel: [w1940 w1943] -> w1932
                  frame False {
                    # "CCW\n+1"
                    n713 = Increment(x=w1941) -> (x+1=w1940:i8)
                  }
                  frame True {
                    # "CW\n-1"
                    n714 = Decrement(x=w1942) -> (x-1=w1943:i8)
                  }
                }
                n715 = Multiply(x=w1932, y=w1931) -> (x*y=w1929:u16)
                n716 = To Unsigned Word Integer(number=w1929) -> (unsigned 16bit integer=w1927:u16)
              }
            }
            n717 = case shown="False" w1899 {
              tunnel: [w1910 FALSE] -> w1901
              tunnel: w1900 -> [w1910 _]
              tunnel: [w1911 w1916] -> w1898
              tunnel: w1897 -> [_ w1914]
              frame False {
                # "Check other Servo\nStay in Startup  State"
                n718 = local read "Track Angle Valid  - R"() -> (w1907:bool)
                n719 = local read "Image Lock - Right"() -> (w1908:bool)
                n720 = Or(x=w1907, y=w1908) -> (x .or. y?=w1909:bool)
                n721 = case shown="True" w1909 {
                  tunnel: [T1."Start Up Search" ("Next Main State") T1."Recovery Mode" ("Next Main State")] -> w1911
                  frame False {
                  }
                  frame True {
                  }
                }
              }
              frame True {
                # "Override Move Servo\nCommand bc an Angle Was Found\nduring this Step"
                # "Transition to Tracking State When\nImage Processing has Locked"
                n722 = case shown="False" w1914 {
                  tunnel: [T1."Start Up Search" ("Next Main State") T1."Tracking" ("Next Main State")] -> w1916
                  frame False {
                  }
                  frame True {
                  }
                }
              }
            }
          }
          frame "Tracking" {
            w1959 = 0
            # "Frames Processed Count"
            # "Image Lock - L"
            # "Track Angle Valid"
            # "Tracking Angle"
            # "Tracking Timeout Count"
            # "Max ove delta"
            # "Move delta threshold"
            # "mount offset"
            # "Current Position"
            # "Move Respond"
            # "Trackin Timeout count"
            # "Move Servo"
            # "delta"
            # "GP"
            # "Reset Move Respond"
            # "New Tracking State"
            # "Delta Move Sum"
            # "Choose Next State"
            n723 = case shown="\"Track\", Default" w1972 {
              tunnel: w1986 -> [w2004 _]
              tunnel: w1985 -> [w2003 _]
              tunnel: w1984 -> [w2002 _]
              tunnel: w1983 -> [w2001 w2059]
              tunnel: [w2000 w2057] -> w1982
              tunnel: [w1999 w2065] -> w1981
              tunnel: [w1998 0] -> w1980
              tunnel: w1979 -> [w1997 _]
              tunnel: w1977 -> [w1996 w2049]
              tunnel: w1976 -> [w1995 w2052]
              tunnel: w1975 -> [w1994 w2054]
              tunnel: w1971 -> [_ w2064]
              tunnel: w1970 -> [_ w2063]
              tunnel: w1969 -> [_ w2062]
              tunnel: w1968 -> [_ w2061]
              tunnel: w1962 -> [_ w2060]
              tunnel: w1967 -> [_ w2058]
              tunnel: [TRUE w2055] -> w1964
              tunnel: [w1991 w2053] -> w1966
              tunnel: [w1989 w2051] -> w1963
              tunnel: [0 0] -> w1960
              frame "Track", Default {
                # "Reset"
                # "Tracking Timeout"
                # "Move Delta"
                # "Goal Position"
                # "Tracking Move"
                # "Move Servo"
                # "Only Consider Tracking Angle\n\nIF\n\nImage Locked        == T\nTrack Angle Flag   == T"
                n724 = And(x=w1996, y=w1995) -> (x .and. y?=w1988:bool)
                n725 = case shown="True" w1988 {
                  tunnel: w2004 -> [_ w2010]
                  tunnel: w2003 -> [_ w2028]
                  tunnel: w2002 -> [_ w2025]
                  tunnel: w2001 -> [w2007 w2015]
                  tunnel: [w2007 w2024] -> w1999
                  tunnel: [w2009 w2023] -> w2000
                  tunnel: [w2009 w2022] -> _
                  tunnel: [u16 0 w2021] -> w1998
                  tunnel: w1997 -> [_ w2017]
                  tunnel: w1994 -> [w2006 _]
                  tunnel: [w2005 0] -> w1991
                  frame False {
                    w2009 = FALSE
                    # "Increment timeout"
                    n726 = Increment(x=w2006) -> (x+1=w2005:i32)
                  }
                  frame True {
                    # "Convert Track Angle to UINT16"
                    # "1024/300"
                    # "Move to Tracking Angle \n\nif delta is greater than move servo threshold\nAND less than max move threshold"
                    n727 = Add(x=w2028, y=w2010) -> (x+y=w2031:sgl)
                    n728 = Add(x=w2031, y=sgl 60.0) -> (x+y=w2030:sgl)
                    n729 = Multiply(x=3.413333333333333, y=w2030) -> (x*y=w2011:dbl)
                    n730 = To Word Integer(number=w2015) -> (16bit integer=w2013:i16)
                    n731 = To Unsigned Word Integer(number=w2011) -> (unsigned 16bit integer=w2027:u16)
                    n732 = To Word Integer(number=w2011) -> (16bit integer=w2026:i16)
                    n733 = Subtract(x=w2026, y=w2013) -> (x-y=w2016:i16)
                    n734 = Absolute Value(x=w2016) -> (abs(x)=w2012:i16)
                    n735 = Greater Or Equal?(x=w2012, y=w2025) -> (x >= y?=w2019:bool)
                    n736 = Less Or Equal?(x=w2012, y=w2017) -> (x <= y?=w2018:bool)
                    n737 = And(x=w2019, y=w2018) -> (x .and. y?=w2020:bool)
                    n738 = case shown="True" w2020 {
                      tunnel: w2027 -> [_ w2039]
                      tunnel: [w2034 w2039] -> w2024
                      tunnel: [w2035 w2045] -> w2023
                      tunnel: [w2035 w2045] -> w2022
                      tunnel: w2015 -> [w2034 _]
                      tunnel: w2012 -> [_ w2044]
                      tunnel: [u16 0 w2044] -> w2021
                      tunnel: w2010 -> [_ w2038]
                      frame False {
                        w2035 = FALSE
                        # "Don't Move"
                      }
                      frame True {
                        w2045 = TRUE
                        # "45 DEG MOUNT OFFSET"
                        # "1024/300"
                        # "Current Delta"
                        # "Use new Track Angle"
                        n739 = Divide(x=w2039, y=3.413333333333333) -> (x/y=w2041:dbl)
                        n740 = Negate(x=w2038) -> (-x=w2037:sgl)
                        n741 = Subtract(x=w2041, y=sgl 60.0) -> (x-y=w2043:dbl)
                        n742 = Add(x=w2043, y=w2037) -> (x+y=w2036:dbl)
                        n743 = local write "Last Track Angle - L"(w2036) -> ()
                      }
                    }
                  }
                }
                n744 = local read "Timeout to \nEnable Reactive Predict"() -> (w1992:u16)
                n745 = Less?(x=w1991, y=w1992) -> (x < y?=w1990:bool)
                n746 = case shown="False" w1990 {
                  tunnel: [enum16{"Track", "Reactive Predict", ""}."Reactive Predict" ("Initial Tracking State - Right") enum16{"Track", "Reactive Predict", ""}."Track" ("Initial Tracking State - Right")] -> w1989
                  frame False {
                  }
                  frame True {
                  }
                }
              }
              frame "Reactive Predict" {
                # "Choose New\nTracking State"
                n747 = Or(x=w2049, y=w2052) -> (x .or. y?=w2048:bool)
                n748 = case shown="False" w2048 {
                  tunnel: [w2078 w2130] -> w2065
                  tunnel: w2064 -> [w2077 _]
                  tunnel: w2063 -> [w2076 _]
                  tunnel: w2062 -> [w2075 _]
                  tunnel: w2061 -> [w2074 _]
                  tunnel: w2060 -> [w2073 _]
                  tunnel: w2058 -> [w2072 _]
                  tunnel: [w2071 w2129] -> w2057
                  tunnel: [w2070 w2129] -> w2055
                  tunnel: w2054 -> [w2069 _]
                  tunnel: [w2068 0] -> w2053
                  tunnel: [enum16{"Track", "Reactive Predict", ""}."Reactive Predict" ("Initial Tracking State - Right") enum16{"Track", "Reactive Predict", ""}."Track" ("Initial Tracking State - Right")] -> w2051
                  tunnel: w2059 -> [w2066 w2130]
                  frame False {
                    # "Stay in Reactive State"
                    # "Increment Track Timeout"
                    # "Move Respond Flag"
                    n749 = Increment(x=w2069) -> (x+1=w2068:i32)
                    n750 = case shown="True" w2073 {
                      tunnel: w2077 -> [_ w2093]
                      tunnel: w2076 -> [_ w2092]
                      tunnel: w2075 -> [_ w2091]
                      tunnel: w2074 -> [_ w2090]
                      tunnel: w2072 -> [_ w2087]
                      tunnel: [w2079 w2083] -> w2078
                      tunnel: [w2080 w2082] -> w2071
                      tunnel: [w2080 w2082] -> w2070
                      tunnel: w2066 -> [w2079 w2081]
                      frame False {
                        w2080 = FALSE
                        # "Reset Move Respond = F"
                        # "Move Servo = F"
                      }
                      frame True {
                        w2082 = TRUE
                        # "Position Lock"
                        # "Current Servo\nPosition"
                        # "Reset Move\nRespond = T"
                        # "Move Servo = T"
                        # "Apply Direction \nto Offset (delta sum)"
                        # "Check Last Known Position of Robot"
                        n751 = case shown="True" w2093 {
                          tunnel: w2092 -> [_ w2121]
                          tunnel: w2091 -> [_ w2096]
                          tunnel: w2090 -> [_ w2097]
                          tunnel: [sgl 1.0 ("y") w2095] -> w2089
                          frame False {
                            # "No Position Data Available"
                            # "Default is to move\nSame Direction as other\nServo"
                          }
                          frame True {
                            w2102 = sgl 1.0 ("y")
                            # "Use previous position/orientation to Guess Which Direction to Move Servo"
                            # "Choose Search Direction"
                            # "\"Perpendicular \nThreshold\""
                            # "If Orientation is\n ~Perpendicular -> Start Search\n in Opposite Direction of Other"
                            # "****add 90 until orientation angle is fixed"
                            # "Last Orientation"
                            # "Convert to Rad"
                            # "Avoid Divide by 0"
                            # "-1/m"
                            # "Calculate Normal Line to \nLast Robot Position\nfrom Center Beacon"
                            # "last Position \nCoordinates"
                            n752 = Unbundle(w2121) -> ("X"=w2101:sgl, "Y"=w2100:sgl)
                            n753 = Unbundle(w2097) -> ("X"=w2099:sgl, "Y"=w2098:sgl)
                            n754 = Subtract(x=w2100, y=w2098) -> (x-y=w2117:sgl)
                            n755 = Subtract(x=w2101, y=w2099) -> (x-y=w2115:sgl)
                            n756 = Equal To 0?(x=w2115) -> (x = 0?=w2116:bool)
                            n757 = case shown="False" w2116 {
                              tunnel: w2117 -> [w2124 _]
                              tunnel: w2115 -> [w2123 _]
                              tunnel: [w2122 1000000000000000.0] -> w2114
                              frame False {
                                n758 = Divide(x=w2124, y=w2123) -> (x/y=w2122:sgl)
                              }
                              frame True {
                              }
                            }
                            n759 = Equal To 0?(x=w2114) -> (x = 0?=w2119:bool)
                            n760 = case shown="False" w2119 {
                              tunnel: [w2126 1e-08] -> w2118
                              tunnel: w2114 -> [w2126 _]
                              frame False {
                              }
                              frame True {
                                # "Can't have infinit slope"
                              }
                            }
                            n761 = Divide(x=-1.0, y=w2118) -> (x/y=w2113:dbl)
                            n762 = Inverse Tangent(1:w2113) -> (0:w2111:dbl)
                            n763 = expression code="(x/pi)*180.0" "radians to degrees"(w2111) -> (w2112:dbl)
                            n764 = To Single Precision Float(number=w2112) -> (single precision float=w2109:sgl)
                            n765 = Add(x=w2096, y=sgl 90.0) -> (x+y=w2108:sgl)
                            n766 = Subtract(x=w2109, y=w2108) -> (x-y=w2107:sgl)
                            n767 = Absolute Value(x=w2107) -> (abs(x)=w2106:sgl)
                            n768 = Less Or Equal?(x=w2106, y=sgl 10.0) -> (x <= y?=w2104:bool)
                            n769 = Negate(x=w2102) -> (-x=w2103:sgl)
                            n770 = Select(t=w2103, s=w2104, f=w2102) -> (s? t:f=w2095:sgl)
                          }
                        }
                        n771 = To Word Integer(number=w2089) -> (16bit integer=w2088:i16)
                        n772 = Multiply(x=w2088, y=w2087) -> (x*y=w2086:i32)
                        n773 = To Word Integer(number=w2081) -> (16bit integer=w2085:i16)
                        n774 = Add(x=w2086, y=w2085) -> (x+y=w2084:i32)
                        n775 = To Unsigned Word Integer(number=w2084) -> (unsigned 16bit integer=w2083:u16)
                      }
                    }
                  }
                  frame True {
                    w2129 = TRUE
                    # "Go Directly to Track State"
                  }
                }
              }
            }
            n776 = local read "Tracking Timeout\nThreshold"() -> (w1973:i32)
            n777 = Less?(x=w1966, y=w1973) -> (x < y?=w1974:bool)
            n778 = case shown="False" w1974 {
              tunnel: [T1."Recovery Mode" ("Next Main State") T1."Tracking" ("Next Main State")] -> w1978
              frame False {
              }
              frame True {
              }
            }
          }
          frame "Recovery Mode" {
            w2140 = u16 0
            # "Frames Processed"
            # "Choose Next Main State"
            # "Reset recovery count"
            # "Recovery move\nCount"
            # "Recovery Search\nAttempt count"
            # "Wait Tick Timer"
            # "Move Servo = T"
            # "Service Recovery Count"
            # "delta move sum"
            # "Robot Position Valid"
            n779 = local read "Image Lock - Right"() -> (w2144:bool)
            n780 = Greater Or Equal?(x=w2161, y=w2162) -> (x >= y?=w2157:bool)
            n781 = Or(x=w2135, y=w2136) -> (x .or. y?=w2134:bool)
            n782 = case shown="\"Recovery Search\"" w2137 {
              tunnel: w2171 -> [_ _]
              tunnel: w2170 -> [_ _]
              tunnel: w2169 -> [_ _]
              tunnel: w2168 -> [_ _]
              tunnel: w2167 -> [_ _]
              tunnel: w2166 -> [_ _]
              tunnel: w2165 -> [w2206 w2292]
              tunnel: [w2198 w2290] -> w2164
              tunnel: [w2195 w2284] -> w2163
              tunnel: [FALSE FALSE] -> w2138
              tunnel: [w2200 w2281] -> w2159
              tunnel: w2155 -> [w2204 _]
              tunnel: w2158 -> [w2207 _]
              tunnel: w2157 -> [_ _]
              tunnel: w2156 -> [w2205 w2287]
              tunnel: [w2197 w2280] -> w2153
              tunnel: [w2196 w2280] -> w2154
              tunnel: w2144 -> [w2194 _]
              tunnel: [w2185 w2291] -> w2152
              tunnel: w2151 -> [w2183 w2275]
              tunnel: w2150 -> [w2188 w2288]
              tunnel: w2149 -> [w2184 w2286]
              tunnel: w2135 -> [_ _]
              tunnel: w2136 -> [_ w2283]
              tunnel: [FALSE w2282] -> w2146
              tunnel: w2143 -> [w2192 _]
              tunnel: w2142 -> [w2191 _]
              tunnel: [w2188 w2279] -> w2141
              frame "Recovery Search" {
                # "Wait for 2 Images to be Processed\nBefore Going to Next Step"
                # "Choose Next Reovery State"
                # "Recovery Search \nAttempt Count"
                # "Move Servo"
                # "Goal Position"
                # "Recovery Search\nmove Count"
                # "Attempt Recovery Search if Other Servo has Valid Angle"
                n783 = local read "Last Track Angle - R"() -> (w2187:sgl)
                n784 = Greater Or Equal?(x=w2183, y=w2184) -> (x >= y?=w2186:bool)
                n785 = case shown="True" w2186 {
                  tunnel: w2207 -> [_ w2227]
                  tunnel: [w2212 w2226] -> w2196
                  tunnel: w2206 -> [w2215 w2225]
                  tunnel: w2205 -> [_ w2224]
                  tunnel: [w2213 w2223] -> w2197
                  tunnel: [w2215 w2222] -> w2198
                  tunnel: [FALSE w2221] -> w2195
                  tunnel: w2192 -> [w2213 w2220]
                  tunnel: w2191 -> [w2212 w2219]
                  tunnel: w2194 -> [_ w2218]
                  tunnel: w2187 -> [_ w2217]
                  tunnel: [w2210 0 ("Frames Processed\nCount - in")] -> w2185
                  tunnel: w2183 -> [w2211 _]
                  frame False {
                    # "Increment Frames Processed"
                    # "WAIT"
                    n786 = Increment(x=w2211) -> (x+1=w2210:i32)
                  }
                  frame True {
                    n787 = case shown="True" w2218 {
                      tunnel: w2217 -> [_ w2240]
                      tunnel: w2220 -> [w2228 w2236]
                      tunnel: w2227 -> [_ w2241]
                      tunnel: [w2231 w2239] -> w2222
                      tunnel: [w2229 w2238] -> w2226
                      tunnel: w2219 -> [w2229 w2237]
                      tunnel: w2225 -> [w2231 w2235]
                      tunnel: w2224 -> [_ w2234]
                      tunnel: [FALSE TRUE] -> w2221
                      tunnel: [w2228 w2232] -> w2223
                      frame False {
                        # "Don't Move bc Other Servo Doesn't Have Image Lock"
                      }
                      frame True {
                        # "Move Servo = T"
                        n788 = Greater Than 0?(x=w2236) -> (x > 0?=w2242:bool)
                        n789 = case shown="False" w2242 {
                          tunnel: w2241 -> [w2249 _]
                          tunnel: w2240 -> [w2243 _]
                          tunnel: [w2248 w2259] -> w2239
                          tunnel: [w2246 w2265] -> w2238
                          tunnel: w2237 -> [w2247 w2265]
                          tunnel: w2236 -> [w2245 w2262]
                          tunnel: [w2244 w2264] -> w2232
                          tunnel: w2235 -> [_ w2260]
                          tunnel: w2234 -> [_ w2257]
                          frame False {
                            # "Increment move count to transition\nto Pan mode"
                            # "Increment Recovery Search Attempt Count"
                            # "1024/300"
                            # "Move Parallel to Other Servo"
                            n790 = Increment(x=w2247) -> (x+1=w2246:i32)
                            n791 = Add(x=w2243, y=w2249) -> (x+y=w2255:sgl)
                            n792 = Add(x=w2255, y=sgl 60.0) -> (x+y=w2254:sgl)
                            n793 = Multiply(x=3.413333333333333, y=w2254) -> (x*y=w2252:dbl)
                            n794 = Add(x=0.5, y=w2252) -> (x+y=w2250:dbl)
                            n795 = To Unsigned Word Integer(number=w2250) -> (unsigned 16bit integer=w2248:u16)
                            n796 = Increment(x=w2245) -> (x+1=w2244:i32)
                          }
                          frame True {
                            # "Apply Direction"
                            # "Step SIze"
                            # "Current Position"
                            # "Attempt to Pan in Steps Towards other Servo"
                            # "Could be same or function of \nregular search step size"
                            # "Max # of Pan\nMoves"
                            # "Pan Towards Other Servo"
                            n797 = Greater Or Equal?(x=w2262, y=u16 20) -> (x >= y?=w2263:bool)
                            n798 = case shown="False" w2263 {
                              tunnel: w2262 -> [w2273 _]
                              tunnel: [w2272 u16 0] -> w2264
                              frame False {
                                # "Increment Pan Count"
                                n799 = Increment(x=w2273) -> (x+1=w2272:i32)
                              }
                              frame True {
                                # "Reset move count"
                              }
                            }
                            n800 = local read "Recovery Search\nDirection - L"() -> (w2258:bool)
                            n801 = case shown="False" w2258 {
                              tunnel: w2260 -> [w2267 w2271]
                              tunnel: w2257 -> [w2268 w2270]
                              tunnel: [w2266 w2269] -> w2259
                              frame False {
                                # "CCW"
                                n802 = Add(x=w2267, y=w2268) -> (x+y=w2266:u16)
                              }
                              frame True {
                                # "CW"
                                n803 = Subtract(x=w2271, y=w2270) -> (x-y=w2269:u16)
                              }
                            }
                          }
                        }
                      }
                    }
                  }
                }
                n804 = local read "Max Recovery Count\n(Recovery Search)"() -> (w2189:u16)
                n805 = local read "Max Recovery\nSearch Attempts"() -> (w2190:u16)
                n806 = Less Or Equal?(x=w2196, y=w2190) -> (x <= y?=w2202:bool)
                n807 = Less Or Equal?(x=w2204, y=w2189) -> (x <= y?=w2203:bool)
                n808 = And(x=w2202, y=w2203) -> (x .and. y?=w2201:bool)
                n809 = case shown="False" w2201 {
                  tunnel: [enum16{"Generic Sweep", "Recovery Search"}."Generic Sweep" enum16{"Generic Sweep", "Recovery Search"}."Recovery Search"] -> w2200
                  frame False {
                  }
                  frame True {
                  }
                }
              }
              frame "Generic Sweep" {
                w2280 = u16 0
                # "Angle Valid?"
                # "Choose Next Recovery State"
                # "Wait for 2 Images to be Processed\nBefore Going to Next Step"
                # "New Goal Position"
                # "Move Servo"
                # "Frames Processed Count"
                n810 = Greater Or Equal?(x=w2275, y=w2286) -> (x >= y?=w2293:bool)
                n811 = case shown="True" w2293 {
                  tunnel: w2292 -> [w2309 w2321]
                  tunnel: w2287 -> [_ w2319]
                  tunnel: w2288 -> [w2308 w2318]
                  tunnel: [w2309 w2315] -> w2290
                  tunnel: [w2307 0] -> w2291
                  tunnel: [FALSE TRUE] -> w2285
                  tunnel: w2275 -> [w2310 _]
                  tunnel: [w2308 w2312] -> w2279
                  frame False {
                    # "Increment Frames Processed"
                    n812 = Increment(x=w2310) -> (x+1=w2307:i32)
                  }
                  frame True {
                    # "Reset Frames\nProcessed Count"
                    # "SWEEP SEARCH - Startup"
                    # "Multiple New Step\nby Step SIze"
                    # "F = CCW\nT = CW"
                    # "Last Direction"
                    # "Min Step"
                    # "add 10 in case\nactual position\nis lower than GP"
                    # "Set New Step #"
                    # "Choose Direction"
                    # "Nearest step"
                    # "Adjust Actual Posiiton\n to pre-determiend steps"
                    # "Move Servo 1 \"Step\" to\nSearch"
                    n813 = Add(x=5, y=w2321) -> (x+y=w2327:i32)
                    n814 = Quotient & Remainder(x=w2327, y=w2319) -> (floor(x/y)=w2325:i32)  [unwired: 1 out]
                    n815 = To Byte Integer(number=w2325) -> (8bit integer=w2316:i8)
                    n816 = Less?(x=w2316, y=1) -> (x < y?=w2322:bool)
                    n817 = case shown="False" w2322 {
                      tunnel: w2316 -> [w2338 w2346]
                      tunnel: [w2340 FALSE] -> w2312
                      tunnel: [w2339 w2346] -> w2324
                      tunnel: w2318 -> [w2337 _]
                      tunnel: w2319 -> [w2335 _]
                      frame False {
                        # "Max Step"
                        # "# of steps\nminus 1"
                        n818 = Divide(x=1024, y=w2335) -> (x/y=w2332:dbl)
                        n819 = To Unsigned Byte Integer(number=w2332) -> (unsigned 8bit integer=w2333:u8)
                        n820 = Greater Or Equal?(x=w2338, y=w2333) -> (x >= y?=w2334:bool)
                        n821 = case shown="True" w2334 {
                          tunnel: [w2341 TRUE] -> w2340
                          tunnel: [w2342 w2343] -> w2339
                          tunnel: w2338 -> [w2342 w2343]
                          tunnel: w2337 -> [w2341 _]
                          frame False {
                            # "No Need to\nChange Direction"
                          }
                          frame True {
                            # "T"
                            # "Move CW"
                          }
                        }
                      }
                      frame True {
                        # "F"
                        # "Move CCW"
                      }
                    }
                    n822 = case shown="True" w2312 {
                      tunnel: w2324 -> [w2329 w2330]
                      tunnel: [w2328 w2331] -> w2320
                      frame False {
                        # "CCW\n+1"
                        n823 = Increment(x=w2329) -> (x+1=w2328:i8)
                      }
                      frame True {
                        # "CW\n-1"
                        n824 = Decrement(x=w2330) -> (x-1=w2331:i8)
                      }
                    }
                    n825 = Multiply(x=w2320, y=w2319) -> (x*y=w2317:u16)
                    n826 = To Unsigned Word Integer(number=w2317) -> (unsigned 16bit integer=w2315:u16)
                  }
                }
                n827 = local read "Track Angle Valid  - R"() -> (w2278:bool)
                n828 = local read "Image Lock - Right"() -> (w2277:bool)
                n829 = Or(x=w2277, y=w2278) -> (x .or. y?=w2276:bool)
                n830 = case shown="False" w2283 {
                  tunnel: [w2296 w2306] -> w2284
                  tunnel: w2285 -> [w2297 _]
                  tunnel: [w2298 enum16{"Generic Sweep", "Recovery Search"}."Generic Sweep"] -> w2281
                  tunnel: [w2295 w2306] -> w2282
                  tunnel: w2276 -> [w2294 _]
                  frame False {
                    # "Is other servo tracking?"
                    n831 = case shown="True" w2294 {
                      tunnel: [enum16{"Generic Sweep", "Recovery Search"}."Generic Sweep" enum16{"Generic Sweep", "Recovery Search"}."Recovery Search"] -> w2298
                      tunnel: w2297 -> [w2301 _]
                      tunnel: [w2301 FALSE] -> w2296
                      tunnel: [FALSE TRUE] -> w2295
                      frame False {
                        # "Stay in Sweep"
                      }
                      frame True {
                        # "G o to Recovery Search  State"
                      }
                    }
                  }
                  frame True {
                    w2306 = FALSE
                    # "Override Move Servo\nCommand bc an Angle Was Found\nduring this Step"
                    # "Stay In Sweep\nLet Main State Machine transition\ninto Tracking"
                  }
                }
              }
            }
            n832 = case shown="True" w2157 {
              tunnel: [w2177 0] -> w2160
              tunnel: w2161 -> [w2179 _]
              tunnel: w2155 -> [w2178 w2181]
              tunnel: [w2178 w2180] -> w2148
              frame False {
                # "Increase Wait Tick"
                n833 = Increment(x=w2179) -> (x+1=w2177:i32)
              }
              frame True {
                # "Increment Recovery\n Mode Count"
                # "Reset Wait Tick Count"
                n834 = Increment(x=w2181) -> (x+1=w2180:i32)
              }
            }
            n835 = case shown="True" w2146 {
              tunnel: w2148 -> [w2174 _]
              tunnel: [w2174 w2175] -> w2147
              frame False {
              }
              frame True {
                n836 = local read "Max Recovery Count\n(Recovery Search)"() -> (w2176:u16)
                n837 = Decrement(x=w2176) -> (x-1=w2175:u16)
              }
            }
            n838 = case shown="False" w2134 {
              tunnel: [T1."Recovery Mode" ("Next Main State") T1."Tracking" ("Next Main State")] -> w2145
              frame False {
              }
              frame True {
              }
            }
          }
        }
        "Current Move Delta - L" <- w1860
        n839 = Less?(x=w1888, y=w1887) -> (x < y?=w1886:bool)
        n840 = local write "New Data  Flag\nLeft Servo"(FALSE) -> ()
        n841 = Select(t=w1887, s=w1886, f=w1888) -> (s? t:f=w1883:u16)
        n842 = Greater?(x=w1883, y=w1884) -> (0:w1885:bool)
        n843 = Select(t=w1884, s=w1885, f=w1883) -> (s? t:f=w1882:u16)
      }
    }
    "Next Main State - Left" <- w1269
    "Next Tracking State - Left" <- w1250
    "Next Recovery State - Left" <- w1248
    n844 = flat-sequence {
      tunnel: w1296 -> [w2353]
      tunnel: w1218 -> [w2352]
      tunnel: w1297 -> [w2355]
      tunnel: w1206 -> [w2354]
      tunnel: [w2353] -> w1310
      tunnel: [w2352] -> w1309
      tunnel: w1310 -> [w2361]
      tunnel: [w2360] -> w1305
      tunnel: [w2359] -> w1306
      tunnel: w1309 -> [w2358]
      frame #0 {
        # "Only Update GP if Moving Servo"
        n845 = case shown="True" w2353 {
          tunnel: w2355 -> [_ w2357]
          frame False {
          }
          frame True {
            # "Update Goal Position"
            n846 = local write "Servo Goal Position\n - Left"(w2357) -> ()
          }
        }
        n847 = case shown="True" w2352 {
          tunnel: w2354 -> [_ w2356]
          frame False {
          }
          frame True {
            # "New Direction"
            # "Update Goal Position"
            # "Update Direction"
            n848 = local write "Servo Goal Position\n - Right"(w2356) -> ()
          }
        }
      }
      frame #1 {
        # "Allow Comm Process to Take Down the Flag\nOnly Raise if not already in motion"
        n849 = local read "Servo Moving - R"() -> (w2366:bool)
        n850 = local read "Servo Moving - L"() -> (w2363:bool)
        n851 = local read "Move Servo - L"() -> (w2362:bool)
        n852 = local read "Move Servo - R"() -> (w2369:bool)
        n853 = Not(x=w2366) -> (.not. x?=w2368:bool)
        n854 = Not(x=w2363) -> (.not. x?=w2365:bool)
        n855 = And(x=w2358, y=w2368) -> (x .and. y?=w2367:bool)
        n856 = And(x=w2361, y=w2365) -> (x .and. y?=w2364:bool)
        n857 = case shown="True" w2367 {
          selector: w2367 -> [_ w2371]
          tunnel: [w2370 w2371] -> w2359
          tunnel: w2369 -> [w2370 _]
          frame False {
          }
          frame True {
          }
        }
        n858 = case shown="False" w2364 {
          selector: w2364 -> [_ w2373]
          tunnel: [w2372 w2373] -> w2360
          tunnel: w2362 -> [w2372 _]
          frame False {
          }
          frame True {
          }
        }
        n859 = local write "Move Servo - R"(w2359) -> ()
        n860 = local write "Move Servo - L"(w2360) -> ()
      }
    }
    n861 = local read "Current Main State - Right"() -> (w1274:T1)
    n862 = local read "Current Main State - Left"() -> (w1275:T1)
    n863 = Equal?(x=w1275, y=w1273) -> (x = y?=w1272:bool)
    n864 = Equal?(x=w1274, y=w1273) -> (x = y?=w1271:bool)
    n865 = And(x=w1272, y=w1305) -> (x .and. y?=w1301:bool)
    n866 = And(x=w1306, y=w1271) -> (x .and. y?=w1302:bool)
    n867 = And(x=w1272, y=w1271) -> (x .and. y?=w1300:bool)
    n868 = Exclusive Or(1:w1302, 2:w1301) -> (0:w1299:bool)
    n869 = case shown="True" w1299 {
      tunnel: [w2384 w2405] -> w1307
      tunnel: [w2385 w2404] -> w1303
      tunnel: w1217 -> [_ w2408]
      tunnel: w1261 -> [w2382 w2409]
      tunnel: w1221 -> [w2380 w2407]
      tunnel: [w2383 w2395] -> w1304
      tunnel: [w2381 w2394] -> w1308
      tunnel: w1270 -> [_ w2406]
      tunnel: w1300 -> [w2379 _]
      tunnel: w1301 -> [_ w2405]
      tunnel: w1302 -> [_ w2404]
      frame False {
        n870 = case shown="False" w2379 {
          tunnel: [w2389 w2391] -> w2385
          tunnel: [w2388 w2391] -> w2384
          tunnel: [w2387 w2390] -> w2383
          tunnel: w2382 -> [w2387 _]
          tunnel: [w2386 w2390] -> w2381
          tunnel: w2380 -> [w2386 _]
          frame False {
            # "No Movement\nRetain All Values"
            n871 = local read "Move Respond - L"() -> (w2389:bool)
            n872 = local read "Move Respond - R"() -> (w2388:bool)
          }
          frame True {
            w2390 = i16 0
            w2391 = FALSE
            # "Reset Delta Move sum\nfor both"
            # "F"
            # "Both Moved,\nMake Flags False"
          }
        }
      }
      frame True {
        w2401 = 200 ("y")
        w2392 = -200 ("y")
        # "Add/Clear Sum for \nServo That didn't move"
        # "Update Moving Servo's  Delta Position"
        # "if one Servo Moves, other should \nmove too eventually,\nUsed in Search Process"
        # "Only 1 Servo is Moving Due to Tracking --> Update delta move sum"
        n873 = case shown="True" w2404 {
          tunnel: w2409 -> [_ w2417]
          tunnel: w2408 -> [_ w2416]
          tunnel: [i16 0 w2415] -> w2402
          frame False {
          }
          frame True {
            n874 = Add(x=w2417, y=w2416) -> (x+y=w2415:i32)
          }
        }
        n875 = case shown="True" w2405 {
          tunnel: w2407 -> [_ w2413]
          tunnel: w2406 -> [_ w2412]
          tunnel: [i16 0 w2411] -> w2399
          frame False {
          }
          frame True {
            n876 = Add(x=w2413, y=w2412) -> (x+y=w2411:i32)
          }
        }
        n877 = Greater?(x=w2402, y=w2401) -> (0:w2403:bool)
        n878 = Greater?(x=w2399, y=w2401) -> (0:w2400:bool)
        n879 = Select(t=w2401, s=w2400, f=w2399) -> (s? t:f=w2396:i32)
        n880 = Select(t=w2401, s=w2403, f=w2402) -> (s? t:f=w2397:i32)
        n881 = Greater?(x=w2397, y=w2392) -> (0:w2393:bool)
        n882 = Greater?(x=w2396, y=w2392) -> (0:w2398:bool)
        n883 = Select(t=w2396, s=w2398, f=w2392) -> (s? t:f=w2394:i32)
        n884 = Select(t=w2397, s=w2393, f=w2392) -> (s? t:f=w2395:i32)
      }
    }
    n885 = case shown="True" w1213 {
      selector: w1213 -> [_ w2351]
      tunnel: [w2348 w2350] -> w1255
      tunnel: [w2347 i16 0] -> w1256
      tunnel: w1307 -> [w2348 _]
      tunnel: w1308 -> [w2347 _]
      frame False {
      }
      frame True {
        n886 = Not(x=w2351) -> (.not. x?=w2350:bool)
      }
    }
    "Move Respond - R" <- w1255
    "deltaMoveServo\n- R" <- w1256
    n887 = case shown="False" w1268 {
      selector: w1268 -> [_ w2378]
      tunnel: [w2375 w2377] -> w1259
      tunnel: [w2374 i16 0] -> w1262
      tunnel: w1303 -> [w2375 _]
      tunnel: w1304 -> [w2374 _]
      frame False {
      }
      frame True {
        n888 = Not(x=w2378) -> (.not. x?=w2377:bool)
      }
    }
    "Move Respond - L" <- w1259
    "deltaMoveServo\n- L" <- w1262
    "Current Main State - Left" <- w1295
    "Frames Processed\nCount - in -L" <- w1287
    "Wait Tick Count - in - L" <- w1286
    "Recovery Mode Count - in Left" <- w1281
    "Recovery Search\nmove Count - in - L" <- w1280
    "Recovery Search\nAttempt Count - in - L" <- w1279
    "Current Main State - Right" <- w1246
    "Frames Processed\nCount - in Right" <- w1229
    "Recovery Search\nmove Count - Right" <- w1231
    "Recovery Search\nAttempt Count - Right" <- w1230
    "Wait Tick Count - Right" <- w1226
    "Recovery Mode Count in Right" <- w1220
    "Tracking Timeout\nCount - L" <- w1253
    "Tracking Timeout\nCount - R" <- w1238
    "Current Tracking State - Left" <- w1252
    "Current Tracking State - Right 2" <- w1244
    "Current Recovery State - Right" <- w1245
    "Current Recovery State -L" <- w1249
  }
